vi "CRYUnflatten Analysis.vi"(11 "Unflatten Analysis":string) -> (0 "Error?":bool, 2 "Analysis":T1={"Name"="", "Harmonics"=[1.0], " Algorithm"=0, "delay"=0.0, "THD(%)"=FALSE, "Rub&Buzz"=FALSE, "Imp"=FALSE, "Imp Ref resistor"=1.0, "Y data"=0, "Y prefix"="", "Y unit"="", "Y dB ref"=1.0, "Custom Curve Names"=[], "har list items"=[""], "Envelope"=FALSE, "use custom unit"=FALSE, "autodelay ch"=0.0, "impulse"=FALSE, " start ms"=1.0, " stop ms"=1.0, "Scaling"=1, "Default Overlap "=FALSE, "Advanced View"=FALSE, "Loose Particle"=FALSE, "Use default"=FALSE, "Auto-Correlation(Stimulus)"=FALSE, "Auto-Correlation(Response)"=FALSE, "Deconvolved Response"=FALSE, "Mic Current"=FALSE, "M List Vaiues"=0, "Type"=0, "Delay Method"=3, "Apply Correction Out"=FALSE, "Apply Correction In"=FALSE, "Harmonics @ meas.frq"=FALSE, "THD Normalized(%)"=FALSE, "Total Distortion"=FALSE, "THD+Noise(%)"=FALSE, "Rub&Buzz Norm'd(%)"=FALSE, "Standard Error"=FALSE, "Confidence Limits"=FALSE, "Total Diff"=FALSE, "Total Noise"=FALSE, "Total DFD(%)"=FALSE, "Total IMD(%)"=FALSE, "Total IM"=FALSE, "Total DFD+Noise(%)"=FALSE, "Use Channel Name"=FALSE, "Waveform In"="", "Waveform Out"="", "Method"=3, "Spectral Scaling"=3, "Appliied Unit"=1, "Length Unit"=1, "Applied Units"=1, "Sens Item"=0, "Tab"=1, "Distance Unit"=0, "discard cycles"=1.0, "Weigting"="", "Averaging Time"=0.0, "Max duration"=0.0, "Min duration"=0.0, "Attack Threshold"=0.0, "Hysteresis Up"=0.0, "Fmin(Hz)"=0.0, "Fmax(Hz)"=0.0, "Freq.Resolution"=0.0, "Over-samples Res."=0.0, "Win Resolution"=0.0, "distance"=0.0, "samples"=1.0, "Overlap"=1.0, "Record Length"=1.0, "No.of FFTs"=0.0, "Hz"=1.0, "record delay"=1.0, " Std Err"=1.0, "Response"=FALSE, "Coherent Power*"=FALSE, "Stimulus"=FALSE, "Measurement Confidence"=FALSE, "Auto Spectrum(Response)*"=FALSE, "Auto Spectrum(Stimulus)*"=FALSE, "Cross Spectrum*"=FALSE, "functions"=FALSE, "Frequency Response"=FALSE, "Non-Coherent Power*"=FALSE, "Coherence (%)"=FALSE, "Non-Coherence (%)"=FALSE, "Signal-Noise Ratio (dB)"=FALSE, "Non-Coherenct Distirtion*"=FALSE, "Result Waveforms"=FALSE, "Coupling"=FALSE, "Averaging"=0, "Harmonics"=0, "Custom Curve Names"=0, "unLabel"="", "Custom Curve Names"="", "Unit"="", "Total IMD + Noise(%) "=FALSE, "ResponseMe"=1, "Intermod"=[1.0], "Diff\n"=[1.0], "Cross-Correlation"=FALSE, "IM list items"=[""], "Diff list items"=[""], "TSR Window Type"="", "Help"="", "Custom Curve IDs"=[], "Default Curve Names"=[], "Loose Particle waveform"=FALSE, "Perceptual Rub&Buzz"=FALSE, "Imp Auto Mode"=0, "Mic Auto Mode"=0, "Mic Ref resistor"=1.0, "Curve Resolution"=3, "Curve Resolution Hz"=0.0, "Polarity"=FALSE} {"Curve Resolution Hz" format="%.2f"; "Mic Ref resistor" format="%.2f"; "Diff" format="%.2f"; "Intermod" format="%.2f"; "ResponseMe" items=["Absolute", "Relative"]; "Std Err" format="%.1f"; "record delay" format="%.1f"; "Hz" format="%.1f"; "No.of FFTs" format="%.2f"; "Record Length" format="%.1f"; "Overlap" format="%.1f"; "samples" format="%.1f"; "distance" format="%.2f"; "Win Resolution" format="%.2f"; "Over-samples Res." format="%.2f"; "Freq.Resolution" format="%.2f"; "Fmax(Hz)" format="%.2f"; "Fmin(Hz)" format="%.2f"; "Hysteresis Up" format="%.2f"; "Attack Threshold" format="%.2f"; "Min duration" format="%.2f"; "Max duration" format="%.2f"; "Averaging Time" format="%.2f"; "Distance Unit" items=["Absolute", "Relative"]; "Sens Item" items=["x", "y", "z"]; "Applied Units" items=["Absolute", "Relative"]; "Length Unit" items=["Absolute", "Relative"]; "Appliied Unit" items=["Absolute", "Relative"]; "Spectral Scaling" items=["Absolute", "Relative"]; "M List Vaiues" items=["x", "y", "z"]; "Scaling" format="%.1f"; "stop ms" format="%.1f"; "start ms" format="%.1f"; "Y data" items=["dB", "Lin"]; "Y dB ref" format="%.1f"; "Imp Ref resistor" format="%.2f"; "Harmonics" format="%.2f"; "delay" format="%.2f"}, 3 "Header info":T2={"Data type"="Data            ", "Version"=1, "Dimensions"=0})   [LabVIEW 2013]
uses:
  Typedef Control/CRYAnalysis Cluster.ctl
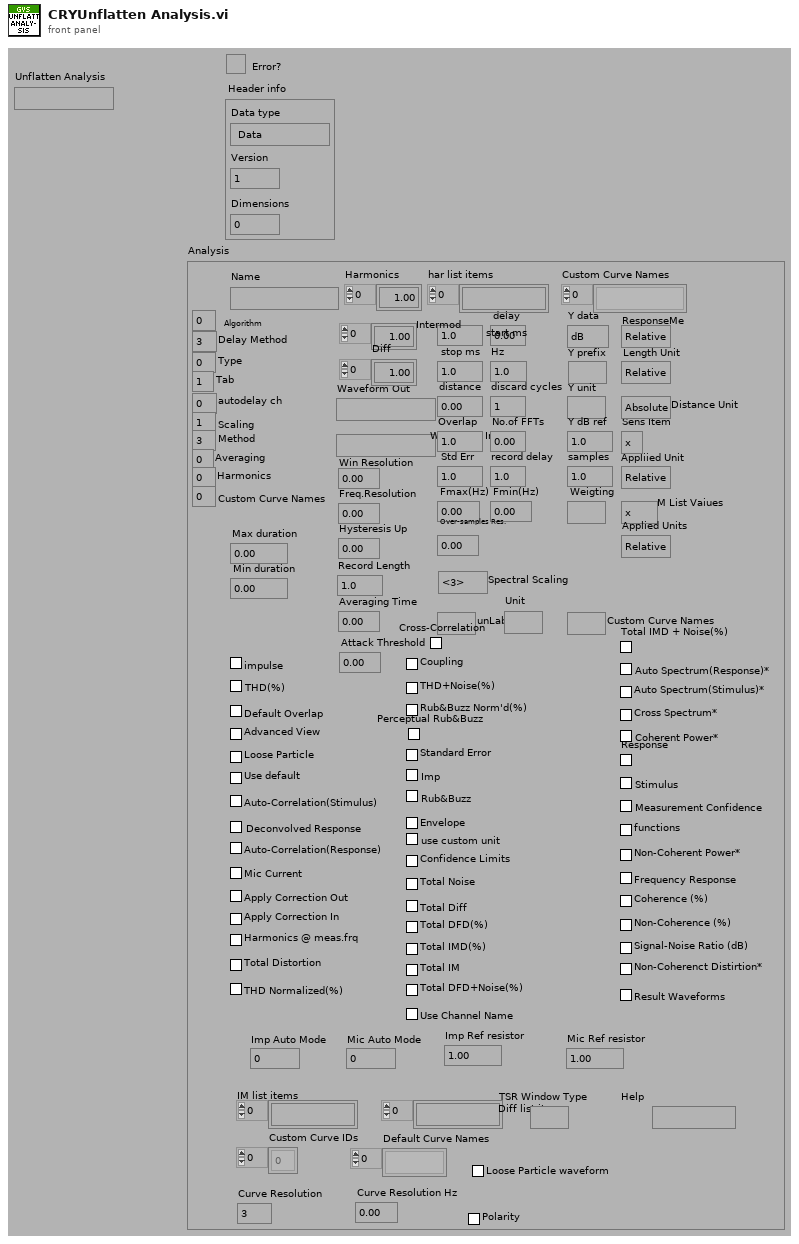
[diagram p1: front panel]
types:
  T1 = typedef "CRYAnalysis Cluster.ctl" = cluster{"Name":string, "Harmonics":dbl[], " Algorithm":u16, "delay":dbl, "THD(%)":bool, "Rub&Buzz":bool, "Imp":bool, "Imp Ref resistor":dbl, "Y data":u16, "Y prefix":string, "Y unit":string, "Y dB ref":dbl, "Custom Curve Names":string[], "har list items":string[], "Envelope":bool, "use custom unit":bool, "autodelay ch":dbl, "impulse":bool, " start ms":dbl, " stop ms":dbl, "Scaling":i32, "Default Overlap ":bool, "Advanced View":bool, "Loose Particle":bool, "Use default":bool, "Auto-Correlation(Stimulus)":bool, "Auto-Correlation(Response)":bool, "Deconvolved Response":bool, "Mic Current":bool, "M List Vaiues":u16, "Type":u16, "Delay Method":u16, "Apply Correction Out":bool, "Apply Correction In":bool, "Harmonics @ meas.frq":bool, "THD Normalized(%)":bool, "Total Distortion":bool, "THD+Noise(%)":bool, "Rub&Buzz Norm'd(%)":bool, "Standard Error":bool, "Confidence Limits":bool, "Total Diff":bool, "Total Noise":bool, "Total DFD(%)":bool, "Total IMD(%)":bool, "Total IM":bool, "Total DFD+Noise(%)":bool, "Use Channel Name":bool, "Waveform In":string, "Waveform Out":string, "Method":u16, "Spectral Scaling":u16, "Appliied Unit":u16, "Length Unit":u16, "Applied Units":u16, "Sens Item":u16, "Tab":i32, "Distance Unit":u16, "discard cycles":dbl, "Weigting":string, "Averaging Time":dbl, "Max duration":dbl, "Min duration":dbl, "Attack Threshold":dbl, "Hysteresis Up":dbl, "Fmin(Hz)":dbl, "Fmax(Hz)":dbl, "Freq.Resolution":dbl, "Over-samples Res.":dbl, "Win Resolution":dbl, "distance":dbl, "samples":dbl, "Overlap":dbl, "Record Length":dbl, "No.of FFTs":dbl, "Hz":dbl, "record delay":dbl, " Std Err":dbl, "Response":bool, "Coherent Power*":bool, "Stimulus":bool, "Measurement Confidence":bool, "Auto Spectrum(Response)*":bool, "Auto Spectrum(Stimulus)*":bool, "Cross Spectrum*":bool, "functions":bool, "Frequency Response":bool, "Non-Coherent Power*":bool, "Coherence (%)":bool, "Non-Coherence (%)":bool, "Signal-Noise Ratio (dB)":bool, "Non-Coherenct Distirtion*":bool, "Result Waveforms":bool, "Coupling":bool, "Averaging":u16, "Harmonics":i32, "Custom Curve Names":i32, "unLabel":string, "Custom Curve Names":string, "Unit":string, "Total IMD + Noise(%) ":bool, "ResponseMe":u16, "Intermod":dbl[], "Diff\n":dbl[], "Cross-Correlation":bool, "IM list items":string[], "Diff list items":string[], "TSR Window Type":string, "Help":string, "Custom Curve IDs":i32[], "Default Curve Names":string[], "Loose Particle waveform":bool, "Perceptual Rub&Buzz":bool, "Imp Auto Mode":u16, "Mic Auto Mode":u16, "Mic Ref resistor":dbl, "Curve Resolution":u16, "Curve Resolution Hz":dbl, "Polarity":bool}
  T2 = cluster{"Data type":string, "Version":u16, "Dimensions":u8}
  T3 = cluster{"Name":string, "Harmonics":dbl[], " Algorithm":u16, "delay":dbl, "THD(%)":bool, "Rub&Buzz":bool, "Imp":bool, "Imp Ref resistor":dbl, "Y data":u16, "Y prefix":string, "Y unit":string, "Y dB ref":dbl, "Custom Curve Names":string[], "har list items":string[], "Envelope":bool, "use custom unit":bool, "autodelay ch":dbl, "impulse":bool, " start ms":dbl, " stop ms":dbl, "Scaling":i32, "Default Overlap ":bool, "Advanced View":bool, "Loose Particle":bool, "Use default":bool, "Auto-Correlation(Stimulus)":bool, "Auto-Correlation(Response)":bool, "Deconvolved Response":bool, "Mic Current":bool, "M List Vaiues":u16, "Type":u16, "Delay Method":u16, "Apply Correction Out":bool, "Apply Correction In":bool, "Harmonics @ meas.frq":bool, "THD Normalized(%)":bool, "Total Distortion":bool, "THD+Noise(%)":bool, "Rub&Buzz Norm'd(%)":bool, "Standard Error":bool, "Confidence Limits":bool, "Total Diff":bool, "Total Noise":bool, "Total DFD(%)":bool, "Total IMD(%)":bool, "Total IM":bool, "Total DFD+Noise(%)":bool, "Use Channel Name":bool, "Waveform In":string, "Waveform Out":string, "Method":u16, "Spectral Scaling":u16, "Appliied Unit":u16, "Length Unit":u16, "Applied Units":u16, "Sens Item":u16, "Tab":i32, "Distance Unit":u16, "discard cycles":dbl, "Weigting":string, "Averaging Time":dbl, "Max duration":dbl, "Min duration":dbl, "Attack Threshold":dbl, "Hysteresis Up":dbl, "Fmin(Hz)":dbl, "Fmax(Hz)":dbl, "Freq.Resolution":dbl, "Over-samples Res.":dbl, "Win Resolution":dbl, "distance":dbl, "samples":dbl, "Overlap":dbl, "Record Length":dbl, "No.of FFTs":dbl, "Hz":dbl, "record delay":dbl, " Std Err":dbl, "Response":bool, "Coherent Power*":bool, "Stimulus":bool, "Measurement Confidence":bool, "Auto Spectrum(Response)*":bool, "Auto Spectrum(Stimulus)*":bool, "Cross Spectrum*":bool, "functions":bool, "Frequency Response":bool, "Non-Coherent Power*":bool, "Coherence (%)":bool, "Non-Coherence (%)":bool, "Signal-Noise Ratio (dB)":bool, "Non-Coherenct Distirtion*":bool, "Result Waveforms":bool, "Coupling":bool, "Averaging":u16, "Harmonics":i32, "Custom Curve Names":i32, "unLabel":string, "Custom Curve Names":string, "Unit":string, "Total IMD + Noise(%) ":bool, "ResponseMe":u16, "Intermod":dbl[], "Diff\n":dbl[], "Cross-Correlation":bool, "IM list items":string[], "Diff list items":string[], "TSR Window Type":string, "Help":string, "Custom Curve IDs":i32[], "Default Curve Names":string[], "Loose Particle waveform":bool, "Perceptual Rub&Buzz":bool, "Imp Auto Mode":u16, "Mic Auto Mode":u16, "Mic Ref resistor":dbl, "Curve Resolution":u16, "Curve Resolution Hz":dbl, "Polarity":bool}
  T4 = cluster{"Name":string, "Harmonics":dbl[], " Algorithm":u16, "delay":dbl, "THD(%)":bool, "Rub&Buzz":bool, "Imp":bool, "Imp Ref resistor":dbl, "Y data":u16, "Y prefix":string, "Y unit":string, "Y dB ref":dbl, "Custom Curve Names":string[], "har list items":string[], "Envelope":bool, "use custom unit":bool, "autodelay ch":dbl, "impulse":bool, " start ms":dbl, " stop ms":dbl, "Scaling":i32, "Default Overlap ":bool, "Advanced View":bool, "Loose Particle":bool, "Use default":bool, "Auto-Correlation(Stimulus)":bool, "Auto-Correlation(Response)":bool, "Deconvolved Response":bool, "Mic Current":bool, "M List Vaiues":u16, "Type":u16, "Delay Method":u16, "Apply Correction Out":bool, "Apply Correction In":bool, "Harmonics @ meas.frq":bool, "THD Normalized(%)":bool, "Total Distortion":bool, "THD+Noise(%)":bool, "Rub&Buzz Norm'd(%)":bool, "Standard Error":bool, "Confidence Limits":bool, "Total Diff":bool, "Total Noise":bool, "Total DFD(%)":bool, "Total IMD(%)":bool, "Total IM":bool, "Total DFD+Noise(%)":bool, "Use Channel Name":bool, "Waveform In":string, "Waveform Out":string, "Method":u16, "Spectral Scaling":u16, "Appliied Unit":u16, "Length Unit":u16, "Applied Units":u16, "Sens Item":u16, "Tab":i32, "Distance Unit":u16, "discard cycles":dbl, "Weigting":string, "Averaging Time":dbl, "Max duration":dbl, "Min duration":dbl, "Attack Threshold":dbl, "Hysteresis Up":dbl, "Fmin(Hz)":dbl, "Fmax(Hz)":dbl, "Freq.Resolution":dbl, "Over-samples Res.":dbl, "Win Resolution":dbl, "distance":dbl, "samples":dbl, "Overlap":dbl, "Record Length":dbl, "No.of FFTs":dbl, "Hz":dbl, "record delay":dbl, " Std Err":dbl, "Response":bool, "Coherent Power*":bool, "Stimulus":bool, "Measurement Confidence":bool, "Auto Spectrum(Response)*":bool, "Auto Spectrum(Stimulus)*":bool, "Cross Spectrum*":bool, "functions":bool, "Frequency Response":bool, "Non-Coherent Power*":bool, "Coherence (%)":bool, "Non-Coherence (%)":bool, "Signal-Noise Ratio (dB)":bool, "Non-Coherenct Distirtion*":bool, "Result Waveforms":bool, "Coupling":bool, "Averaging":u16, "Harmonics":i32, "Custom Curve Names":i32, "unLabel":string, "Custom Curve Names":string, "Unit":string, "Total IMD + Noise(%) ":bool, "ResponseMe":u16, "Intermod":dbl[], "Diff\n":dbl[], "Cross-Correlation":bool, "IM list items":string[], "Diff list items":string[], "TSR Window Type":string, "Help":string, "Custom Curve IDs":i32[], "Default Curve Names":string[], "Loose Particle waveform":bool, "Perceptual Rub&Buzz":bool, "Imp Auto Mode":u16, "Mic Auto Mode":u16, "Mic Ref resistor":dbl, "Curve Resolution":u16, "Curve Resolution Hz":dbl}
  T5 = cluster{"Name":string, "Harmonics":dbl[], " Algorithm":u16, "delay":dbl, "THD(%)":bool, "Rub&Buzz":bool, "Imp":bool, "Imp Ref resistor":dbl, "Y data":u16, "Y prefix":string, "Y unit":string, "Y dB ref":dbl, "Custom Curve Names":string[], "har list items":string[], "Envelope":bool, "use custom unit":bool, "autodelay ch":dbl, "impulse":bool, " start ms":dbl, " stop ms":dbl, "Scaling":i32, "Default Overlap ":bool, "Advanced View":bool, "Loose Particle":bool, "Use default":bool, "Auto-Correlation(Stimulus)":bool, "Auto-Correlation(Response)":bool, "Deconvolved Response":bool, "Mic Current":bool, "M List Vaiues":u16, "Type":u16, "Delay Method":u16, "Apply Correction Out":bool, "Apply Correction In":bool, "Harmonics @ meas.frq":bool, "THD Normalized(%)":bool, "Total Distortion":bool, "THD+Noise(%)":bool, "Rub&Buzz Norm'd(%)":bool, "Standard Error":bool, "Confidence Limits":bool, "Total Diff":bool, "Total Noise":bool, "Total DFD(%)":bool, "Total IMD(%)":bool, "Total IM":bool, "Total DFD+Noise(%)":bool, "Use Channel Name":bool, "Waveform In":string, "Waveform Out":string, "Method":u16, "Spectral Scaling":u16, "Appliied Unit":u16, "Length Unit":u16, "Applied Units":u16, "Sens Item":u16, "Tab":i32, "Distance Unit":u16, "discard cycles":dbl, "Weigting":string, "Averaging Time":dbl, "Max duration":dbl, "Min duration":dbl, "Attack Threshold":dbl, "Hysteresis Up":dbl, "Fmin(Hz)":dbl, "Fmax(Hz)":dbl, "Freq.Resolution":dbl, "Over-samples Res.":dbl, "Win Resolution":dbl, "distance":dbl, "samples":dbl, "Overlap":dbl, "Record Length":dbl, "No.of FFTs":dbl, "Hz":dbl, "record delay":dbl, " Std Err":dbl, "Response":bool, "Coherent Power*":bool, "Stimulus":bool, "Measurement Confidence":bool, "Auto Spectrum(Response)*":bool, "Auto Spectrum(Stimulus)*":bool, "Cross Spectrum*":bool, "functions":bool, "Frequency Response":bool, "Non-Coherent Power*":bool, "Coherence (%)":bool, "Non-Coherence (%)":bool, "Signal-Noise Ratio (dB)":bool, "Non-Coherenct Distirtion*":bool, "Result Waveforms":bool, "Coupling":bool, "Averaging":u16, "Harmonics":i32, "Custom Curve Names":i32, "unLabel":string, "Custom Curve Names":string, "Unit":string, "Total IMD + Noise(%) ":bool, "ResponseMe":u16, "Intermod":dbl[], "Diff\n":dbl[], "Cross-Correlation":bool, "IM list items":string[], "Diff list items":string[], "TSR Window Type":string, "Help":string, "Custom Curve IDs":i32[], "Default Curve Names":string[], "Loose Particle waveform":bool, "Perceptual Rub&Buzz":bool, "Imp Auto Mode":u16, "Mic Auto Mode":u16, "Mic Ref resistor":dbl}
  T6 = cluster{"Name":string, "Harmonics":dbl[], " Algorithm":u16, "delay":dbl, "THD(%)":bool, "Rub&Buzz":bool, "Imp":bool, "Ref resistor":dbl, "Y data":u16, "Y prefix":string, "Y unit":string, "Y dB ref":dbl, "Custom Curve Names":string[], "har list items":string[], "Envelope":bool, "use custom unit":bool, "autodelay ch":dbl, "impulse":bool, " start ms":dbl, " stop ms":dbl, "Scaling":i32, "Default Overlap ":bool, "Advanced View":bool, "Loose Particle":bool, "Use default":bool, "Auto-Correlation(Stimulus)":bool, "Auto-Correlation(Response)":bool, "Deconvolved Response":bool, "Mic Current":bool, "M List Vaiues":u16, "Type":u16, "Delay Method":u16, "Apply Correction Out":bool, "Apply Correction In":bool, "Harmonics @ meas.frq":bool, "THD Normalized(%)":bool, "Total Distortion":bool, "THD+Noise(%)":bool, "Rub&Buzz Norm'd(%)":bool, "Standard Error":bool, "Confidence Limits":bool, "Total Diff":bool, "Total Noise":bool, "Total DFD(%)":bool, "Total IMD(%)":bool, "Total IM":bool, "Total DFD+Noise(%)":bool, "Use Channel Name":bool, "Waveform In":string, "Waveform Out":string, "Method":u16, "Spectral Scaling":u16, "Appliied Unit":u16, "Length Unit":u16, "Applied Units":u16, "Sens Item":u16, "Tab":i32, "Distance Unit":u16, "discard cycles":dbl, "Weigting":string, "Averaging Time":dbl, "Max duration":dbl, "Min duration":dbl, "Attack Threshold":dbl, "Hysteresis Up":dbl, "Fmin(Hz)":dbl, "Fmax(Hz)":dbl, "Freq.Resolution":dbl, "Over-samples Res.":dbl, "Win Resolution":dbl, "distance":dbl, "samples":dbl, "Overlap":dbl, "Record Length":dbl, "No.of FFTs":dbl, "Hz":dbl, "record delay":dbl, " Std Err":dbl, "Response":bool, "Coherent Power*":bool, "Stimulus":bool, "Measurement Confidence":bool, "Auto Spectrum(Response)*":bool, "Auto Spectrum(Stimulus)*":bool, "Cross Spectrum*":bool, "functions":bool, "Frequency Response":bool, "Non-Coherent Power*":bool, "Coherence (%)":bool, "Non-Coherence (%)":bool, "Signal-Noise Ratio (dB)":bool, "Non-Coherenct Distirtion*":bool, "Result Waveforms":bool, "Coupling":bool, "Averaging":u16, "Harmonics":i32, "Custom Curve Names":i32, "unLabel":string, "Custom Curve Names":string, "Unit":string, "Total IMD + Noise(%) ":bool, "ResponseMe":u16, "Intermod":dbl[], "Diff\n":dbl[], "Cross-Correlation":bool, "IM list items":string[], "Diff list items":string[], "TSR Window Type":string, "Help":string, "Custom Curve IDs":i32[], "Default Curve Names":string[], "Loose Particle waveform":bool, "Perceptual Rub&Buzz":bool, "Imp Auto Mode":u16}
  T7 = cluster{"Name":string, "Harmonics":dbl[], " Algorithm":u16, "delay":dbl, "THD(%)":bool, "Rub&Buzz":bool, "Imp":bool, "Ref resistor":dbl, "Y data":u16, "Y prefix":string, "Y unit":string, "Y dB ref":dbl, "Custom Curve Names":string[], "har list items":string[], "AC/DC":bool, "Envelope":bool, "use custom unit":bool, "autodelay ch":dbl, "impulse":bool, " start ms":dbl, " stop ms":dbl, "Scaling":i32, "Default Overlap ":bool, "Advanced View":bool, "Loose Particle":bool, "Use default":bool, "Auto-Correlation(Stimulus)":bool, "Auto-Correlation(Response)":bool, "Deconvolved Response":bool, "DC Connect Measurement":bool, "M List Vaiues":u16, "Type":u16, "Delay Method":u16, "Apply Correction Out":bool, "Apply Correction In":bool, "Harmonics @ meas.frq":bool, "THD Normalized(%)":bool, "Total Distortion":bool, "THD+Noise(%)":bool, "Rub&Buzz Norm'd(%)":bool, "Standard Error":bool, "Confidence Limits":bool, "Total Diff":bool, "Total Noise":bool, "Total DFD(%)":bool, "Total IMD(%)":bool, "Total IM":bool, "Total DFD+Noise(%)":bool, "Use Channel Name":bool, "Waveform In":string, "Waveform Out":string, "Method":u16, "Spectral Scaling":u16, "Appliied Unit":u16, "Length Unit":u16, "Applied Units":u16, "Sens Item":u16, "Tab":i32, "Distance Unit":u16, "discard cycles":dbl, "Weigting":string, "Averaging Time":dbl, "Max duration":dbl, "Min duration":dbl, "Attack Threshold":dbl, "Hysteresis Up":dbl, "Fmin(Hz)":dbl, "Fmax(Hz)":dbl, "Freq.Resolution":dbl, "Over-samples Res.":dbl, "Win Resolution":dbl, "distance":dbl, "samples":dbl, "Overlap":dbl, "Record Length":dbl, "No.of FFTs":dbl, "Hz":dbl, "record delay":dbl, " Std Err":dbl, "Response":bool, "Coherent Power*":bool, "Stimulus":bool, "Measurement Confidence":bool, "Auto Spectrum(Response)*":bool, "Auto Spectrum(Stimulus)*":bool, "Cross Spectrum*":bool, "functions":bool, "Frequency Response":bool, "Non-Coherent Power*":bool, "Coherence (%)":bool, "Non-Coherence (%)":bool, "Signal-Noise Ratio (dB)":bool, "Non-Coherenct Distirtion*":bool, "Result Waveforms":bool, "Coupling":bool, "Averaging":u16, "AC/DC 2":bool, "Harmonics":i32, "Custom Curve Names":i32, "unLabel":string, "Custom Curve Names":string, "Unit":string, "Total IMD + Noise(%) ":bool, "ResponseMe":u16, "Intermod":dbl[], "Diff\n":dbl[], "Cross-Correlation":bool, "IM list items":string[], "Diff list items":string[], "TSR Window Type":string, "Help":string, "Custom Curve IDs":i32[], "Default Curve Names":string[], "Loose Particle waveform":bool, "Perceptual Rub&Buzz":bool}
  T8 = cluster{"Name":string, "Harmonics":dbl[], " Algorithm":u16, "delay":dbl, "THD(%)":bool, "Rub&Buzz":bool, "Imp":bool, "Ref resistor":dbl, "Y data":u16, "Y prefix":string, "Y unit":string, "Y dB ref":dbl, "Custom Curve Names":string[], "har list items":string[], "AC/DC":bool, "Envelope":bool, "use custom unit":bool, "autodelay ch":dbl, "impulse":bool, " start ms":dbl, " stop ms":dbl, "Scaling":i32, "Default Overlap ":bool, "Advanced View":bool, "Loose Particle":bool, "Use default":bool, "Auto-Correlation(Stimulus)":bool, "Auto-Correlation(Response)":bool, "Deconvolved Response":bool, "DC Connect Measurement":bool, "M List Vaiues":u16, "Type":u16, "Delay Method":u16, "Apply Correction Out":bool, "Apply Correction In":bool, "Harmonics @ meas.frq":bool, "THD Normalized(%)":bool, "Total Distortion":bool, "THD+Noise(%)":bool, "Rub&Buzz Norm'd(%)":bool, "Standard Error":bool, "Confidence Limits":bool, "Total Diff":bool, "Total Noise":bool, "Total DFD(%)":bool, "Total IMD(%)":bool, "Total IM":bool, "Total DFD+Noise(%)":bool, "Use Channel Name":bool, "Waveform In":string, "Waveform Out":string, "Method":u16, "Spectral Scaling":u16, "Appliied Unit":u16, "Length Unit":u16, "Applied Units":u16, "Sens Item":u16, "Tab":i32, "Distance Unit":u16, "discard cycles":dbl, "Weigting":string, "Averaging Time":dbl, "Max duration":dbl, "Min duration":dbl, "Attack Threshold":dbl, "Hysteresis Up":dbl, "Fmin(Hz)":dbl, "Fmax(Hz)":dbl, "Freq.Resolution":dbl, "Over-samples Res.":dbl, "Win Resolution":dbl, "distance":dbl, "samples":dbl, "Overlap":dbl, "Record Length":dbl, "No.of FFTs":dbl, "Hz":dbl, "record delay":dbl, " Std Err":dbl, "Response":bool, "Coherent Power*":bool, "Stimulus":bool, "Measurement Confidence":bool, "Auto Spectrum(Response)*":bool, "Auto Spectrum(Stimulus)*":bool, "Cross Spectrum*":bool, "functions":bool, "Frequency Response":bool, "Non-Coherent Power*":bool, "Coherence (%)":bool, "Non-Coherence (%)":bool, "Signal-Noise Ratio (dB)":bool, "Non-Coherenct Distirtion*":bool, "Result Waveforms":bool, "Coupling":bool, "Averaging":u16, "AC/DC 2":bool, "Harmonics":i32, "Custom Curve Names":i32, "unLabel":string, "Custom Curve Names":string, "Unit":string, "Total IMD + Noise(%) ":bool, "ResponseMe":u16, "Intermod":dbl[], "Diff\n":dbl[], "Cross-Correlation":bool, "IM list items":string[], "Diff list items":string[], "TSR Window Type":string, "Help":string, "Custom Curve IDs":i32[], "Default Curve Names":string[]}
  T9 = cluster{"Name":string, "Harmonics":dbl[], " Algorithm":u16, "delay":dbl, "THD(%)":bool, "Rub&Buzz":bool, "Imp":bool, "Ref resistor":dbl, "Y data":u16, "Y prefix":string, "Y unit":string, "Y dB ref":dbl, "Custom Curve Names":string[], "har list items":string[], "AC/DC":bool, "Envelope":bool, "use custom unit":bool, "autodelay ch":dbl, "impulse":bool, " start ms":dbl, " stop ms":dbl, "Scaling":i32, "Default Overlap ":bool, "Advanced View":bool, "Loose Particle":bool, "Use default":bool, "Auto-Correlation(Stimulus)":bool, "Auto-Correlation(Response)":bool, "Deconvolved Response":bool, "DC Connect Measurement":bool, "M List Vaiues":u16, "Type":u16, "Delay Method":u16, "Apply Correction Out":bool, "Apply Correction In":bool, "Harmonics @ meas.frq":bool, "THD Normalized(%)":bool, "Total Distortion":bool, "THD+Noise(%)":bool, "Rub&Buzz Norm'd(%)":bool, "Standard Error":bool, "Confidence Limits":bool, "Total Diff":bool, "Total Noise":bool, "Total DFD(%)":bool, "Total IMD(%)":bool, "Total IM":bool, "Total DFD+Noise(%)":bool, "Use Channel Name":bool, "Waveform In":string, "Waveform Out":string, "Method":u16, "Spectral Scaling":u16, "Appliied Unit":u16, "Length Unit":u16, "Applied Units":u16, "Sens Item":u16, "Tab":i32, "Distance Unit":u16, "discard cycles":dbl, "Weigting":string, "Averaging Time":dbl, "Max duration":dbl, "Min duration":dbl, "Attack Threshold":dbl, "Hysteresis Up":dbl, "Fmin(Hz)":dbl, "Fmax(Hz)":dbl, "Freq.Resolution":dbl, "Over-samples Res.":dbl, "Win Resolution":dbl, "distance":dbl, "samples":dbl, "Overlap":dbl, "Record Length":dbl, "No.of FFTs":dbl, "Hz":dbl, "record delay":dbl, " Std Err":dbl, "Response":bool, "Coherent Power*":bool, "Stimulus":bool, "Measurement Confidence":bool, "Auto Spectrum(Response)*":bool, "Auto Spectrum(Stimulus)*":bool, "Cross Spectrum*":bool, "functions":bool, "Frequency Response":bool, "Non-Coherent Power*":bool, "Coherence (%)":bool, "Non-Coherence (%)":bool, "Signal-Noise Ratio (dB)":bool, "Non-Coherenct Distirtion*":bool, "Result Waveforms":bool, "Coupling":bool, "Averaging":u16, "AC/DC 2":bool, "Harmonics":i32, "Custom Curve Names":i32, "unLabel":string, "Custom Curve Names":string, "Unit":string, "Total IMD + Noise(%) ":bool, "ResponseMe":u16, "Intermod":dbl[], "Diff\n":dbl[], "Cross-Correlation":bool, "IM list items":string[], "Diff list items":string[], "TSR Window Type":string, "Help":string}
  T10 = cluster{"Name":string, "Harmonics":dbl[], " Algorithm":u16, "delay":dbl, "THD(%)":bool, "Rub&Buzz":bool, "Imp":bool, "Ref resistor":dbl, "Y data":u16, "Y prefix":string, "Y unit":string, "Y dB ref":dbl, "Curves generated":string[], "har list items":string[], "AC/DC":bool, "Envelope":bool, "use custom unit":bool, "autodelay ch":dbl, "impulse":bool, " start ms":dbl, " stop ms":dbl, "Scaling":i32, "Default Overlap ":bool, "Advanced View":bool, "Loose Particle":bool, "Use default":bool, "Auto-Correlation(Stimulus)":bool, "Auto-Correlation(Response)":bool, "Deconvolved Response":bool, "DC Connect Measurement":bool, "M List Vaiues":u16, "Type":u16, "Delay Method":u16, "Apply Correction Out":bool, "Apply Correction In":bool, "Harmonics @ meas.frq":bool, "THD Normalized(%)":bool, "Total Distortion":bool, "THD+Noise(%)":bool, "Rub&Buzz Norm'd(%)":bool, "Standard Error":bool, "Confidence Limits":bool, "Total Diff":bool, "Total Noise":bool, "Total DFD(%)":bool, "Total IMD(%)":bool, "Total IM":bool, "Total DFD+Noise(%)":bool, "Use Channel Name":bool, "Waveform In":string, "Waveform Out":string, "Method":u16, "Spectral Scaling":u16, "Appliied Unit":u16, "Length Unit":u16, "Applied Units":u16, "Sens Item":u16, "Tab":i32, "Distance Unit":u16, "discard cycles":dbl, "Weigting":string, "Averaging Time":dbl, "Max duration":dbl, "Min duration":dbl, "Attack Threshold":dbl, "Hysteresis Up":dbl, "Fmin(Hz)":dbl, "Fmax(Hz)":dbl, "Freq.Resolution":dbl, "Over-samples Res.":dbl, "Win Resolution":dbl, "distance":dbl, "samples":dbl, "Overlap":dbl, "Record Length":dbl, "No.of FFTs":dbl, "Hz":dbl, "record delay":dbl, " Std Err":dbl, "Response":bool, "Coherent Power*":bool, "Stimulus":bool, "Measurement Confidence":bool, "Auto Spectrum(Response)*":bool, "Auto Spectrum(Stimulus)*":bool, "Cross Spectrum*":bool, "functions":bool, "Frequency Response":bool, "Non-Coherent Power*":bool, "Coherence (%)":bool, "Non-Coherence (%)":bool, "Signal-Noise Ratio (dB)":bool, "Non-Coherenct Distirtion*":bool, "Result Waveforms":bool, "Coupling":bool, "Averaging":u16, "AC/DC 2":bool, "Harmonics":i32, "Custom Curve Names":i32, "unLabel":string, "Custom Curve Names":string, "Unit":string, "Total IMD + Noise(%) ":bool, "ResponseMe":u16, "Intermod":dbl[], "Diff\n":dbl[], "Cross-Correlation":bool, "IM list items":string[], "Diff list items":string[], "TSR Window Type":string}
  T11 = cluster{"Name":string, "Harmonics":dbl[], " Algorithm":u16, "delay":dbl, "THD(%)":bool, "Rub&Buzz":bool, "Imp":bool, "Ref resistor":dbl, "Y data":u16, "Y prefix":string, "Y unit":string, "Y dB ref":dbl, "Custom Curve Names":string[], "har list items":string[], "AC/DC":bool, "Envelope":bool, "use custom unit":bool, "autodelay ch":dbl, "impulse":bool, " start ms":dbl, " stop ms":dbl, "Scaling":i32, "Default Overlap ":bool, "Advanced View":bool, "Loose Particle":bool, "Use default":bool, "Auto-Correlation(Stimulus)":bool, "Auto-Correlation(Response)":bool, "Deconvolved Response":bool, "DC Connect Measurement":bool, "M List Vaiues":u16, "Type":u16, "Delay Method":u16, "Apply Correction Out":bool, "Apply Correction In":bool, "Harmonics @ meas.frq":bool, "THD Normalized(%)":bool, "Total Distortion":bool, "THD+Noise(%)":bool, "Rub&Buzz Norm'd(%)":bool, "Standard Error":bool, "Confidence Limits":bool, "Total Diff":bool, "Total Noise":bool, "Total DFD(%)":bool, "Total IMD(%)":bool, "Total IM":bool, "Total DFD+Noise(%)":bool, "Use Channel Name":bool, "Waveform In":string, "Waveform Out":string, "Method":u16, "Spectral Scaling":u16, "Appliied Unit":u16, "Length Unit":u16, "Applied Units":u16, "Sens Item":u16, "Tab":i32, "Distance Unit":u16, "discard cycles":dbl, "Weigting":string, "Averaging Time":dbl, "Max duration":dbl, "Min duration":dbl, "Attack Threshold":dbl, "Hysteresis Up":dbl, "Fmin(Hz)":dbl, "Fmax(Hz)":dbl, "Freq.Resolution":dbl, "Over-samples Res.":dbl, "Win Resolution":dbl, "distance":dbl, "samples":dbl, "Overlap":dbl, "Record Length":dbl, "No.of FFTs":dbl, "Hz":dbl, "record delay":dbl, " Std Err":dbl, "Response":bool, "Coherent Power*":bool, "Stimulus":bool, "Measurement Confidence":bool, "Auto Spectrum(Response)*":bool, "Auto Spectrum(Stimulus)*":bool, "Cross Spectrum*":bool, "functions":bool, "Frequency Response":bool, "Non-Coherent Power*":bool, "Coherence (%)":bool, "Non-Coherence (%)":bool, "Signal-Noise Ratio (dB)":bool, "Non-Coherenct Distirtion*":bool, "Result Waveforms":bool, "Coupling":bool, "Averaging":u16, "AC/DC 2":bool, "Harmonics":i32, "Custom Curve Names":i32, "unLabel":string, "Custom Curve Names":string, "Unit":string, "Total IMD + Noise(%) ":bool, "ResponseMe":u16, "Intermod":dbl[], "Diff\n":dbl[], "Cross-Correlation":bool, "IM list items":string[], "Diff list items":string[], "TSR Window Type":string, "Help":string, "Custom Curve IDs":i32[], "Default Curve Names":string[], "Loose Particle waveform":bool}
  T12 = cluster{"Name":string, "Harmonics":dbl[], " Algorithm":u16, "delay":dbl, "THD(%)":bool, "Rub&Buzz":bool, "Imp":bool, "Ref resistor":dbl, "Y data":u16, "Y prefix":string, "Y unit":string, "Y dB ref":dbl, "Curves generated":string[], "har list items":string[], "AC/DC":bool, "Envelope":bool, "use custom unit":bool, "autodelay ch":dbl, "impulse":bool, " start ms":dbl, " stop ms":dbl, "Scaling":i32, "Default Overlap ":bool, "Advanced View":bool, "Loose Particle":bool, "Use default":bool, "Auto-Correlation(Stimulus)":bool, "Auto-Correlation(Response)":bool, "Deconvolved Response":bool, "DC Connect Measurement":bool, "M List Vaiues":u16, "Type":u16, "Delay Method":u16, "Apply Correction Out":bool, "Apply Correction In":bool, "Harmonics @ meas.frq":bool, "THD Normalized(%)":bool, "Total Distortion":bool, "THD+Noise(%)":bool, "Rub&Buzz Norm'd(%)":bool, "Standard Error":bool, "Confidence Limits":bool, "Total Diff":bool, "Total Noise":bool, "Total DFD(%)":bool, "Total IMD(%)":bool, "Total IM":bool, "Total DFD+Noise(%)":bool, "Use Channel Name":bool, "Waveform In":string, "Waveform Out":string, "Method":u16, "Spectral Scaling":u16, "Appliied Unit":u16, "Length Unit":u16, "Applied Units":u16, "Sens Item":u16, "Tab":i32, "Ring":u16, "discard cycles":dbl, "Weigting":string, "Averaging Time":dbl, "Max duration":dbl, "Min duration":dbl, "Attack Threshold":dbl, "Hysteresis Up":dbl, "Fmin(Hz)":dbl, "Fmax(Hz)":dbl, "Freq.Resolution":dbl, "Over-samples Res.":dbl, "Win Resolution":dbl, "distance":dbl, "samples":dbl, "Overlap":dbl, "Record Length":dbl, "No.of FFTs":dbl, "Hz":dbl, "record delay":dbl, " Std Err":dbl, "Response":bool, "Coherent Power*":bool, "Stimulus":bool, "Measurement Confidence":bool, "Auto Spectrum(Response)*":bool, "Auto Spectrum(Stimulus)*":bool, "Cross Spectrum*":bool, "functions":bool, "Frequency Response":bool, "Non-Coherent Power*":bool, "Coherence (%)":bool, "Non-Coherence (%)":bool, "Signal-Noise Ratio (dB)":bool, "Non-Coherenct Dustirtion*":bool, "Result Waveforms":bool, "Coupling":bool, "Averaging":u16, "AC/DC 2":bool, "Harmonics":i32, "Custom Curve Names":i32, "unLabel":string, "Custom Curve Names":string, "Unit":string, "Total IMD + Noise(%) ":bool, "ResponseMe":u16, "Orders 2":dbl[], "Orders1\n":dbl[], "Cross-Correlation":bool, "IM list items":string[], "Diff list items":string[]}
  T13 = cluster{"unsigned byte array[0]":u8, "unsigned byte array[1]":u8, "unsigned byte array[2]":u8}
  T14 = cluster{"substring":string, u16, "unsigned byte array[2]":u8}
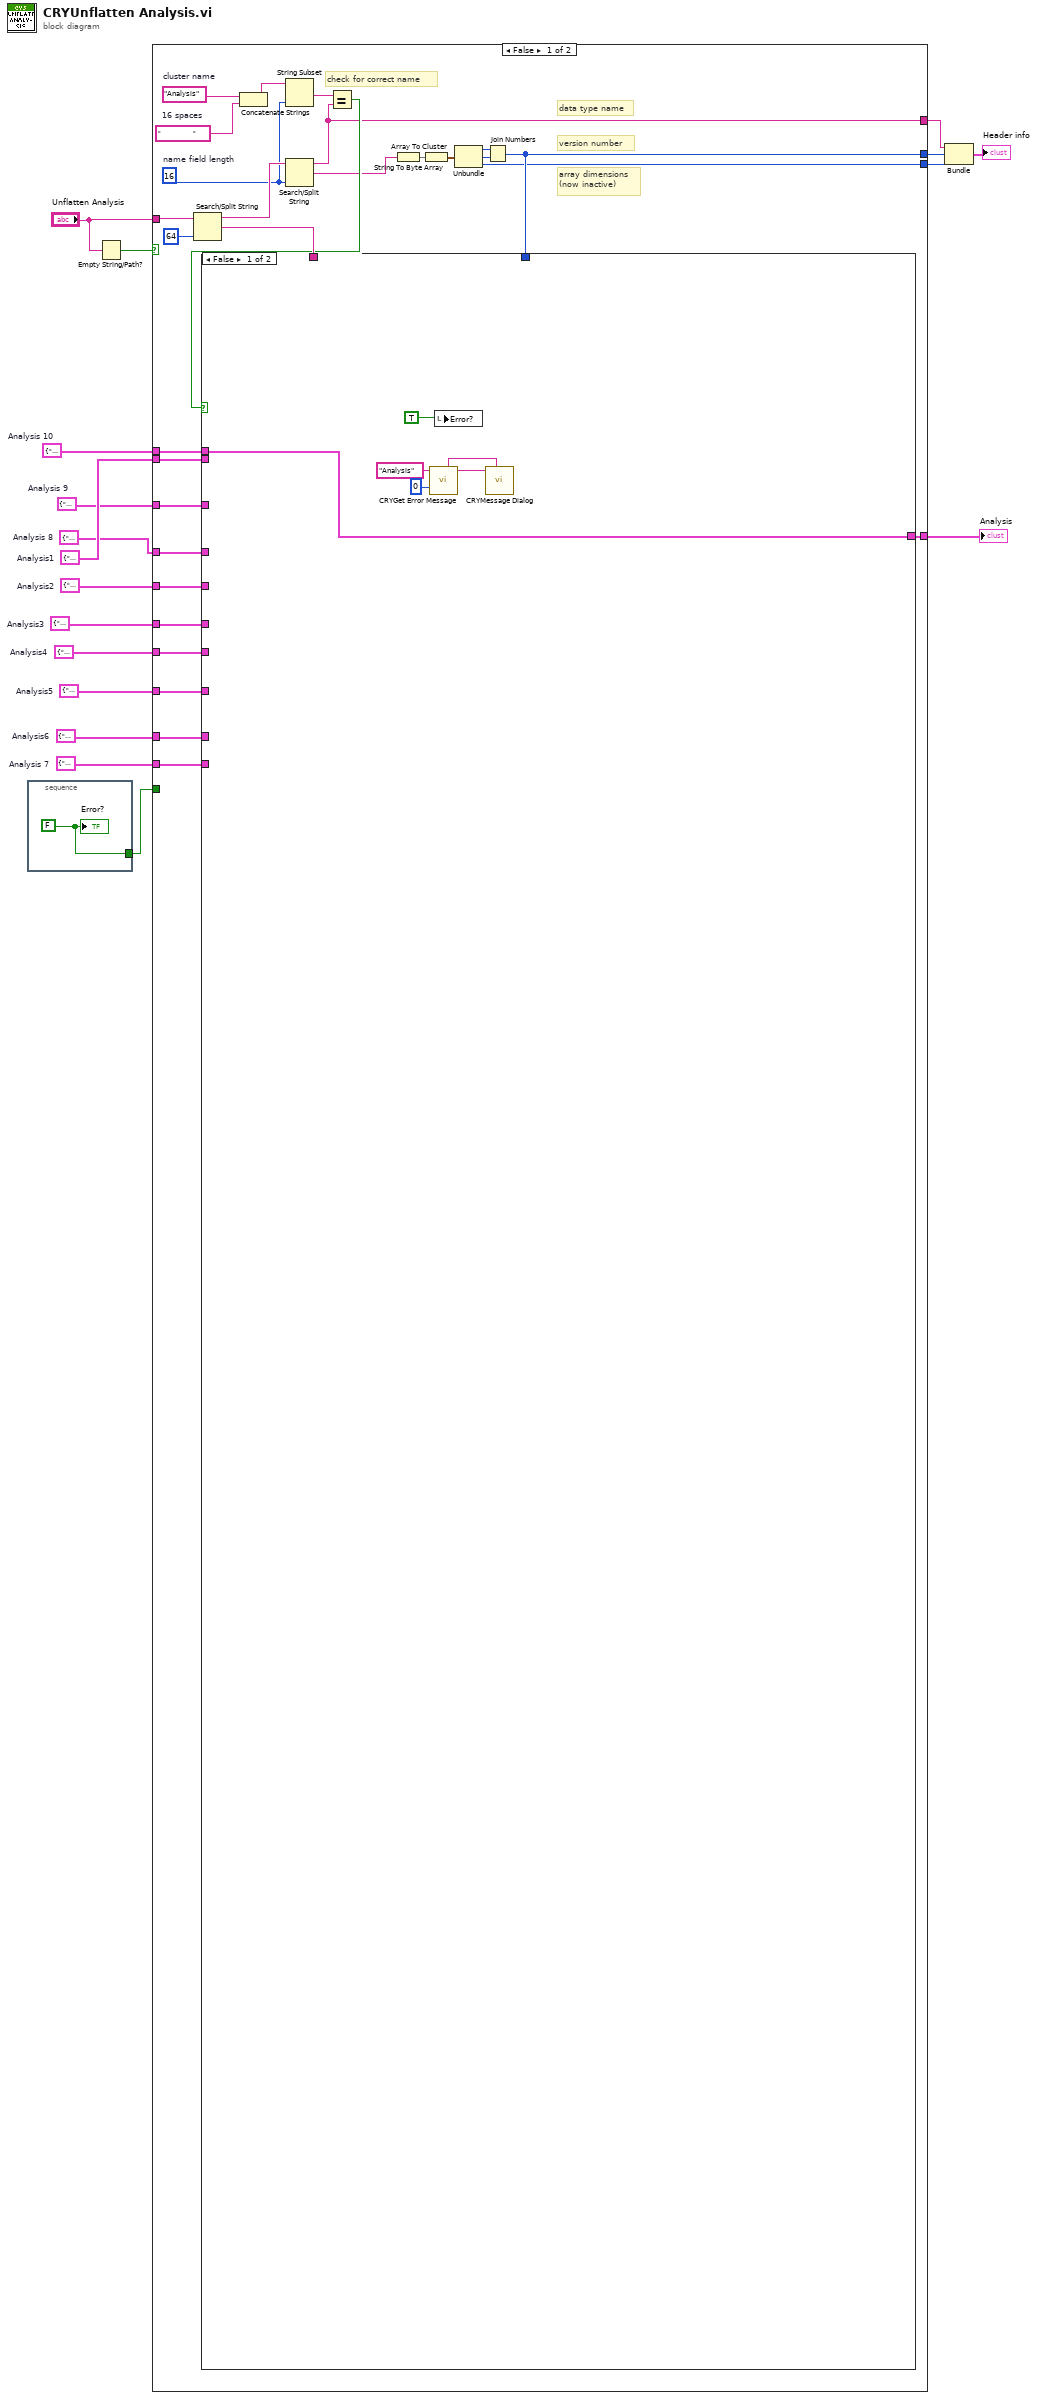
[diagram p0: block diagram]
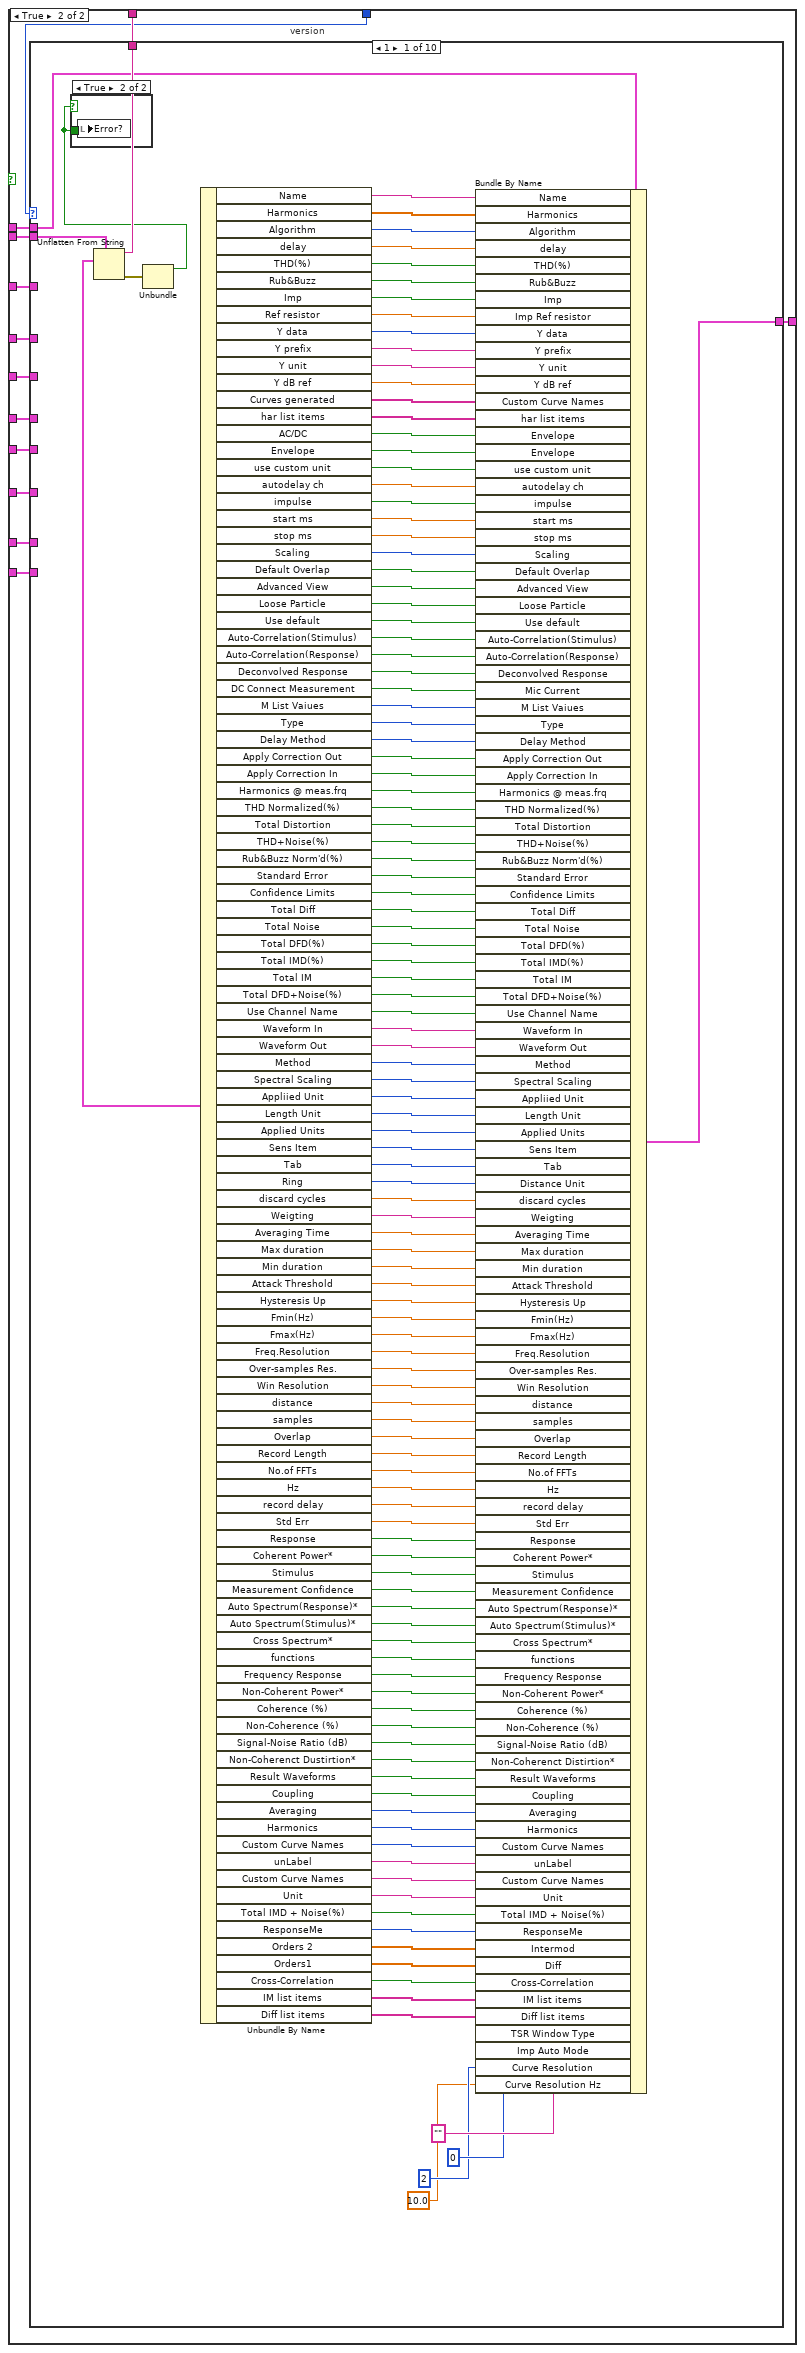
[diagram p2: hidden frame]
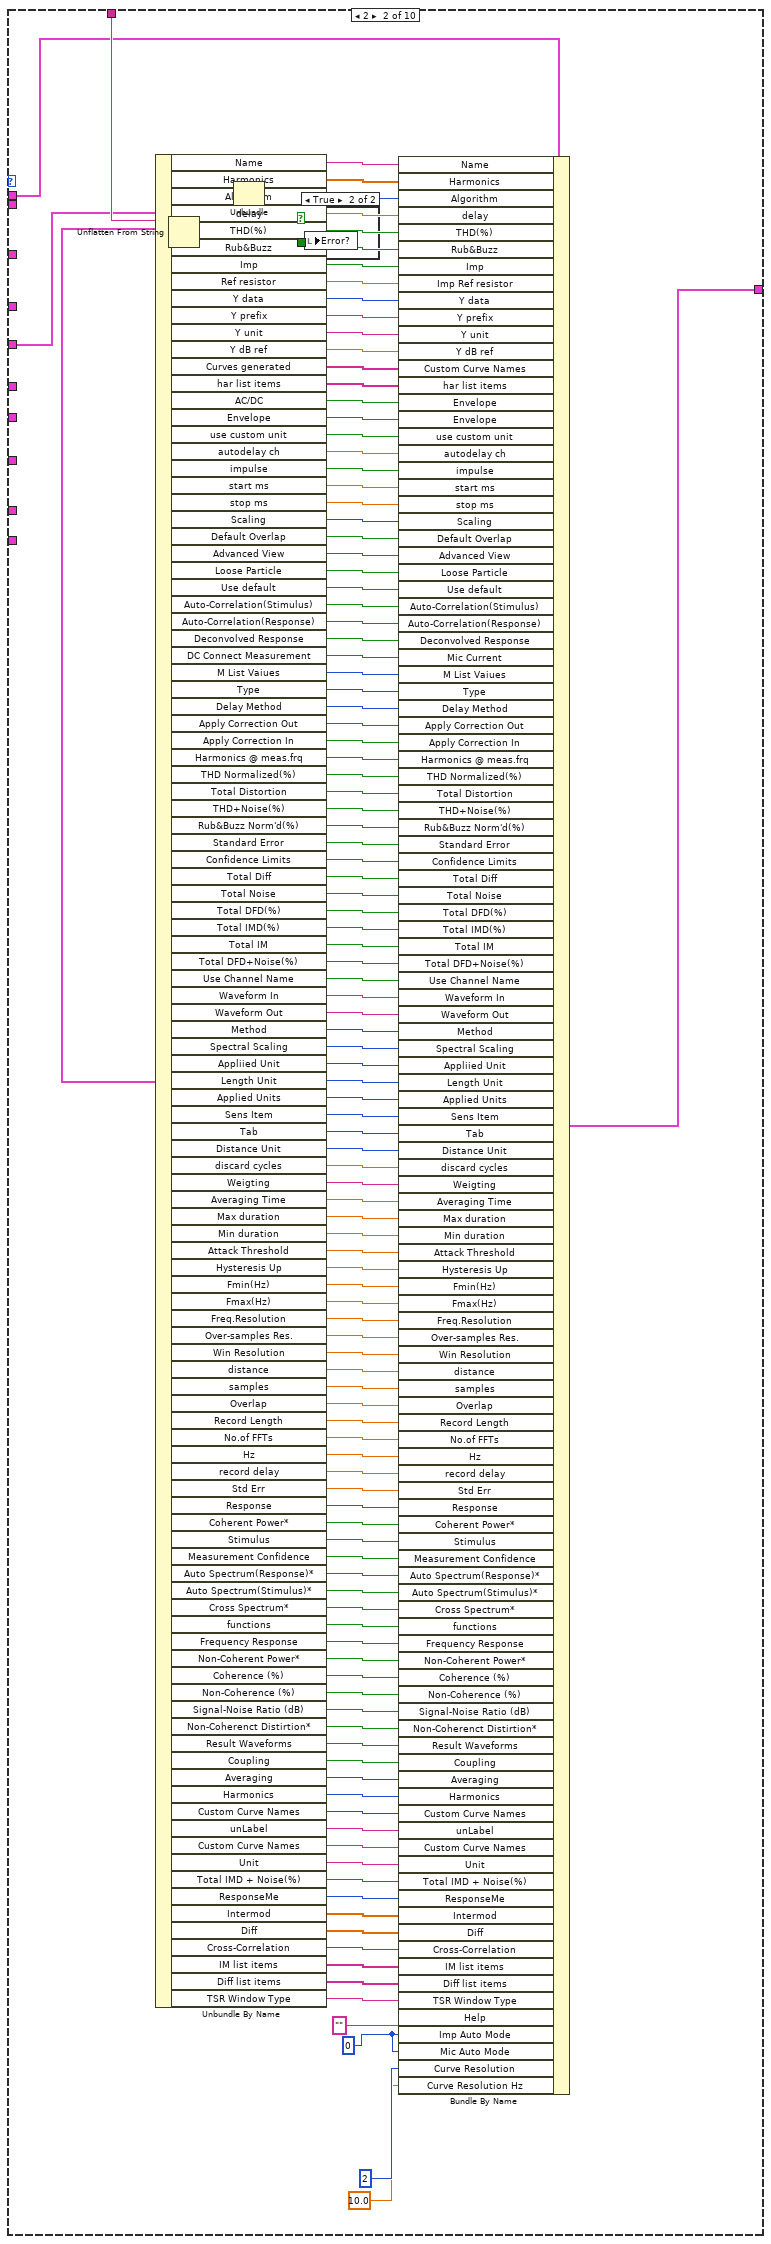
[diagram p4: hidden frame]
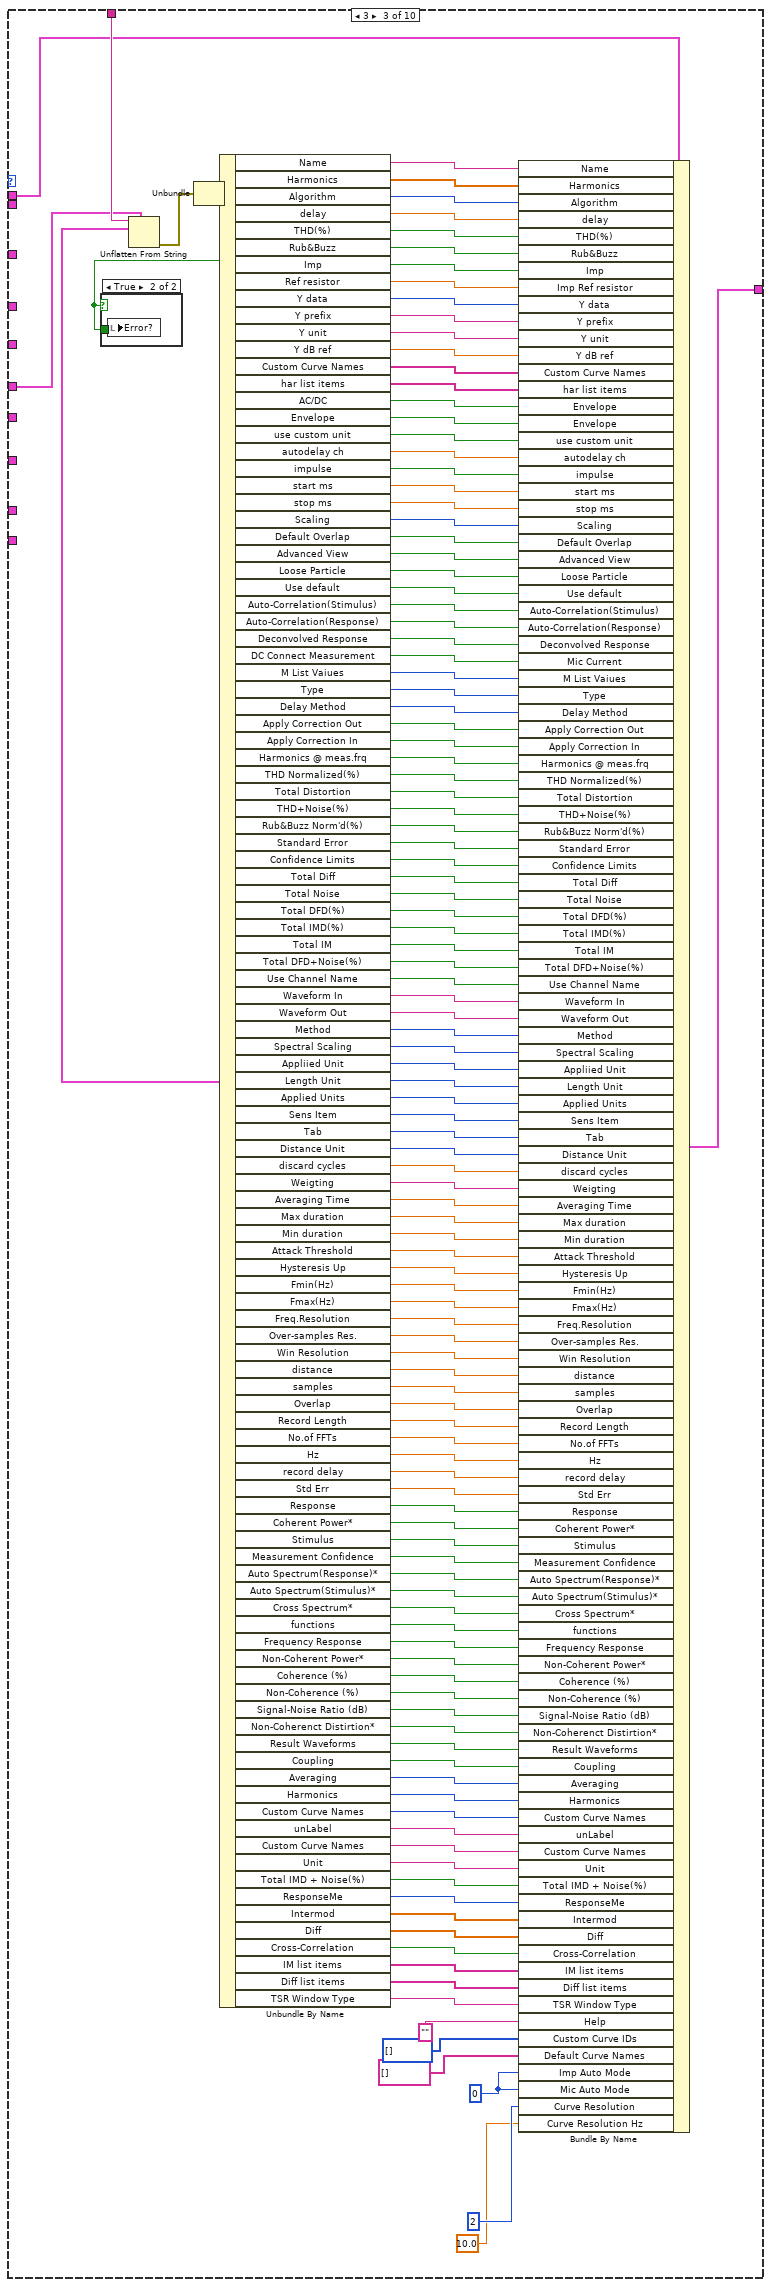
[diagram p6: hidden frame]
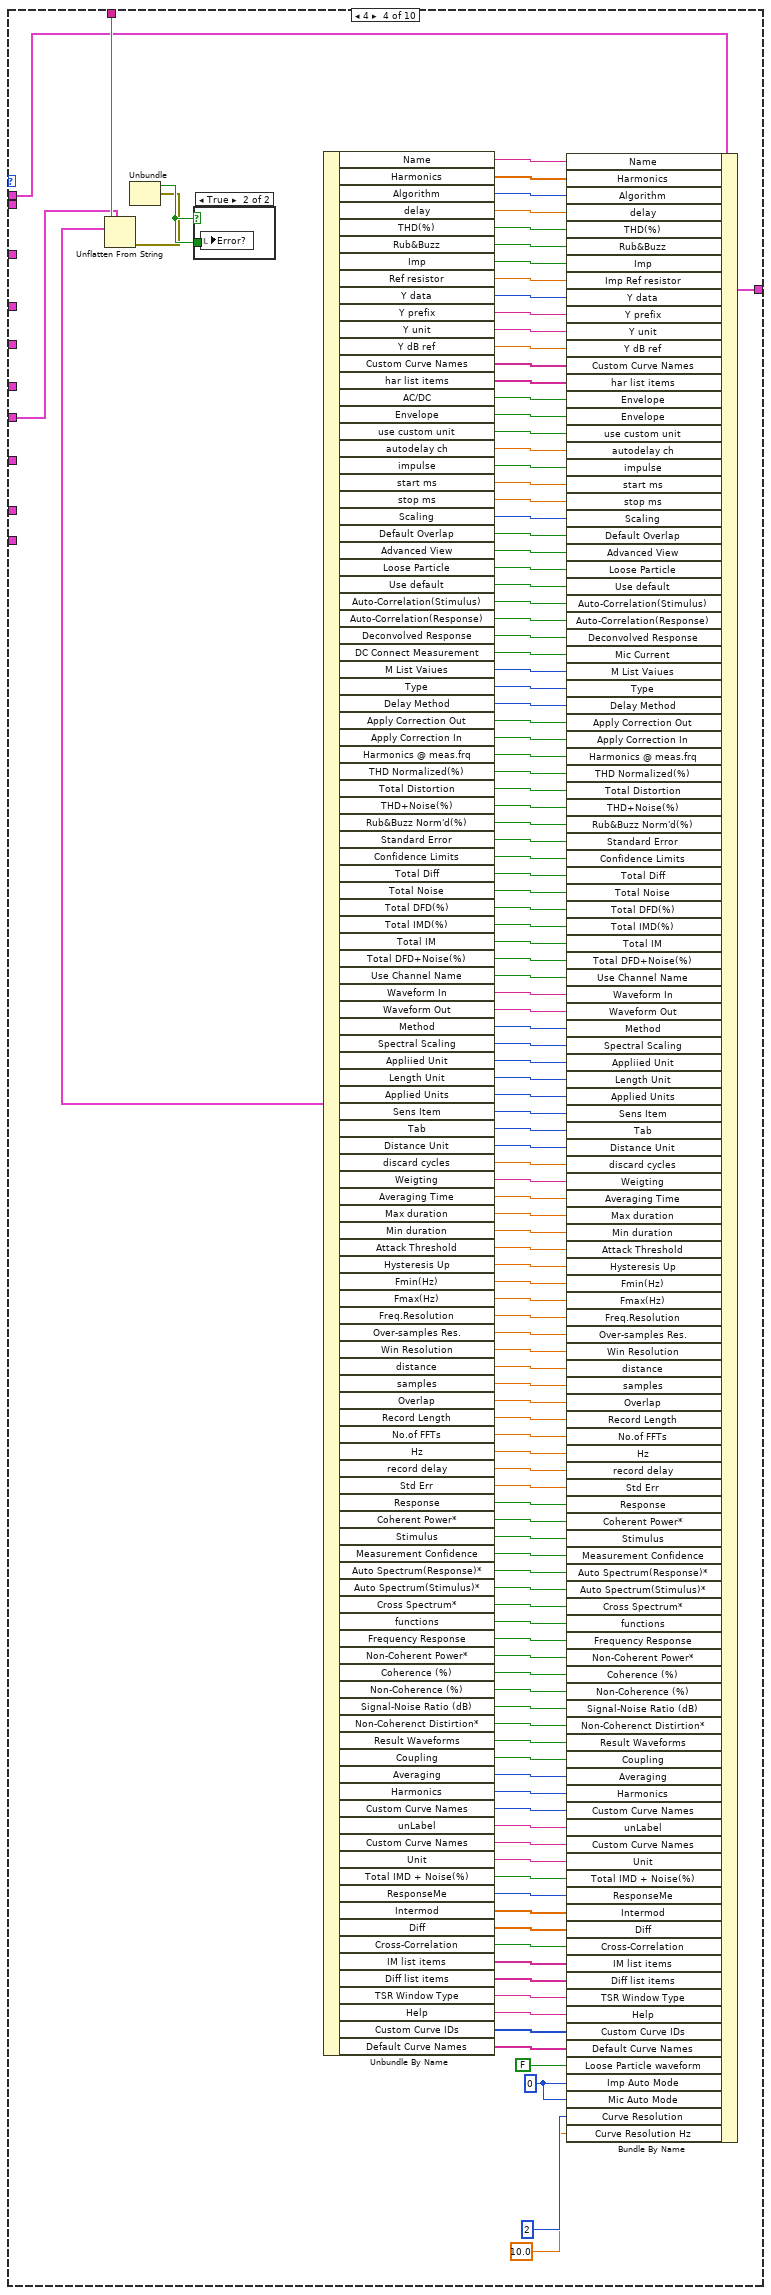
[diagram p8: hidden frame]
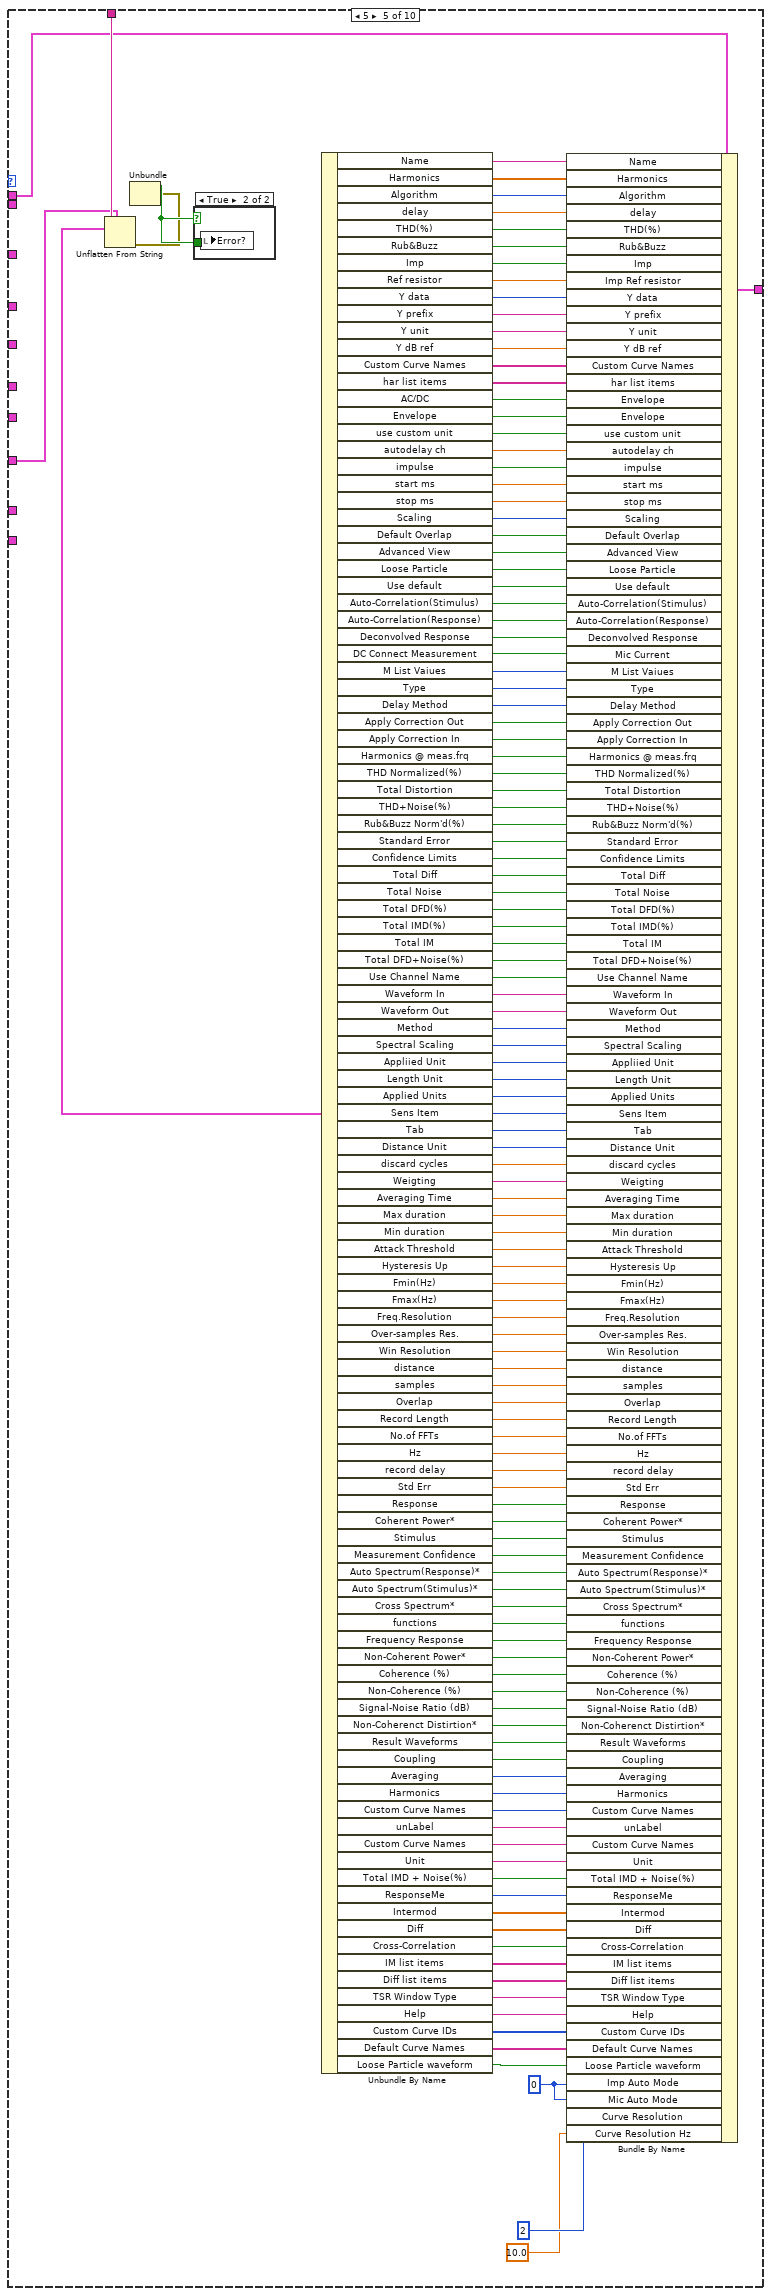
[diagram p10: hidden frame]
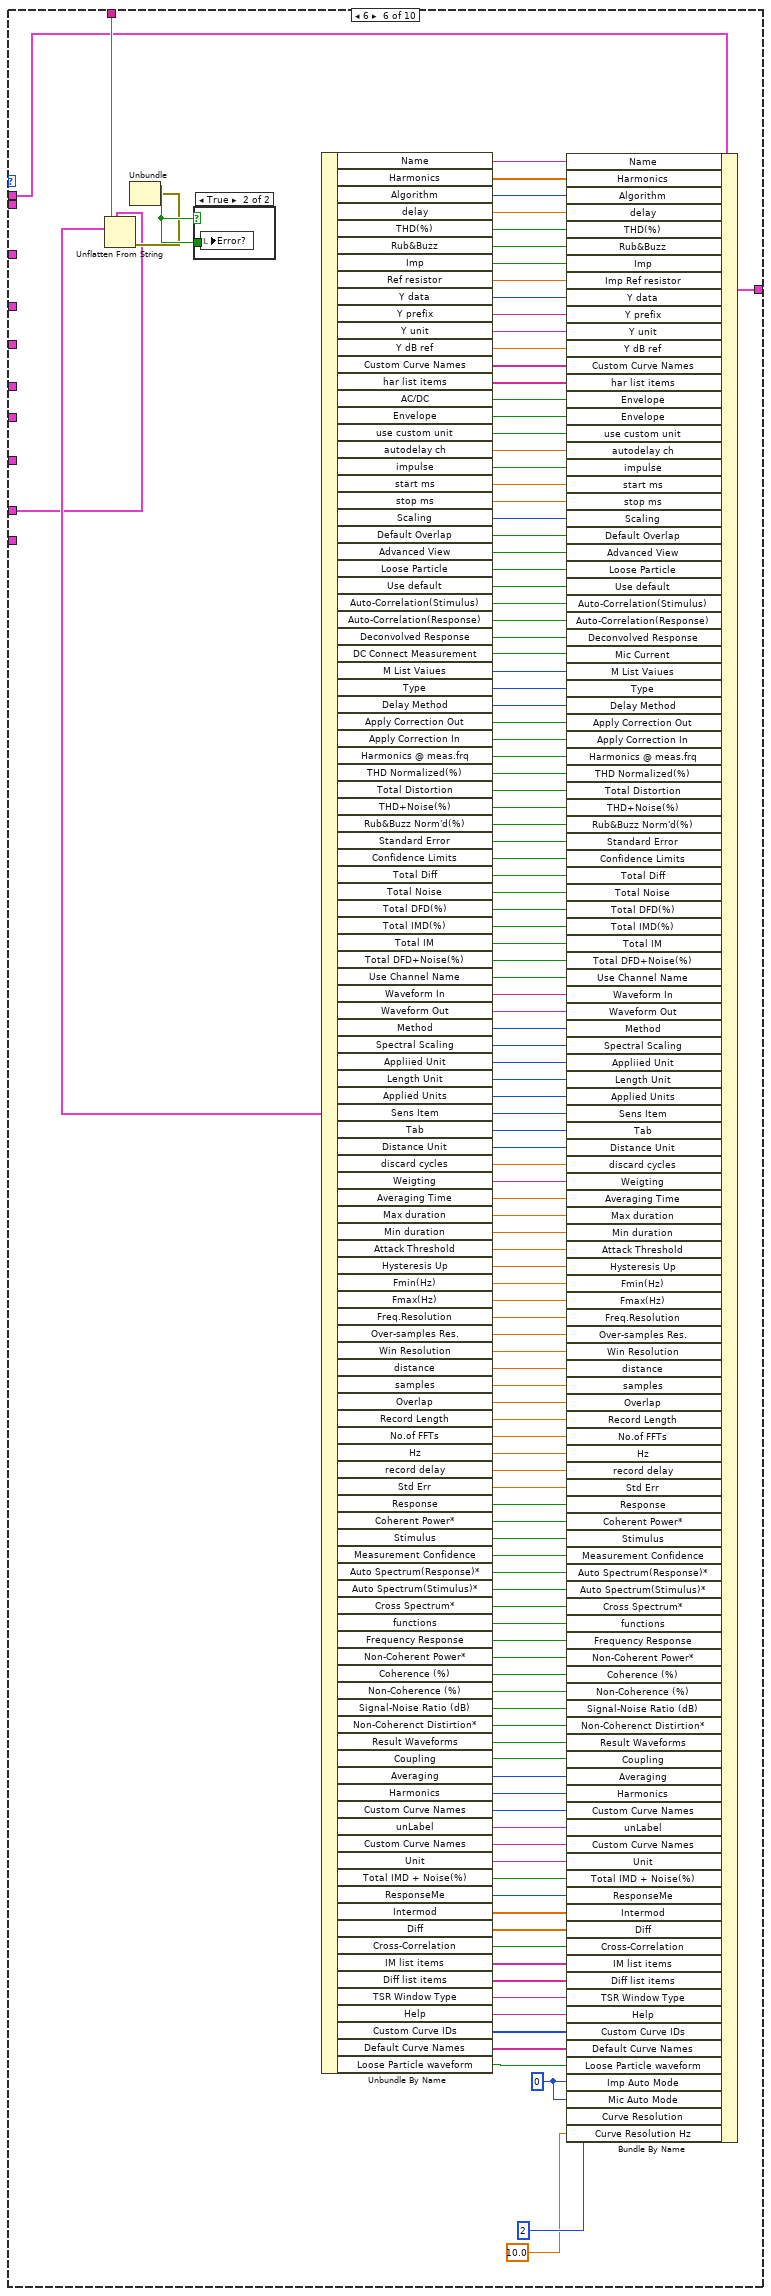
[diagram p12: hidden frame]
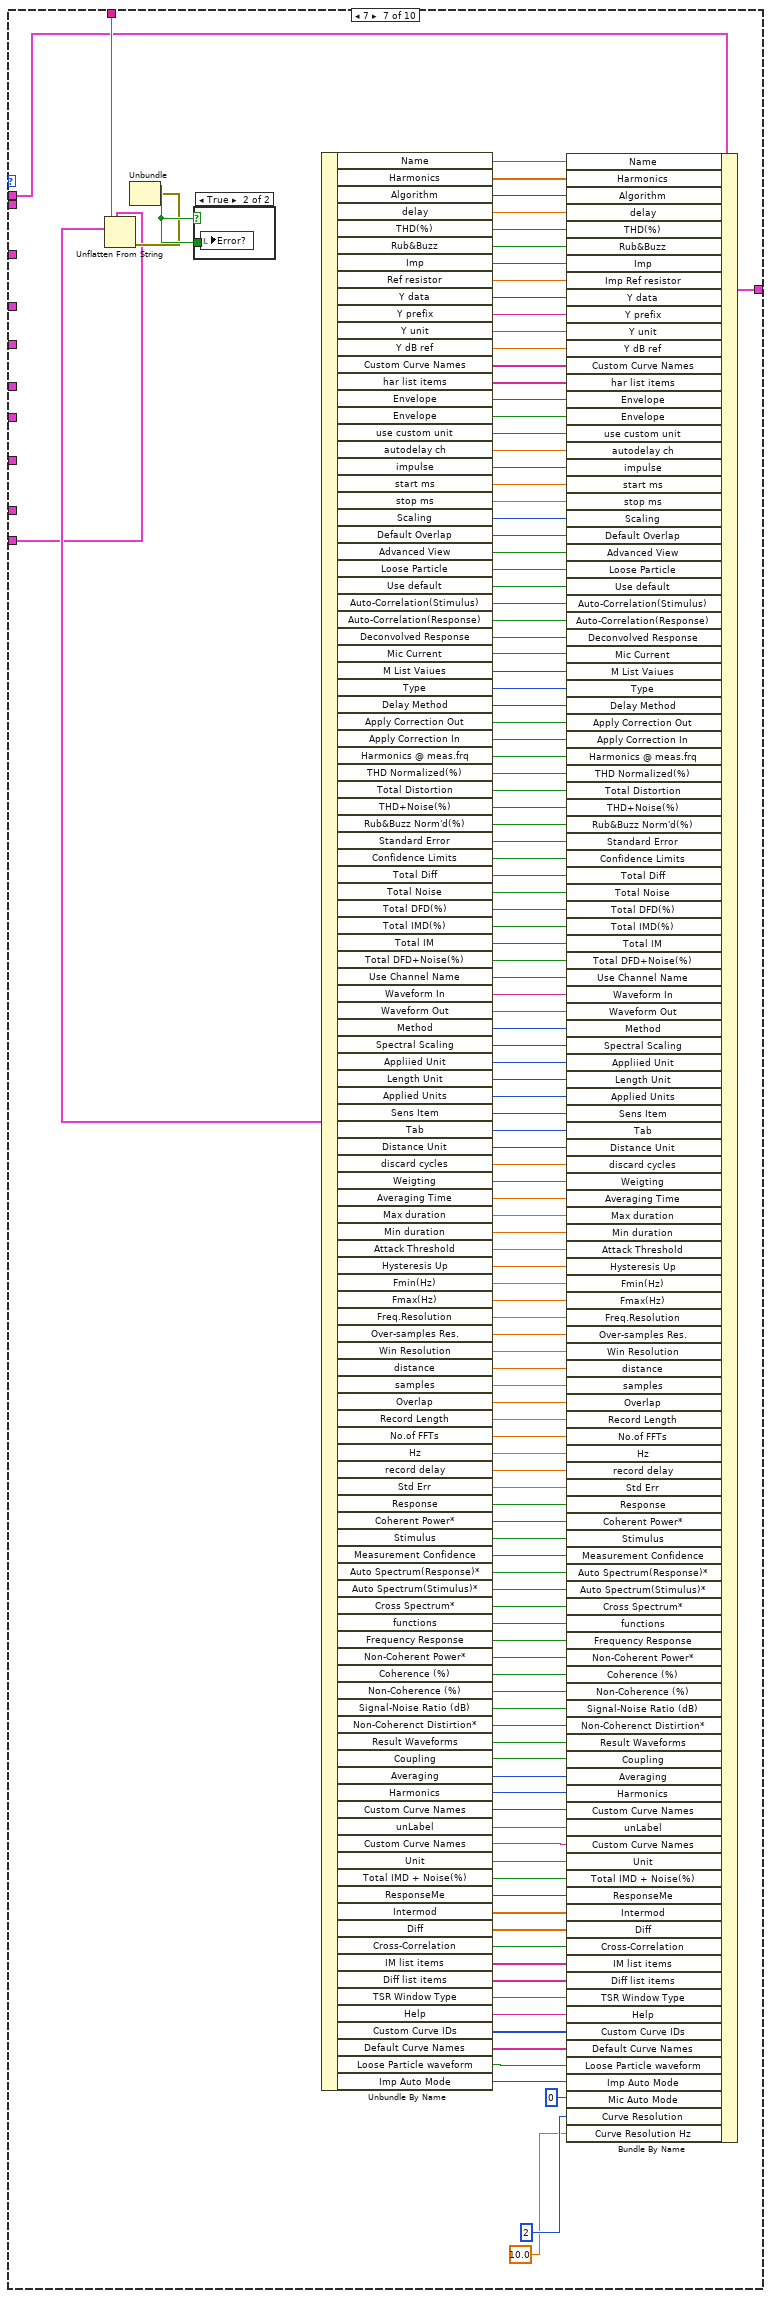
[diagram p14: hidden frame]
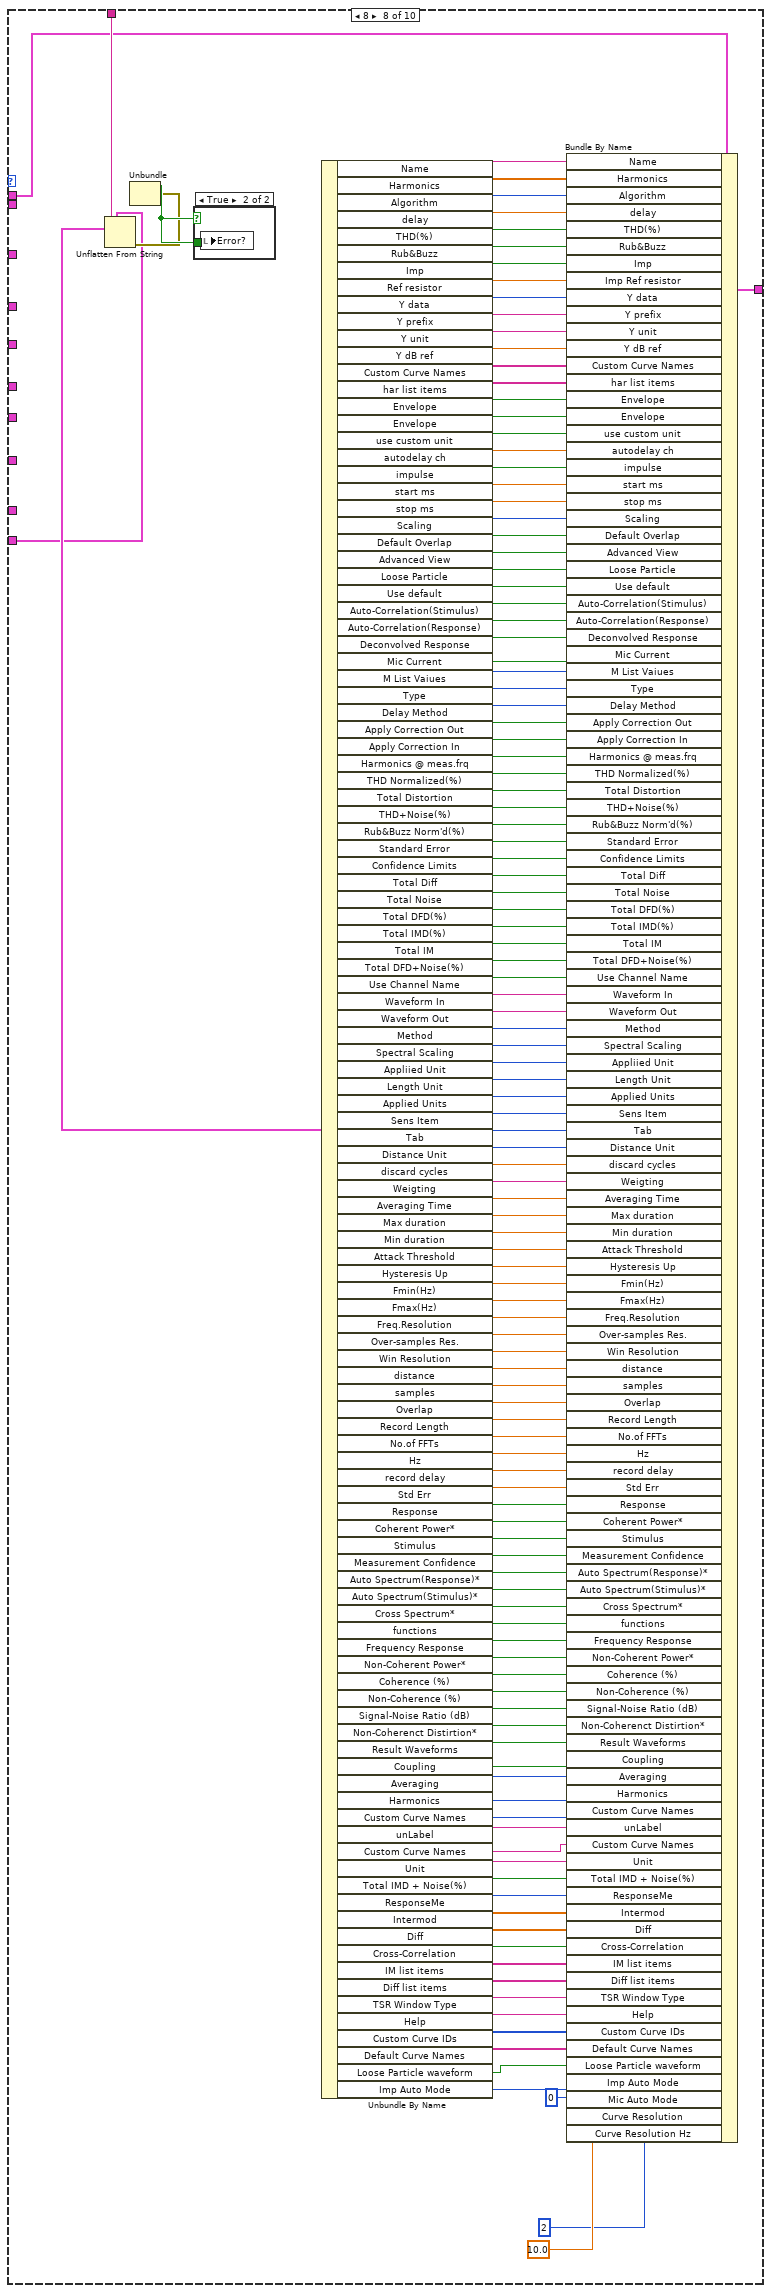
[diagram p16: hidden frame]
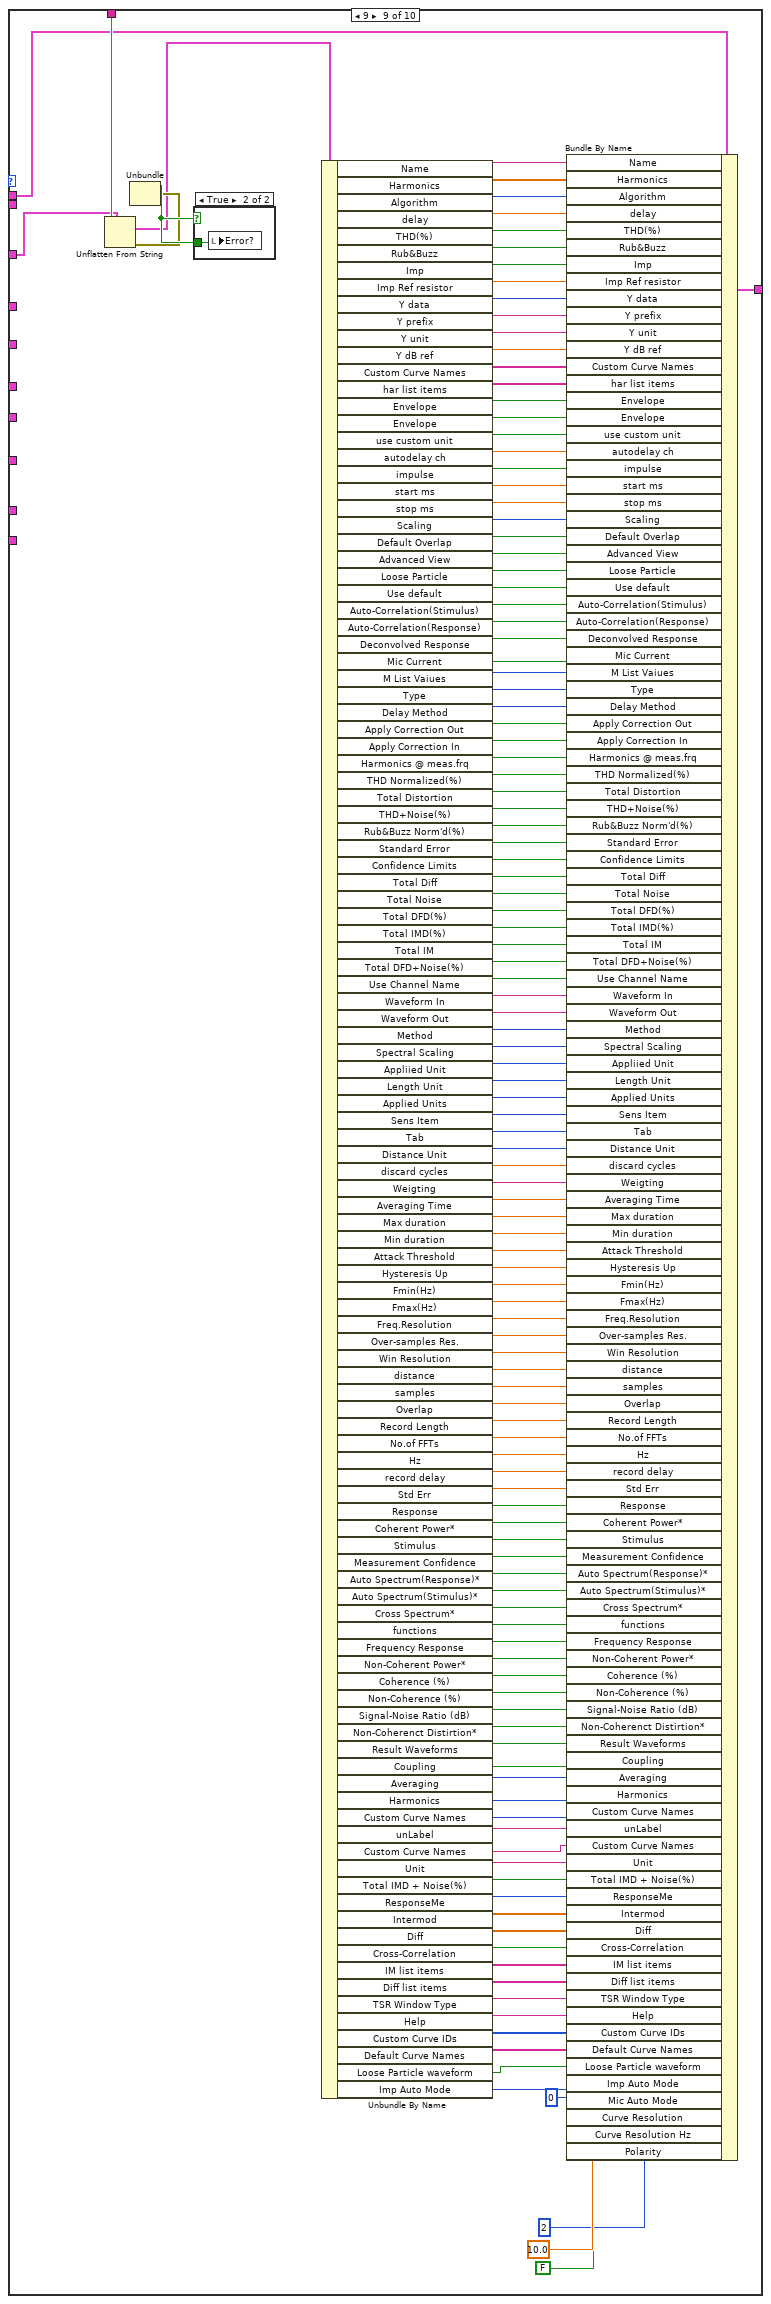
[diagram p18: hidden frame]
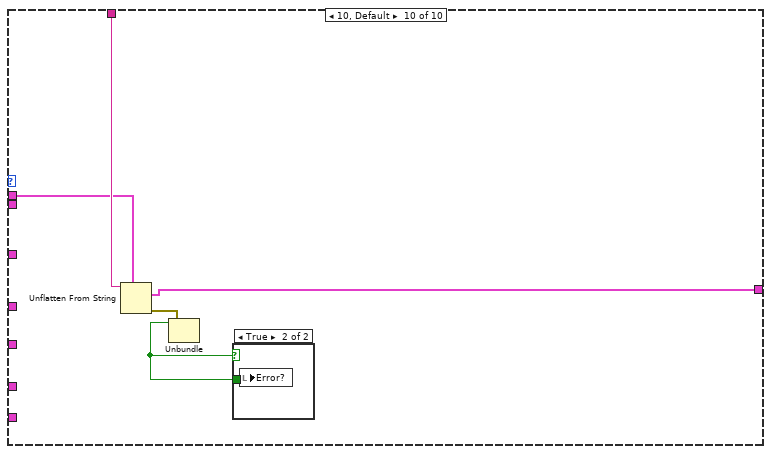
[diagram p20: hidden frame]
diagram:
  w2 = T3 {"Name"="", "Harmonics"=[1.0], " Algorithm"=0, "delay"=0.0, "THD(%)"=FALSE, "Rub&Buzz"=FALSE, "Imp"=FALSE, "Imp Ref resistor"=1.0, "Y data"=0, "Y prefix"="", "Y unit"="", "Y dB ref"=1.0, "Custom Curve Names"=[], "har list items"=[""], "Envelope"=FALSE, "use custom unit"=FALSE, "autodelay ch"=0.0, "impulse"=FALSE, " start ms"=1.0, " stop ms"=1.0, "Scaling"=1, "Default Overlap "=FALSE, "Advanced View"=FALSE, "Loose Particle"=FALSE, "Use default"=FALSE, "Auto-Correlation(Stimulus)"=FALSE, "Auto-Correlation(Response)"=FALSE, "Deconvolved Response"=FALSE, "Mic Current"=FALSE, "M List Vaiues"=0, "Type"=0, "Delay Method"=3, "Apply Correction Out"=FALSE, "Apply Correction In"=FALSE, "Harmonics @ meas.frq"=FALSE, "THD Normalized(%)"=FALSE, "Total Distortion"=FALSE, "THD+Noise(%)"=FALSE, "Rub&Buzz Norm'd(%)"=FALSE, "Standard Error"=FALSE, "Confidence Limits"=FALSE, "Total Diff"=FALSE, "Total Noise"=FALSE, "Total DFD(%)"=FALSE, "Total IMD(%)"=FALSE, "Total IM"=FALSE, "Total DFD+Noise(%)"=FALSE, "Use Channel Name"=FALSE, "Waveform In"="", "Waveform Out"="", "Method"=3, "Spectral Scaling"=3, "Appliied Unit"=1, "Length Unit"=1, "Applied Units"=1, "Sens Item"=0, "Tab"=1, "Distance Unit"=0, "discard cycles"=1.0, "Weigting"="", "Averaging Time"=0.0, "Max duration"=0.0, "Min duration"=0.0, "Attack Threshold"=0.0, "Hysteresis Up"=0.0, "Fmin(Hz)"=0.0, "Fmax(Hz)"=0.0, "Freq.Resolution"=0.0, "Over-samples Res."=0.0, "Win Resolution"=0.0, "distance"=0.0, "samples"=1.0, "Overlap"=1.0, "Record Length"=1.0, "No.of FFTs"=0.0, "Hz"=1.0, "record delay"=1.0, " Std Err"=1.0, "Response"=FALSE, "Coherent Power*"=FALSE, "Stimulus"=FALSE, "Measurement Confidence"=FALSE, "Auto Spectrum(Response)*"=FALSE, "Auto Spectrum(Stimulus)*"=FALSE, "Cross Spectrum*"=FALSE, "functions"=FALSE, "Frequency Response"=FALSE, "Non-Coherent Power*"=FALSE, "Coherence (%)"=FALSE, "Non-Coherence (%)"=FALSE, "Signal-Noise Ratio (dB)"=FALSE, "Non-Coherenct Distirtion*"=FALSE, "Result Waveforms"=FALSE, "Coupling"=FALSE, "Averaging"=0, "Harmonics"=0, "Custom Curve Names"=0, "unLabel"="", "Custom Curve Names"="", "Unit"="", "Total IMD + Noise(%) "=FALSE, "ResponseMe"=1, "Intermod"=[1.0], "Diff\n"=[1.0], "Cross-Correlation"=FALSE, "IM list items"=[""], "Diff list items"=[""], "TSR Window Type"="", "Help"="", "Custom Curve IDs"=[], "Default Curve Names"=[], "Loose Particle waveform"=FALSE, "Perceptual Rub&Buzz"=FALSE, "Imp Auto Mode"=0, "Mic Auto Mode"=0, "Mic Ref resistor"=1.0, "Curve Resolution"=3, "Curve Resolution Hz"=0.0, "Polarity"=FALSE}  # Analysis 10
  w3 = T4 {"Name"="", "Harmonics"=[1.0], " Algorithm"=0, "delay"=0.0, "THD(%)"=FALSE, "Rub&Buzz"=FALSE, "Imp"=FALSE, "Imp Ref resistor"=1.0, "Y data"=0, "Y prefix"="", "Y unit"="", "Y dB ref"=1.0, "Custom Curve Names"=[], "har list items"=[""], "Envelope"=FALSE, "use custom unit"=FALSE, "autodelay ch"=0.0, "impulse"=FALSE, " start ms"=1.0, " stop ms"=1.0, "Scaling"=1, "Default Overlap "=FALSE, "Advanced View"=FALSE, "Loose Particle"=FALSE, "Use default"=FALSE, "Auto-Correlation(Stimulus)"=FALSE, "Auto-Correlation(Response)"=FALSE, "Deconvolved Response"=FALSE, "Mic Current"=FALSE, "M List Vaiues"=0, "Type"=0, "Delay Method"=3, "Apply Correction Out"=FALSE, "Apply Correction In"=FALSE, "Harmonics @ meas.frq"=FALSE, "THD Normalized(%)"=FALSE, "Total Distortion"=FALSE, "THD+Noise(%)"=FALSE, "Rub&Buzz Norm'd(%)"=FALSE, "Standard Error"=FALSE, "Confidence Limits"=FALSE, "Total Diff"=FALSE, "Total Noise"=FALSE, "Total DFD(%)"=FALSE, "Total IMD(%)"=FALSE, "Total IM"=FALSE, "Total DFD+Noise(%)"=FALSE, "Use Channel Name"=FALSE, "Waveform In"="", "Waveform Out"="", "Method"=3, "Spectral Scaling"=3, "Appliied Unit"=1, "Length Unit"=1, "Applied Units"=1, "Sens Item"=0, "Tab"=1, "Distance Unit"=0, "discard cycles"=1.0, "Weigting"="", "Averaging Time"=0.0, "Max duration"=0.0, "Min duration"=0.0, "Attack Threshold"=0.0, "Hysteresis Up"=0.0, "Fmin(Hz)"=0.0, "Fmax(Hz)"=0.0, "Freq.Resolution"=0.0, "Over-samples Res."=0.0, "Win Resolution"=0.0, "distance"=0.0, "samples"=1.0, "Overlap"=1.0, "Record Length"=1.0, "No.of FFTs"=0.0, "Hz"=1.0, "record delay"=1.0, " Std Err"=1.0, "Response"=FALSE, "Coherent Power*"=FALSE, "Stimulus"=FALSE, "Measurement Confidence"=FALSE, "Auto Spectrum(Response)*"=FALSE, "Auto Spectrum(Stimulus)*"=FALSE, "Cross Spectrum*"=FALSE, "functions"=FALSE, "Frequency Response"=FALSE, "Non-Coherent Power*"=FALSE, "Coherence (%)"=FALSE, "Non-Coherence (%)"=FALSE, "Signal-Noise Ratio (dB)"=FALSE, "Non-Coherenct Distirtion*"=FALSE, "Result Waveforms"=FALSE, "Coupling"=FALSE, "Averaging"=0, "Harmonics"=0, "Custom Curve Names"=0, "unLabel"="", "Custom Curve Names"="", "Unit"="", "Total IMD + Noise(%) "=FALSE, "ResponseMe"=1, "Intermod"=[1.0], "Diff\n"=[1.0], "Cross-Correlation"=FALSE, "IM list items"=[""], "Diff list items"=[""], "TSR Window Type"="", "Help"="", "Custom Curve IDs"=[], "Default Curve Names"=[], "Loose Particle waveform"=FALSE, "Perceptual Rub&Buzz"=FALSE, "Imp Auto Mode"=0, "Mic Auto Mode"=0, "Mic Ref resistor"=1.0, "Curve Resolution"=3, "Curve Resolution Hz"=0.0}  # Analysis 9
  w5 = T5 {"Name"="", "Harmonics"=[1.0], " Algorithm"=0, "delay"=0.0, "THD(%)"=FALSE, "Rub&Buzz"=FALSE, "Imp"=FALSE, "Imp Ref resistor"=1.0, "Y data"=0, "Y prefix"="", "Y unit"="", "Y dB ref"=1.0, "Custom Curve Names"=[], "har list items"=[""], "Envelope"=FALSE, "use custom unit"=FALSE, "autodelay ch"=0.0, "impulse"=FALSE, " start ms"=1.0, " stop ms"=1.0, "Scaling"=1, "Default Overlap "=FALSE, "Advanced View"=FALSE, "Loose Particle"=FALSE, "Use default"=FALSE, "Auto-Correlation(Stimulus)"=FALSE, "Auto-Correlation(Response)"=FALSE, "Deconvolved Response"=FALSE, "Mic Current"=FALSE, "M List Vaiues"=0, "Type"=0, "Delay Method"=3, "Apply Correction Out"=FALSE, "Apply Correction In"=FALSE, "Harmonics @ meas.frq"=FALSE, "THD Normalized(%)"=FALSE, "Total Distortion"=FALSE, "THD+Noise(%)"=FALSE, "Rub&Buzz Norm'd(%)"=FALSE, "Standard Error"=FALSE, "Confidence Limits"=FALSE, "Total Diff"=FALSE, "Total Noise"=FALSE, "Total DFD(%)"=FALSE, "Total IMD(%)"=FALSE, "Total IM"=FALSE, "Total DFD+Noise(%)"=FALSE, "Use Channel Name"=FALSE, "Waveform In"="", "Waveform Out"="", "Method"=3, "Spectral Scaling"=3, "Appliied Unit"=1, "Length Unit"=1, "Applied Units"=1, "Sens Item"=0, "Tab"=1, "Distance Unit"=0, "discard cycles"=1.0, "Weigting"="", "Averaging Time"=0.0, "Max duration"=0.0, "Min duration"=0.0, "Attack Threshold"=0.0, "Hysteresis Up"=0.0, "Fmin(Hz)"=0.0, "Fmax(Hz)"=0.0, "Freq.Resolution"=0.0, "Over-samples Res."=0.0, "Win Resolution"=0.0, "distance"=0.0, "samples"=1.0, "Overlap"=1.0, "Record Length"=1.0, "No.of FFTs"=0.0, "Hz"=1.0, "record delay"=1.0, " Std Err"=1.0, "Response"=FALSE, "Coherent Power*"=FALSE, "Stimulus"=FALSE, "Measurement Confidence"=FALSE, "Auto Spectrum(Response)*"=FALSE, "Auto Spectrum(Stimulus)*"=FALSE, "Cross Spectrum*"=FALSE, "functions"=FALSE, "Frequency Response"=FALSE, "Non-Coherent Power*"=FALSE, "Coherence (%)"=FALSE, "Non-Coherence (%)"=FALSE, "Signal-Noise Ratio (dB)"=FALSE, "Non-Coherenct Distirtion*"=FALSE, "Result Waveforms"=FALSE, "Coupling"=FALSE, "Averaging"=0, "Harmonics"=0, "Custom Curve Names"=0, "unLabel"="", "Custom Curve Names"="", "Unit"="", "Total IMD + Noise(%) "=FALSE, "ResponseMe"=1, "Intermod"=[1.0], "Diff\n"=[1.0], "Cross-Correlation"=FALSE, "IM list items"=[""], "Diff list items"=[""], "TSR Window Type"="", "Help"="", "Custom Curve IDs"=[], "Default Curve Names"=[], "Loose Particle waveform"=FALSE, "Perceptual Rub&Buzz"=FALSE, "Imp Auto Mode"=0, "Mic Auto Mode"=0, "Mic Ref resistor"=1.0}  # Analysis 8
  w4 = T6 {"Name"="", "Harmonics"=[1.0], " Algorithm"=0, "delay"=0.0, "THD(%)"=FALSE, "Rub&Buzz"=FALSE, "Imp"=FALSE, "Ref resistor"=1.0, "Y data"=0, "Y prefix"="", "Y unit"="", "Y dB ref"=1.0, "Custom Curve Names"=[], "har list items"=[""], "Envelope"=FALSE, "use custom unit"=FALSE, "autodelay ch"=0.0, "impulse"=FALSE, " start ms"=1.0, " stop ms"=1.0, "Scaling"=1, "Default Overlap "=FALSE, "Advanced View"=FALSE, "Loose Particle"=FALSE, "Use default"=FALSE, "Auto-Correlation(Stimulus)"=FALSE, "Auto-Correlation(Response)"=FALSE, "Deconvolved Response"=FALSE, "Mic Current"=FALSE, "M List Vaiues"=0, "Type"=0, "Delay Method"=3, "Apply Correction Out"=FALSE, "Apply Correction In"=FALSE, "Harmonics @ meas.frq"=FALSE, "THD Normalized(%)"=FALSE, "Total Distortion"=FALSE, "THD+Noise(%)"=FALSE, "Rub&Buzz Norm'd(%)"=FALSE, "Standard Error"=FALSE, "Confidence Limits"=FALSE, "Total Diff"=FALSE, "Total Noise"=FALSE, "Total DFD(%)"=FALSE, "Total IMD(%)"=FALSE, "Total IM"=FALSE, "Total DFD+Noise(%)"=FALSE, "Use Channel Name"=FALSE, "Waveform In"="", "Waveform Out"="", "Method"=3, "Spectral Scaling"=3, "Appliied Unit"=1, "Length Unit"=1, "Applied Units"=1, "Sens Item"=0, "Tab"=1, "Distance Unit"=0, "discard cycles"=1.0, "Weigting"="", "Averaging Time"=0.0, "Max duration"=0.0, "Min duration"=0.0, "Attack Threshold"=0.0, "Hysteresis Up"=0.0, "Fmin(Hz)"=0.0, "Fmax(Hz)"=0.0, "Freq.Resolution"=0.0, "Over-samples Res."=0.0, "Win Resolution"=0.0, "distance"=0.0, "samples"=1.0, "Overlap"=1.0, "Record Length"=1.0, "No.of FFTs"=0.0, "Hz"=1.0, "record delay"=1.0, " Std Err"=1.0, "Response"=FALSE, "Coherent Power*"=FALSE, "Stimulus"=FALSE, "Measurement Confidence"=FALSE, "Auto Spectrum(Response)*"=FALSE, "Auto Spectrum(Stimulus)*"=FALSE, "Cross Spectrum*"=FALSE, "functions"=FALSE, "Frequency Response"=FALSE, "Non-Coherent Power*"=FALSE, "Coherence (%)"=FALSE, "Non-Coherence (%)"=FALSE, "Signal-Noise Ratio (dB)"=FALSE, "Non-Coherenct Distirtion*"=FALSE, "Result Waveforms"=FALSE, "Coupling"=FALSE, "Averaging"=0, "Harmonics"=0, "Custom Curve Names"=0, "unLabel"="", "Custom Curve Names"="", "Unit"="", "Total IMD + Noise(%) "=FALSE, "ResponseMe"=1, "Intermod"=[1.0], "Diff\n"=[1.0], "Cross-Correlation"=FALSE, "IM list items"=[""], "Diff list items"=[""], "TSR Window Type"="", "Help"="", "Custom Curve IDs"=[], "Default Curve Names"=[], "Loose Particle waveform"=FALSE, "Perceptual Rub&Buzz"=FALSE, "Imp Auto Mode"=0}  # Analysis 7
  w6 = T7 {"Name"="", "Harmonics"=[1.0], " Algorithm"=0, "delay"=0.0, "THD(%)"=FALSE, "Rub&Buzz"=FALSE, "Imp"=FALSE, "Ref resistor"=1.0, "Y data"=0, "Y prefix"="", "Y unit"="", "Y dB ref"=1.0, "Custom Curve Names"=[], "har list items"=[""], "AC/DC"=FALSE, "Envelope"=FALSE, "use custom unit"=FALSE, "autodelay ch"=0.0, "impulse"=FALSE, " start ms"=1.0, " stop ms"=1.0, "Scaling"=0, "Default Overlap "=FALSE, "Advanced View"=FALSE, "Loose Particle"=FALSE, "Use default"=FALSE, "Auto-Correlation(Stimulus)"=FALSE, "Auto-Correlation(Response)"=FALSE, "Deconvolved Response"=FALSE, "DC Connect Measurement"=FALSE, "M List Vaiues"=0, "Type"=3, "Delay Method"=3, "Apply Correction Out"=FALSE, "Apply Correction In"=FALSE, "Harmonics @ meas.frq"=FALSE, "THD Normalized(%)"=FALSE, "Total Distortion"=FALSE, "THD+Noise(%)"=FALSE, "Rub&Buzz Norm'd(%)"=FALSE, "Standard Error"=FALSE, "Confidence Limits"=FALSE, "Total Diff"=FALSE, "Total Noise"=FALSE, "Total DFD(%)"=FALSE, "Total IMD(%)"=FALSE, "Total IM"=FALSE, "Total DFD+Noise(%)"=FALSE, "Use Channel Name"=FALSE, "Waveform In"="", "Waveform Out"="", "Method"=3, "Spectral Scaling"=1, "Appliied Unit"=1, "Length Unit"=1, "Applied Units"=0, "Sens Item"=1, "Tab"=0, "Distance Unit"=1, "discard cycles"=0.0, "Weigting"="", "Averaging Time"=0.0, "Max duration"=0.0, "Min duration"=0.0, "Attack Threshold"=0.0, "Hysteresis Up"=0.0, "Fmin(Hz)"=0.0, "Fmax(Hz)"=0.0, "Freq.Resolution"=0.0, "Over-samples Res."=0.0, "Win Resolution"=0.0, "distance"=1.0, "samples"=1.0, "Overlap"=1.0, "Record Length"=0.0, "No.of FFTs"=1.0, "Hz"=1.0, "record delay"=1.0, " Std Err"=1.0, "Response"=FALSE, "Coherent Power*"=FALSE, "Stimulus"=FALSE, "Measurement Confidence"=FALSE, "Auto Spectrum(Response)*"=FALSE, "Auto Spectrum(Stimulus)*"=FALSE, "Cross Spectrum*"=FALSE, "functions"=FALSE, "Frequency Response"=FALSE, "Non-Coherent Power*"=FALSE, "Coherence (%)"=FALSE, "Non-Coherence (%)"=FALSE, "Signal-Noise Ratio (dB)"=FALSE, "Non-Coherenct Distirtion*"=FALSE, "Result Waveforms"=FALSE, "Coupling"=FALSE, "Averaging"=0, "AC/DC 2"=FALSE, "Harmonics"=0, "Custom Curve Names"=0, "unLabel"="", "Custom Curve Names"="", "Unit"="", "Total IMD + Noise(%) "=FALSE, "ResponseMe"=1, "Intermod"=[1.0], "Diff\n"=[1.0], "Cross-Correlation"=FALSE, "IM list items"=[""], "Diff list items"=[""], "TSR Window Type"="", "Help"="", "Custom Curve IDs"=[], "Default Curve Names"=[], "Loose Particle waveform"=FALSE, "Perceptual Rub&Buzz"=FALSE}  # Analysis6
  w8 = T8 {"Name"="", "Harmonics"=[1.0], " Algorithm"=0, "delay"=0.0, "THD(%)"=FALSE, "Rub&Buzz"=FALSE, "Imp"=FALSE, "Ref resistor"=1.0, "Y data"=0, "Y prefix"="", "Y unit"="", "Y dB ref"=1.0, "Custom Curve Names"=[], "har list items"=[""], "AC/DC"=FALSE, "Envelope"=FALSE, "use custom unit"=FALSE, "autodelay ch"=0.0, "impulse"=FALSE, " start ms"=1.0, " stop ms"=1.0, "Scaling"=0, "Default Overlap "=FALSE, "Advanced View"=FALSE, "Loose Particle"=FALSE, "Use default"=FALSE, "Auto-Correlation(Stimulus)"=FALSE, "Auto-Correlation(Response)"=FALSE, "Deconvolved Response"=FALSE, "DC Connect Measurement"=FALSE, "M List Vaiues"=0, "Type"=3, "Delay Method"=3, "Apply Correction Out"=FALSE, "Apply Correction In"=FALSE, "Harmonics @ meas.frq"=FALSE, "THD Normalized(%)"=FALSE, "Total Distortion"=FALSE, "THD+Noise(%)"=FALSE, "Rub&Buzz Norm'd(%)"=FALSE, "Standard Error"=FALSE, "Confidence Limits"=FALSE, "Total Diff"=FALSE, "Total Noise"=FALSE, "Total DFD(%)"=FALSE, "Total IMD(%)"=FALSE, "Total IM"=FALSE, "Total DFD+Noise(%)"=FALSE, "Use Channel Name"=FALSE, "Waveform In"="", "Waveform Out"="", "Method"=3, "Spectral Scaling"=1, "Appliied Unit"=1, "Length Unit"=1, "Applied Units"=0, "Sens Item"=1, "Tab"=0, "Distance Unit"=1, "discard cycles"=0.0, "Weigting"="", "Averaging Time"=0.0, "Max duration"=0.0, "Min duration"=0.0, "Attack Threshold"=0.0, "Hysteresis Up"=0.0, "Fmin(Hz)"=0.0, "Fmax(Hz)"=0.0, "Freq.Resolution"=0.0, "Over-samples Res."=0.0, "Win Resolution"=0.0, "distance"=1.0, "samples"=1.0, "Overlap"=1.0, "Record Length"=0.0, "No.of FFTs"=1.0, "Hz"=1.0, "record delay"=1.0, " Std Err"=1.0, "Response"=FALSE, "Coherent Power*"=FALSE, "Stimulus"=FALSE, "Measurement Confidence"=FALSE, "Auto Spectrum(Response)*"=FALSE, "Auto Spectrum(Stimulus)*"=FALSE, "Cross Spectrum*"=FALSE, "functions"=FALSE, "Frequency Response"=FALSE, "Non-Coherent Power*"=FALSE, "Coherence (%)"=FALSE, "Non-Coherence (%)"=FALSE, "Signal-Noise Ratio (dB)"=FALSE, "Non-Coherenct Distirtion*"=FALSE, "Result Waveforms"=FALSE, "Coupling"=FALSE, "Averaging"=0, "AC/DC 2"=FALSE, "Harmonics"=0, "Custom Curve Names"=0, "unLabel"="", "Custom Curve Names"="", "Unit"="", "Total IMD + Noise(%) "=FALSE, "ResponseMe"=1, "Intermod"=[1.0], "Diff\n"=[1.0], "Cross-Correlation"=FALSE, "IM list items"=[""], "Diff list items"=[""], "TSR Window Type"="", "Help"="", "Custom Curve IDs"=[], "Default Curve Names"=[]}  # Analysis4
  w9 = T9 {"Name"="", "Harmonics"=[1.0], " Algorithm"=0, "delay"=0.0, "THD(%)"=FALSE, "Rub&Buzz"=FALSE, "Imp"=FALSE, "Ref resistor"=1.0, "Y data"=0, "Y prefix"="", "Y unit"="", "Y dB ref"=1.0, "Custom Curve Names"=[], "har list items"=[""], "AC/DC"=FALSE, "Envelope"=FALSE, "use custom unit"=FALSE, "autodelay ch"=0.0, "impulse"=FALSE, " start ms"=1.0, " stop ms"=1.0, "Scaling"=0, "Default Overlap "=FALSE, "Advanced View"=FALSE, "Loose Particle"=FALSE, "Use default"=FALSE, "Auto-Correlation(Stimulus)"=FALSE, "Auto-Correlation(Response)"=FALSE, "Deconvolved Response"=FALSE, "DC Connect Measurement"=FALSE, "M List Vaiues"=0, "Type"=3, "Delay Method"=3, "Apply Correction Out"=FALSE, "Apply Correction In"=FALSE, "Harmonics @ meas.frq"=FALSE, "THD Normalized(%)"=FALSE, "Total Distortion"=FALSE, "THD+Noise(%)"=FALSE, "Rub&Buzz Norm'd(%)"=FALSE, "Standard Error"=FALSE, "Confidence Limits"=FALSE, "Total Diff"=FALSE, "Total Noise"=FALSE, "Total DFD(%)"=FALSE, "Total IMD(%)"=FALSE, "Total IM"=FALSE, "Total DFD+Noise(%)"=FALSE, "Use Channel Name"=FALSE, "Waveform In"="", "Waveform Out"="", "Method"=3, "Spectral Scaling"=1, "Appliied Unit"=1, "Length Unit"=1, "Applied Units"=0, "Sens Item"=1, "Tab"=0, "Distance Unit"=1, "discard cycles"=0.0, "Weigting"="", "Averaging Time"=0.0, "Max duration"=0.0, "Min duration"=0.0, "Attack Threshold"=0.0, "Hysteresis Up"=0.0, "Fmin(Hz)"=0.0, "Fmax(Hz)"=0.0, "Freq.Resolution"=0.0, "Over-samples Res."=0.0, "Win Resolution"=0.0, "distance"=1.0, "samples"=1.0, "Overlap"=1.0, "Record Length"=0.0, "No.of FFTs"=1.0, "Hz"=1.0, "record delay"=1.0, " Std Err"=1.0, "Response"=FALSE, "Coherent Power*"=FALSE, "Stimulus"=FALSE, "Measurement Confidence"=FALSE, "Auto Spectrum(Response)*"=FALSE, "Auto Spectrum(Stimulus)*"=FALSE, "Cross Spectrum*"=FALSE, "functions"=FALSE, "Frequency Response"=FALSE, "Non-Coherent Power*"=FALSE, "Coherence (%)"=FALSE, "Non-Coherence (%)"=FALSE, "Signal-Noise Ratio (dB)"=FALSE, "Non-Coherenct Distirtion*"=FALSE, "Result Waveforms"=FALSE, "Coupling"=FALSE, "Averaging"=0, "AC/DC 2"=FALSE, "Harmonics"=0, "Custom Curve Names"=0, "unLabel"="", "Custom Curve Names"="", "Unit"="", "Total IMD + Noise(%) "=FALSE, "ResponseMe"=1, "Intermod"=[1.0], "Diff\n"=[1.0], "Cross-Correlation"=FALSE, "IM list items"=[""], "Diff list items"=[""], "TSR Window Type"="", "Help"=""}  # Analysis3
  w10 = T10 {"Name"="", "Harmonics"=[1.0], " Algorithm"=0, "delay"=0.0, "THD(%)"=FALSE, "Rub&Buzz"=FALSE, "Imp"=FALSE, "Ref resistor"=1.0, "Y data"=0, "Y prefix"="", "Y unit"="", "Y dB ref"=1.0, "Curves generated"=[], "har list items"=[""], "AC/DC"=FALSE, "Envelope"=FALSE, "use custom unit"=FALSE, "autodelay ch"=0.0, "impulse"=FALSE, " start ms"=1.0, " stop ms"=1.0, "Scaling"=0, "Default Overlap "=FALSE, "Advanced View"=FALSE, "Loose Particle"=FALSE, "Use default"=FALSE, "Auto-Correlation(Stimulus)"=FALSE, "Auto-Correlation(Response)"=FALSE, "Deconvolved Response"=FALSE, "DC Connect Measurement"=FALSE, "M List Vaiues"=0, "Type"=3, "Delay Method"=3, "Apply Correction Out"=FALSE, "Apply Correction In"=FALSE, "Harmonics @ meas.frq"=FALSE, "THD Normalized(%)"=FALSE, "Total Distortion"=FALSE, "THD+Noise(%)"=FALSE, "Rub&Buzz Norm'd(%)"=FALSE, "Standard Error"=FALSE, "Confidence Limits"=FALSE, "Total Diff"=FALSE, "Total Noise"=FALSE, "Total DFD(%)"=FALSE, "Total IMD(%)"=FALSE, "Total IM"=FALSE, "Total DFD+Noise(%)"=FALSE, "Use Channel Name"=FALSE, "Waveform In"="", "Waveform Out"="", "Method"=3, "Spectral Scaling"=1, "Appliied Unit"=1, "Length Unit"=1, "Applied Units"=0, "Sens Item"=1, "Tab"=0, "Distance Unit"=1, "discard cycles"=0.0, "Weigting"="", "Averaging Time"=0.0, "Max duration"=0.0, "Min duration"=0.0, "Attack Threshold"=0.0, "Hysteresis Up"=0.0, "Fmin(Hz)"=0.0, "Fmax(Hz)"=0.0, "Freq.Resolution"=0.0, "Over-samples Res."=0.0, "Win Resolution"=0.0, "distance"=1.0, "samples"=1.0, "Overlap"=1.0, "Record Length"=0.0, "No.of FFTs"=1.0, "Hz"=1.0, "record delay"=1.0, " Std Err"=1.0, "Response"=FALSE, "Coherent Power*"=FALSE, "Stimulus"=FALSE, "Measurement Confidence"=FALSE, "Auto Spectrum(Response)*"=FALSE, "Auto Spectrum(Stimulus)*"=FALSE, "Cross Spectrum*"=FALSE, "functions"=FALSE, "Frequency Response"=FALSE, "Non-Coherent Power*"=FALSE, "Coherence (%)"=FALSE, "Non-Coherence (%)"=FALSE, "Signal-Noise Ratio (dB)"=FALSE, "Non-Coherenct Distirtion*"=FALSE, "Result Waveforms"=FALSE, "Coupling"=FALSE, "Averaging"=0, "AC/DC 2"=FALSE, "Harmonics"=0, "Custom Curve Names"=0, "unLabel"="", "Custom Curve Names"="", "Unit"="", "Total IMD + Noise(%) "=FALSE, "ResponseMe"=1, "Intermod"=[1.0], "Diff\n"=[1.0], "Cross-Correlation"=FALSE, "IM list items"=[""], "Diff list items"=[""], "TSR Window Type"=""}  # Analysis2
  w7 = T11 {"Name"="", "Harmonics"=[1.0], " Algorithm"=0, "delay"=0.0, "THD(%)"=FALSE, "Rub&Buzz"=FALSE, "Imp"=FALSE, "Ref resistor"=1.0, "Y data"=0, "Y prefix"="", "Y unit"="", "Y dB ref"=1.0, "Custom Curve Names"=[], "har list items"=[""], "AC/DC"=FALSE, "Envelope"=FALSE, "use custom unit"=FALSE, "autodelay ch"=0.0, "impulse"=FALSE, " start ms"=1.0, " stop ms"=1.0, "Scaling"=0, "Default Overlap "=FALSE, "Advanced View"=FALSE, "Loose Particle"=FALSE, "Use default"=FALSE, "Auto-Correlation(Stimulus)"=FALSE, "Auto-Correlation(Response)"=FALSE, "Deconvolved Response"=FALSE, "DC Connect Measurement"=FALSE, "M List Vaiues"=0, "Type"=3, "Delay Method"=3, "Apply Correction Out"=FALSE, "Apply Correction In"=FALSE, "Harmonics @ meas.frq"=FALSE, "THD Normalized(%)"=FALSE, "Total Distortion"=FALSE, "THD+Noise(%)"=FALSE, "Rub&Buzz Norm'd(%)"=FALSE, "Standard Error"=FALSE, "Confidence Limits"=FALSE, "Total Diff"=FALSE, "Total Noise"=FALSE, "Total DFD(%)"=FALSE, "Total IMD(%)"=FALSE, "Total IM"=FALSE, "Total DFD+Noise(%)"=FALSE, "Use Channel Name"=FALSE, "Waveform In"="", "Waveform Out"="", "Method"=3, "Spectral Scaling"=1, "Appliied Unit"=1, "Length Unit"=1, "Applied Units"=0, "Sens Item"=1, "Tab"=0, "Distance Unit"=1, "discard cycles"=0.0, "Weigting"="", "Averaging Time"=0.0, "Max duration"=0.0, "Min duration"=0.0, "Attack Threshold"=0.0, "Hysteresis Up"=0.0, "Fmin(Hz)"=0.0, "Fmax(Hz)"=0.0, "Freq.Resolution"=0.0, "Over-samples Res."=0.0, "Win Resolution"=0.0, "distance"=1.0, "samples"=1.0, "Overlap"=1.0, "Record Length"=0.0, "No.of FFTs"=1.0, "Hz"=1.0, "record delay"=1.0, " Std Err"=1.0, "Response"=FALSE, "Coherent Power*"=FALSE, "Stimulus"=FALSE, "Measurement Confidence"=FALSE, "Auto Spectrum(Response)*"=FALSE, "Auto Spectrum(Stimulus)*"=FALSE, "Cross Spectrum*"=FALSE, "functions"=FALSE, "Frequency Response"=FALSE, "Non-Coherent Power*"=FALSE, "Coherence (%)"=FALSE, "Non-Coherence (%)"=FALSE, "Signal-Noise Ratio (dB)"=FALSE, "Non-Coherenct Distirtion*"=FALSE, "Result Waveforms"=FALSE, "Coupling"=FALSE, "Averaging"=0, "AC/DC 2"=FALSE, "Harmonics"=0, "Custom Curve Names"=0, "unLabel"="", "Custom Curve Names"="", "Unit"="", "Total IMD + Noise(%) "=FALSE, "ResponseMe"=1, "Intermod"=[1.0], "Diff\n"=[1.0], "Cross-Correlation"=FALSE, "IM list items"=[""], "Diff list items"=[""], "TSR Window Type"="", "Help"="", "Custom Curve IDs"=[], "Default Curve Names"=[], "Loose Particle waveform"=FALSE}  # Analysis5
  w11 = T12 {"Name"="", "Harmonics"=[], " Algorithm"=0, "delay"=0.0, "THD(%)"=FALSE, "Rub&Buzz"=FALSE, "Imp"=FALSE, "Ref resistor"=0.0, "Y data"=0, "Y prefix"="", "Y unit"="", "Y dB ref"=0.0, "Curves generated"=[], "har list items"=[], "AC/DC"=FALSE, "Envelope"=FALSE, "use custom unit"=FALSE, "autodelay ch"=0.0, "impulse"=FALSE, " start ms"=0.0, " stop ms"=0.0, "Scaling"=0, "Default Overlap "=FALSE, "Advanced View"=FALSE, "Loose Particle"=FALSE, "Use default"=FALSE, "Auto-Correlation(Stimulus)"=FALSE, "Auto-Correlation(Response)"=FALSE, "Deconvolved Response"=FALSE, "DC Connect Measurement"=FALSE, "M List Vaiues"=0, "Type"=0, "Delay Method"=0, "Apply Correction Out"=FALSE, "Apply Correction In"=FALSE, "Harmonics @ meas.frq"=FALSE, "THD Normalized(%)"=FALSE, "Total Distortion"=FALSE, "THD+Noise(%)"=FALSE, "Rub&Buzz Norm'd(%)"=FALSE, "Standard Error"=FALSE, "Confidence Limits"=FALSE, "Total Diff"=FALSE, "Total Noise"=FALSE, "Total DFD(%)"=FALSE, "Total IMD(%)"=FALSE, "Total IM"=FALSE, "Total DFD+Noise(%)"=FALSE, "Use Channel Name"=FALSE, "Waveform In"="", "Waveform Out"="", "Method"=0, "Spectral Scaling"=0, "Appliied Unit"=0, "Length Unit"=0, "Applied Units"=0, "Sens Item"=0, "Tab"=0, "Ring"=0, "discard cycles"=0.0, "Weigting"="", "Averaging Time"=0.0, "Max duration"=0.0, "Min duration"=0.0, "Attack Threshold"=0.0, "Hysteresis Up"=0.0, "Fmin(Hz)"=0.0, "Fmax(Hz)"=0.0, "Freq.Resolution"=0.0, "Over-samples Res."=0.0, "Win Resolution"=0.0, "distance"=0.0, "samples"=0.0, "Overlap"=0.0, "Record Length"=0.0, "No.of FFTs"=0.0, "Hz"=0.0, "record delay"=0.0, " Std Err"=0.0, "Response"=FALSE, "Coherent Power*"=FALSE, "Stimulus"=FALSE, "Measurement Confidence"=FALSE, "Auto Spectrum(Response)*"=FALSE, "Auto Spectrum(Stimulus)*"=FALSE, "Cross Spectrum*"=FALSE, "functions"=FALSE, "Frequency Response"=FALSE, "Non-Coherent Power*"=FALSE, "Coherence (%)"=FALSE, "Non-Coherence (%)"=FALSE, "Signal-Noise Ratio (dB)"=FALSE, "Non-Coherenct Dustirtion*"=FALSE, "Result Waveforms"=FALSE, "Coupling"=FALSE, "Averaging"=0, "AC/DC 2"=FALSE, "Harmonics"=0, "Custom Curve Names"=0, "unLabel"="", "Custom Curve Names"="", "Unit"="", "Total IMD + Noise(%) "=FALSE, "ResponseMe"=0, "Orders 2"=[], "Orders1\n"=[], "Cross-Correlation"=FALSE, "IM list items"=[], "Diff list items"=[]}  # Analysis1
  n1 = stacked-sequence {
    tunnel: [w19] -> w12
    frame #0 {
      w19 = FALSE
      "Error?" <- w19
    }
  }
  n2 = Empty String/Path?(string/path="Unflatten Analysis") -> (empty?=w17:bool)
  n3 = case shown="False" w17 {
    tunnel: "Unflatten Analysis" -> [w48 _]
    tunnel: [w40 u16 0] -> w15
    tunnel: [w32 u8 0] -> w16
    tunnel: [w33 "(no data input)" ("substring")] -> w14
    tunnel: w12 -> [_ _]
    tunnel: [w31 w1186] -> w1
    tunnel: w5 -> [w30 _]
    tunnel: w11 -> [w29 _]
    tunnel: w10 -> [w28 _]
    tunnel: w9 -> [w26 _]
    tunnel: w8 -> [w25 _]
    tunnel: w7 -> [w24 _]
    tunnel: w6 -> [w23 _]
    tunnel: w4 -> [w22 _]
    tunnel: w3 -> [w21 _]
    tunnel: w2 -> [w20 w1186]
    frame False {
      w37 = "                "  # 16 spaces
      w38 = "Analysis"  # cluster name
      w35 = 16  # name field length
      # "check for correct name"
      # "array dimensions\n(now inactive)"
      # "version number"
      # "data type name"
      n4 = Search/Split String(string=w48, offset (0)=64 ("header length")) -> (substring before match=w42:string, match + rest of string=w43:string)  [unwired: 2 out]
      n5 = Concatenate Strings(w38, w37) -> (w36:string)
      n6 = String Subset(string=w36, length (rest)=w35) -> (substring=w34:string)  [unwired: 1 out]
      n7 = Search/Split String(string=w42, offset (0)=w35) -> (substring before match=w33:string, match + rest of string=w39:string)  [unwired: 2 out]
      n8 = Equal?(x=w34, y=w33) -> (x = y?=w41:bool)
      n9 = String To Byte Array(string=w39) -> (unsigned byte array=w47:u8[])
      n10 = Array To Cluster(array=w47) -> (cluster=w46:T13)
      n11 = Unbundle(w46) -> ("unsigned byte array[0]"=w45:u8, "unsigned byte array[1]"=w44:u8, "unsigned byte array[2]"=w32:u8)
      n12 = Join Numbers(hi=w45, lo=w44) -> ((hi.lo)=w40:u16)
      n13 = case shown="False" w41 {
        tunnel: w43 -> [_ w67]
        tunnel: w40 -> [_ w66]
        tunnel: [w49 w65] -> w31
        tunnel: w30 -> [_ w64]
        tunnel: w29 -> [_ w63]
        tunnel: w28 -> [_ w62]
        tunnel: w26 -> [_ w61]
        tunnel: w25 -> [_ w60]
        tunnel: w24 -> [_ w59]
        tunnel: w23 -> [_ w58]
        tunnel: w22 -> [_ w57]
        tunnel: w21 -> [_ w56]
        tunnel: w20 -> [w49 w55]
        frame False {
          n14 = call "CRYGet Error Message.vi"("Error No"=0, "Kind"="Analysis") -> ("Message"=w51:string, "Window Title"=w50:string)  [unwired: 4 in, 4 out]
          n15 = local write "Error?"(TRUE) -> ()
          n16 = call "CRYMessage Dialog.vi"("Window Title"=w50, "Message Content"=w51) -> ()  [unwired: 8 in, 2 out]
        }
        frame True {
          n17 = case "version" shown="1" w66 {
            tunnel: w67 -> [w186 w307 w430 w554 w678 w802 w927 w1052 w1178 w1184]
            tunnel: [w181 w303 w426 w550 w674 w798 w923 w1048 w1174 w1181] -> w65
            tunnel: w64 -> [_ _ _ _ _ _ _ _ _ _]
            tunnel: w63 -> [w183 _ _ _ _ _ _ _ _ _]
            tunnel: w62 -> [_ w193 _ _ _ _ _ _ _ _]
            tunnel: w61 -> [_ _ w315 _ _ _ _ _ _ _]
            tunnel: w60 -> [_ _ _ w442 _ _ _ _ _ _]
            tunnel: w59 -> [_ _ _ _ w562 _ _ _ _ _]
            tunnel: w58 -> [_ _ _ _ _ w684 _ _ _ _]
            tunnel: w57 -> [_ _ _ _ _ _ w812 w937 _ _]
            tunnel: w56 -> [_ _ _ _ _ _ _ _ w1055 _]
            tunnel: w55 -> [w68 w188 w309 w432 w556 w680 w804 w929 w1056 w1180]
            frame 1 {
              n18 = Unflatten From String(type=w183, binary string=w186) -> (value=w182:T12, error out=w184:errorcluster)  [unwired: 1 in, 3 out]
              n19 = Unbundle(w184) -> ("status"=w185:bool)  [unwired: 2 out]
              n20 = case shown="True" w185 {
                tunnel: w185 -> [_ w187]
                frame False {
                }
                frame True {
                  n21 = local write "Error?"(w187) -> ()
                }
              }
              n22 = Unbundle By Name(w182) -> ("Name"=w180:string, "Harmonics"=w179:dbl[], "Algorithm"=w178:u16, "delay"=w177:dbl, "THD(%)"=w176:bool, "Rub&Buzz"=w175:bool, "Imp"=w174:bool, "Ref resistor"=w173:dbl, "Y data"=w172:u16, "Y prefix"=w171:string, "Y unit"=w170:string, "Y dB ref"=w169:dbl, "Curves generated"=w168:string[], "har list items"=w167:string[], "AC/DC"=w166:bool, "Envelope"=w165:bool, "use custom unit"=w164:bool, "autodelay ch"=w163:dbl, "impulse"=w162:bool, "start ms"=w161:dbl, "stop ms"=w160:dbl, "Scaling"=w159:i32, "Default Overlap"=w158:bool, "Advanced View"=w157:bool, "Loose Particle"=w156:bool, "Use default"=w155:bool, "Auto-Correlation(Stimulus)"=w154:bool, "Auto-Correlation(Response)"=w153:bool, "Deconvolved Response"=w152:bool, "DC Connect Measurement"=w151:bool, "M List Vaiues"=w150:u16, "Type"=w149:u16, "Delay Method"=w148:u16, "Apply Correction Out"=w147:bool, "Apply Correction In"=w146:bool, "Harmonics @ meas.frq"=w145:bool, "THD Normalized(%)"=w144:bool, "Total Distortion"=w143:bool, "THD+Noise(%)"=w142:bool, "Rub&Buzz Norm'd(%)"=w141:bool, "Standard Error"=w140:bool, "Confidence Limits"=w139:bool, "Total Diff"=w138:bool, "Total Noise"=w137:bool, "Total DFD(%)"=w136:bool, "Total IMD(%)"=w135:bool, "Total IM"=w134:bool, "Total DFD+Noise(%)"=w133:bool, "Use Channel Name"=w132:bool, "Waveform In"=w131:string, "Waveform Out"=w130:string, "Method"=w129:u16, "Spectral Scaling"=w128:u16, "Appliied Unit"=w127:u16, "Length Unit"=w126:u16, "Applied Units"=w125:u16, "Sens Item"=w124:u16, "Tab"=w123:i32, "Ring"=w122:u16, "discard cycles"=w121:dbl, "Weigting"=w120:string, "Averaging Time"=w119:dbl, "Max duration"=w118:dbl, "Min duration"=w117:dbl, "Attack Threshold"=w116:dbl, "Hysteresis Up"=w115:dbl, "Fmin(Hz)"=w114:dbl, "Fmax(Hz)"=w113:dbl, "Freq.Resolution"=w112:dbl, "Over-samples Res."=w111:dbl, "Win Resolution"=w110:dbl, "distance"=w109:dbl, "samples"=w108:dbl, "Overlap"=w107:dbl, "Record Length"=w106:dbl, "No.of FFTs"=w105:dbl, "Hz"=w104:dbl, "record delay"=w103:dbl, "Std Err"=w102:dbl, "Response"=w101:bool, "Coherent Power*"=w100:bool, "Stimulus"=w99:bool, "Measurement Confidence"=w98:bool, "Auto Spectrum(Response)*"=w97:bool, "Auto Spectrum(Stimulus)*"=w96:bool, "Cross Spectrum*"=w95:bool, "functions"=w94:bool, "Frequency Response"=w93:bool, "Non-Coherent Power*"=w92:bool, "Coherence (%)"=w91:bool, "Non-Coherence (%)"=w90:bool, "Signal-Noise Ratio (dB)"=w89:bool, "Non-Coherenct Dustirtion*"=w88:bool, "Result Waveforms"=w87:bool, "Coupling"=w86:bool, "Averaging"=w85:u16, "Harmonics"=w84:i32, "Custom Curve Names"=w72:i32, "unLabel"=w83:string, "Custom Curve Names"=w82:string, "Unit"=w81:string, "Total IMD + Noise(%)"=w80:bool, "ResponseMe"=w79:u16, "Orders 2"=w78:dbl[], "Orders1"=w77:dbl[], "Cross-Correlation"=w76:bool, "IM list items"=w75:string[], "Diff list items"=w74:string[])
              n23 = Bundle By Name(cluster=w68, "Name"=w180, "Harmonics"=w179, "Algorithm"=w178, "delay"=w177, "THD(%)"=w176, "Rub&Buzz"=w175, "Imp"=w174, "Imp Ref resistor"=w173, "Y data"=w172, "Y prefix"=w171, "Y unit"=w170, "Y dB ref"=w169, "Custom Curve Names"=w168, "har list items"=w167, "Envelope"=w166, "Envelope"=w165, "use custom unit"=w164, "autodelay ch"=w163, "impulse"=w162, "start ms"=w161, "stop ms"=w160, "Scaling"=w159, "Default Overlap"=w158, "Advanced View"=w157, "Loose Particle"=w156, "Use default"=w155, "Auto-Correlation(Stimulus)"=w154, "Auto-Correlation(Response)"=w153, "Deconvolved Response"=w152, "Mic Current"=w151, "M List Vaiues"=w150, "Type"=w149, "Delay Method"=w148, "Apply Correction Out"=w147, "Apply Correction In"=w146, "Harmonics @ meas.frq"=w145, "THD Normalized(%)"=w144, "Total Distortion"=w143, "THD+Noise(%)"=w142, "Rub&Buzz Norm'd(%)"=w141, "Standard Error"=w140, "Confidence Limits"=w139, "Total Diff"=w138, "Total Noise"=w137, "Total DFD(%)"=w136, "Total IMD(%)"=w135, "Total IM"=w134, "Total DFD+Noise(%)"=w133, "Use Channel Name"=w132, "Waveform In"=w131, "Waveform Out"=w130, "Method"=w129, "Spectral Scaling"=w128, "Appliied Unit"=w127, "Length Unit"=w126, "Applied Units"=w125, "Sens Item"=w124, "Tab"=w123, "Distance Unit"=w122, "discard cycles"=w121, "Weigting"=w120, "Averaging Time"=w119, "Max duration"=w118, "Min duration"=w117, "Attack Threshold"=w116, "Hysteresis Up"=w115, "Fmin(Hz)"=w114, "Fmax(Hz)"=w113, "Freq.Resolution"=w112, "Over-samples Res."=w111, "Win Resolution"=w110, "distance"=w109, "samples"=w108, "Overlap"=w107, "Record Length"=w106, "No.of FFTs"=w105, "Hz"=w104, "record delay"=w103, "Std Err"=w102, "Response"=w101, "Coherent Power*"=w100, "Stimulus"=w99, "Measurement Confidence"=w98, "Auto Spectrum(Response)*"=w97, "Auto Spectrum(Stimulus)*"=w96, "Cross Spectrum*"=w95, "functions"=w94, "Frequency Response"=w93, "Non-Coherent Power*"=w92, "Coherence (%)"=w91, "Non-Coherence (%)"=w90, "Signal-Noise Ratio (dB)"=w89, "Non-Coherenct Distirtion*"=w88, "Result Waveforms"=w87, "Coupling"=w86, "Averaging"=w85, "Harmonics"=w84, "Custom Curve Names"=w72, "unLabel"=w83, "Custom Curve Names"=w82, "Unit"=w81, "Total IMD + Noise(%)"=w80, "ResponseMe"=w79, "Intermod"=w78, "Diff"=w77, "Cross-Correlation"=w76, "IM list items"=w75, "Diff list items"=w74, "TSR Window Type"="", "Imp Auto Mode"=u16 0, "Curve Resolution"=u16 2, "Curve Resolution Hz"=10.0) -> (w181:T3)
            }
            frame 2 {
              w191 = u16 0 ("Imp Auto Mode")
              n24 = Unflatten From String(type=w193, binary string=w307) -> (value=w304:T10, error out=w305:errorcluster)  [unwired: 1 in, 3 out]
              n25 = Unbundle By Name(w304) -> ("Name"=w302:string, "Harmonics"=w301:dbl[], "Algorithm"=w300:u16, "delay"=w299:dbl, "THD(%)"=w298:bool, "Rub&Buzz"=w297:bool, "Imp"=w296:bool, "Ref resistor"=w295:dbl, "Y data"=w294:u16, "Y prefix"=w293:string, "Y unit"=w292:string, "Y dB ref"=w291:dbl, "Curves generated"=w290:string[], "har list items"=w289:string[], "AC/DC"=w288:bool, "Envelope"=w287:bool, "use custom unit"=w286:bool, "autodelay ch"=w285:dbl, "impulse"=w284:bool, "start ms"=w283:dbl, "stop ms"=w282:dbl, "Scaling"=w281:i32, "Default Overlap"=w280:bool, "Advanced View"=w279:bool, "Loose Particle"=w278:bool, "Use default"=w277:bool, "Auto-Correlation(Stimulus)"=w276:bool, "Auto-Correlation(Response)"=w275:bool, "Deconvolved Response"=w274:bool, "DC Connect Measurement"=w273:bool, "M List Vaiues"=w272:u16, "Type"=w271:u16, "Delay Method"=w270:u16, "Apply Correction Out"=w269:bool, "Apply Correction In"=w268:bool, "Harmonics @ meas.frq"=w267:bool, "THD Normalized(%)"=w266:bool, "Total Distortion"=w265:bool, "THD+Noise(%)"=w264:bool, "Rub&Buzz Norm'd(%)"=w263:bool, "Standard Error"=w262:bool, "Confidence Limits"=w261:bool, "Total Diff"=w260:bool, "Total Noise"=w259:bool, "Total DFD(%)"=w258:bool, "Total IMD(%)"=w257:bool, "Total IM"=w256:bool, "Total DFD+Noise(%)"=w255:bool, "Use Channel Name"=w254:bool, "Waveform In"=w253:string, "Waveform Out"=w252:string, "Method"=w251:u16, "Spectral Scaling"=w250:u16, "Appliied Unit"=w249:u16, "Length Unit"=w248:u16, "Applied Units"=w247:u16, "Sens Item"=w246:u16, "Tab"=w245:i32, "Distance Unit"=w244:u16, "discard cycles"=w243:dbl, "Weigting"=w242:string, "Averaging Time"=w241:dbl, "Max duration"=w240:dbl, "Min duration"=w239:dbl, "Attack Threshold"=w238:dbl, "Hysteresis Up"=w237:dbl, "Fmin(Hz)"=w236:dbl, "Fmax(Hz)"=w235:dbl, "Freq.Resolution"=w234:dbl, "Over-samples Res."=w233:dbl, "Win Resolution"=w232:dbl, "distance"=w231:dbl, "samples"=w230:dbl, "Overlap"=w229:dbl, "Record Length"=w228:dbl, "No.of FFTs"=w227:dbl, "Hz"=w226:dbl, "record delay"=w225:dbl, "Std Err"=w224:dbl, "Response"=w223:bool, "Coherent Power*"=w222:bool, "Stimulus"=w221:bool, "Measurement Confidence"=w220:bool, "Auto Spectrum(Response)*"=w219:bool, "Auto Spectrum(Stimulus)*"=w218:bool, "Cross Spectrum*"=w217:bool, "functions"=w216:bool, "Frequency Response"=w215:bool, "Non-Coherent Power*"=w214:bool, "Coherence (%)"=w213:bool, "Non-Coherence (%)"=w212:bool, "Signal-Noise Ratio (dB)"=w211:bool, "Non-Coherenct Distirtion*"=w210:bool, "Result Waveforms"=w209:bool, "Coupling"=w208:bool, "Averaging"=w207:u16, "Harmonics"=w206:i32, "Custom Curve Names"=w205:i32, "unLabel"=w204:string, "Custom Curve Names"=w203:string, "Unit"=w202:string, "Total IMD + Noise(%)"=w201:bool, "ResponseMe"=w200:u16, "Intermod"=w199:dbl[], "Diff"=w198:dbl[], "Cross-Correlation"=w197:bool, "IM list items"=w196:string[], "Diff list items"=w195:string[], "TSR Window Type"=w192:string)
              n26 = Unbundle(w305) -> ("status"=w306:bool)  [unwired: 2 out]
              n27 = case shown="True" w306 {
                tunnel: w306 -> [_ w308]
                frame False {
                }
                frame True {
                  n28 = local write "Error?"(w308) -> ()
                }
              }
              n29 = Bundle By Name(cluster=w188, "Name"=w302, "Harmonics"=w301, "Algorithm"=w300, "delay"=w299, "THD(%)"=w298, "Rub&Buzz"=w297, "Imp"=w296, "Imp Ref resistor"=w295, "Y data"=w294, "Y prefix"=w293, "Y unit"=w292, "Y dB ref"=w291, "Custom Curve Names"=w290, "har list items"=w289, "Envelope"=w288, "Envelope"=w287, "use custom unit"=w286, "autodelay ch"=w285, "impulse"=w284, "start ms"=w283, "stop ms"=w282, "Scaling"=w281, "Default Overlap"=w280, "Advanced View"=w279, "Loose Particle"=w278, "Use default"=w277, "Auto-Correlation(Stimulus)"=w276, "Auto-Correlation(Response)"=w275, "Deconvolved Response"=w274, "Mic Current"=w273, "M List Vaiues"=w272, "Type"=w271, "Delay Method"=w270, "Apply Correction Out"=w269, "Apply Correction In"=w268, "Harmonics @ meas.frq"=w267, "THD Normalized(%)"=w266, "Total Distortion"=w265, "THD+Noise(%)"=w264, "Rub&Buzz Norm'd(%)"=w263, "Standard Error"=w262, "Confidence Limits"=w261, "Total Diff"=w260, "Total Noise"=w259, "Total DFD(%)"=w258, "Total IMD(%)"=w257, "Total IM"=w256, "Total DFD+Noise(%)"=w255, "Use Channel Name"=w254, "Waveform In"=w253, "Waveform Out"=w252, "Method"=w251, "Spectral Scaling"=w250, "Appliied Unit"=w249, "Length Unit"=w248, "Applied Units"=w247, "Sens Item"=w246, "Tab"=w245, "Distance Unit"=w244, "discard cycles"=w243, "Weigting"=w242, "Averaging Time"=w241, "Max duration"=w240, "Min duration"=w239, "Attack Threshold"=w238, "Hysteresis Up"=w237, "Fmin(Hz)"=w236, "Fmax(Hz)"=w235, "Freq.Resolution"=w234, "Over-samples Res."=w233, "Win Resolution"=w232, "distance"=w231, "samples"=w230, "Overlap"=w229, "Record Length"=w228, "No.of FFTs"=w227, "Hz"=w226, "record delay"=w225, "Std Err"=w224, "Response"=w223, "Coherent Power*"=w222, "Stimulus"=w221, "Measurement Confidence"=w220, "Auto Spectrum(Response)*"=w219, "Auto Spectrum(Stimulus)*"=w218, "Cross Spectrum*"=w217, "functions"=w216, "Frequency Response"=w215, "Non-Coherent Power*"=w214, "Coherence (%)"=w213, "Non-Coherence (%)"=w212, "Signal-Noise Ratio (dB)"=w211, "Non-Coherenct Distirtion*"=w210, "Result Waveforms"=w209, "Coupling"=w208, "Averaging"=w207, "Harmonics"=w206, "Custom Curve Names"=w205, "unLabel"=w204, "Custom Curve Names"=w203, "Unit"=w202, "Total IMD + Noise(%)"=w201, "ResponseMe"=w200, "Intermod"=w199, "Diff"=w198, "Cross-Correlation"=w197, "IM list items"=w196, "Diff list items"=w195, "TSR Window Type"=w192, "Help"="" ("TSR Window Type"), "Imp Auto Mode"=w191, "Mic Auto Mode"=w191, "Curve Resolution"=u16 2, "Curve Resolution Hz"=10.0) -> (w303:T3)
            }
            frame 3 {
              w312 = u16 0 ("Imp Auto Mode")
              n30 = Unflatten From String(type=w315, binary string=w430) -> (value=w427:T9, error out=w428:errorcluster)  [unwired: 1 in, 3 out]
              n31 = Unbundle(w428) -> ("status"=w429:bool)  [unwired: 2 out]
              n32 = case shown="True" w429 {
                tunnel: w429 -> [_ w431]
                frame False {
                }
                frame True {
                  n33 = local write "Error?"(w431) -> ()
                }
              }
              n34 = Unbundle By Name(w427) -> ("Name"=w425:string, "Harmonics"=w424:dbl[], "Algorithm"=w423:u16, "delay"=w422:dbl, "THD(%)"=w421:bool, "Rub&Buzz"=w420:bool, "Imp"=w419:bool, "Ref resistor"=w418:dbl, "Y data"=w417:u16, "Y prefix"=w416:string, "Y unit"=w415:string, "Y dB ref"=w414:dbl, "Custom Curve Names"=w413:string[], "har list items"=w412:string[], "AC/DC"=w411:bool, "Envelope"=w410:bool, "use custom unit"=w409:bool, "autodelay ch"=w408:dbl, "impulse"=w407:bool, "start ms"=w406:dbl, "stop ms"=w405:dbl, "Scaling"=w404:i32, "Default Overlap"=w403:bool, "Advanced View"=w402:bool, "Loose Particle"=w401:bool, "Use default"=w400:bool, "Auto-Correlation(Stimulus)"=w399:bool, "Auto-Correlation(Response)"=w398:bool, "Deconvolved Response"=w397:bool, "DC Connect Measurement"=w396:bool, "M List Vaiues"=w395:u16, "Type"=w394:u16, "Delay Method"=w393:u16, "Apply Correction Out"=w392:bool, "Apply Correction In"=w391:bool, "Harmonics @ meas.frq"=w390:bool, "THD Normalized(%)"=w389:bool, "Total Distortion"=w388:bool, "THD+Noise(%)"=w387:bool, "Rub&Buzz Norm'd(%)"=w386:bool, "Standard Error"=w385:bool, "Confidence Limits"=w384:bool, "Total Diff"=w383:bool, "Total Noise"=w382:bool, "Total DFD(%)"=w381:bool, "Total IMD(%)"=w380:bool, "Total IM"=w379:bool, "Total DFD+Noise(%)"=w378:bool, "Use Channel Name"=w377:bool, "Waveform In"=w376:string, "Waveform Out"=w375:string, "Method"=w374:u16, "Spectral Scaling"=w373:u16, "Appliied Unit"=w372:u16, "Length Unit"=w371:u16, "Applied Units"=w370:u16, "Sens Item"=w369:u16, "Tab"=w368:i32, "Distance Unit"=w367:u16, "discard cycles"=w366:dbl, "Weigting"=w365:string, "Averaging Time"=w364:dbl, "Max duration"=w363:dbl, "Min duration"=w362:dbl, "Attack Threshold"=w361:dbl, "Hysteresis Up"=w360:dbl, "Fmin(Hz)"=w359:dbl, "Fmax(Hz)"=w358:dbl, "Freq.Resolution"=w357:dbl, "Over-samples Res."=w356:dbl, "Win Resolution"=w355:dbl, "distance"=w354:dbl, "samples"=w353:dbl, "Overlap"=w352:dbl, "Record Length"=w351:dbl, "No.of FFTs"=w350:dbl, "Hz"=w349:dbl, "record delay"=w348:dbl, "Std Err"=w347:dbl, "Response"=w346:bool, "Coherent Power*"=w345:bool, "Stimulus"=w344:bool, "Measurement Confidence"=w343:bool, "Auto Spectrum(Response)*"=w342:bool, "Auto Spectrum(Stimulus)*"=w341:bool, "Cross Spectrum*"=w340:bool, "functions"=w339:bool, "Frequency Response"=w338:bool, "Non-Coherent Power*"=w337:bool, "Coherence (%)"=w336:bool, "Non-Coherence (%)"=w335:bool, "Signal-Noise Ratio (dB)"=w334:bool, "Non-Coherenct Distirtion*"=w333:bool, "Result Waveforms"=w332:bool, "Coupling"=w331:bool, "Averaging"=w330:u16, "Harmonics"=w329:i32, "Custom Curve Names"=w328:i32, "unLabel"=w327:string, "Custom Curve Names"=w326:string, "Unit"=w325:string, "Total IMD + Noise(%)"=w324:bool, "ResponseMe"=w323:u16, "Intermod"=w322:dbl[], "Diff"=w321:dbl[], "Cross-Correlation"=w320:bool, "IM list items"=w319:string[], "Diff list items"=w318:string[], "TSR Window Type"=w316:string)
              n35 = Bundle By Name(cluster=w309, "Name"=w425, "Harmonics"=w424, "Algorithm"=w423, "delay"=w422, "THD(%)"=w421, "Rub&Buzz"=w420, "Imp"=w419, "Imp Ref resistor"=w418, "Y data"=w417, "Y prefix"=w416, "Y unit"=w415, "Y dB ref"=w414, "Custom Curve Names"=w413, "har list items"=w412, "Envelope"=w411, "Envelope"=w410, "use custom unit"=w409, "autodelay ch"=w408, "impulse"=w407, "start ms"=w406, "stop ms"=w405, "Scaling"=w404, "Default Overlap"=w403, "Advanced View"=w402, "Loose Particle"=w401, "Use default"=w400, "Auto-Correlation(Stimulus)"=w399, "Auto-Correlation(Response)"=w398, "Deconvolved Response"=w397, "Mic Current"=w396, "M List Vaiues"=w395, "Type"=w394, "Delay Method"=w393, "Apply Correction Out"=w392, "Apply Correction In"=w391, "Harmonics @ meas.frq"=w390, "THD Normalized(%)"=w389, "Total Distortion"=w388, "THD+Noise(%)"=w387, "Rub&Buzz Norm'd(%)"=w386, "Standard Error"=w385, "Confidence Limits"=w384, "Total Diff"=w383, "Total Noise"=w382, "Total DFD(%)"=w381, "Total IMD(%)"=w380, "Total IM"=w379, "Total DFD+Noise(%)"=w378, "Use Channel Name"=w377, "Waveform In"=w376, "Waveform Out"=w375, "Method"=w374, "Spectral Scaling"=w373, "Appliied Unit"=w372, "Length Unit"=w371, "Applied Units"=w370, "Sens Item"=w369, "Tab"=w368, "Distance Unit"=w367, "discard cycles"=w366, "Weigting"=w365, "Averaging Time"=w364, "Max duration"=w363, "Min duration"=w362, "Attack Threshold"=w361, "Hysteresis Up"=w360, "Fmin(Hz)"=w359, "Fmax(Hz)"=w358, "Freq.Resolution"=w357, "Over-samples Res."=w356, "Win Resolution"=w355, "distance"=w354, "samples"=w353, "Overlap"=w352, "Record Length"=w351, "No.of FFTs"=w350, "Hz"=w349, "record delay"=w348, "Std Err"=w347, "Response"=w346, "Coherent Power*"=w345, "Stimulus"=w344, "Measurement Confidence"=w343, "Auto Spectrum(Response)*"=w342, "Auto Spectrum(Stimulus)*"=w341, "Cross Spectrum*"=w340, "functions"=w339, "Frequency Response"=w338, "Non-Coherent Power*"=w337, "Coherence (%)"=w336, "Non-Coherence (%)"=w335, "Signal-Noise Ratio (dB)"=w334, "Non-Coherenct Distirtion*"=w333, "Result Waveforms"=w332, "Coupling"=w331, "Averaging"=w330, "Harmonics"=w329, "Custom Curve Names"=w328, "unLabel"=w327, "Custom Curve Names"=w326, "Unit"=w325, "Total IMD + Noise(%)"=w324, "ResponseMe"=w323, "Intermod"=w322, "Diff"=w321, "Cross-Correlation"=w320, "IM list items"=w319, "Diff list items"=w318, "TSR Window Type"=w316, "Help"="" ("TSR Window Type"), "Custom Curve IDs"=i32[] [], "Default Curve Names"=string[] [], "Imp Auto Mode"=w312, "Mic Auto Mode"=w312, "Curve Resolution"=u16 2, "Curve Resolution Hz"=10.0) -> (w426:T3)
            }
            frame 4 {
              w435 = u16 0 ("Imp Auto Mode")
              n36 = Unflatten From String(type=w442, binary string=w554) -> (value=w551:T8, error out=w552:errorcluster)  [unwired: 1 in, 3 out]
              n37 = Unbundle(w552) -> ("status"=w553:bool)  [unwired: 2 out]
              n38 = case shown="True" w553 {
                tunnel: w553 -> [_ w555]
                frame False {
                }
                frame True {
                  n39 = local write "Error?"(w555) -> ()
                }
              }
              n40 = Unbundle By Name(w551) -> ("Name"=w549:string, "Harmonics"=w548:dbl[], "Algorithm"=w547:u16, "delay"=w546:dbl, "THD(%)"=w545:bool, "Rub&Buzz"=w544:bool, "Imp"=w543:bool, "Ref resistor"=w542:dbl, "Y data"=w541:u16, "Y prefix"=w540:string, "Y unit"=w539:string, "Y dB ref"=w538:dbl, "Custom Curve Names"=w537:string[], "har list items"=w536:string[], "AC/DC"=w535:bool, "Envelope"=w534:bool, "use custom unit"=w533:bool, "autodelay ch"=w532:dbl, "impulse"=w531:bool, "start ms"=w530:dbl, "stop ms"=w529:dbl, "Scaling"=w528:i32, "Default Overlap"=w527:bool, "Advanced View"=w526:bool, "Loose Particle"=w525:bool, "Use default"=w524:bool, "Auto-Correlation(Stimulus)"=w523:bool, "Auto-Correlation(Response)"=w522:bool, "Deconvolved Response"=w521:bool, "DC Connect Measurement"=w437:bool, "M List Vaiues"=w520:u16, "Type"=w519:u16, "Delay Method"=w518:u16, "Apply Correction Out"=w517:bool, "Apply Correction In"=w516:bool, "Harmonics @ meas.frq"=w515:bool, "THD Normalized(%)"=w514:bool, "Total Distortion"=w513:bool, "THD+Noise(%)"=w512:bool, "Rub&Buzz Norm'd(%)"=w511:bool, "Standard Error"=w510:bool, "Confidence Limits"=w509:bool, "Total Diff"=w508:bool, "Total Noise"=w507:bool, "Total DFD(%)"=w506:bool, "Total IMD(%)"=w505:bool, "Total IM"=w504:bool, "Total DFD+Noise(%)"=w503:bool, "Use Channel Name"=w502:bool, "Waveform In"=w501:string, "Waveform Out"=w500:string, "Method"=w499:u16, "Spectral Scaling"=w498:u16, "Appliied Unit"=w497:u16, "Length Unit"=w496:u16, "Applied Units"=w495:u16, "Sens Item"=w494:u16, "Tab"=w493:i32, "Distance Unit"=w492:u16, "discard cycles"=w491:dbl, "Weigting"=w490:string, "Averaging Time"=w489:dbl, "Max duration"=w488:dbl, "Min duration"=w487:dbl, "Attack Threshold"=w486:dbl, "Hysteresis Up"=w485:dbl, "Fmin(Hz)"=w484:dbl, "Fmax(Hz)"=w483:dbl, "Freq.Resolution"=w482:dbl, "Over-samples Res."=w481:dbl, "Win Resolution"=w480:dbl, "distance"=w479:dbl, "samples"=w478:dbl, "Overlap"=w477:dbl, "Record Length"=w476:dbl, "No.of FFTs"=w475:dbl, "Hz"=w474:dbl, "record delay"=w473:dbl, "Std Err"=w472:dbl, "Response"=w471:bool, "Coherent Power*"=w470:bool, "Stimulus"=w469:bool, "Measurement Confidence"=w468:bool, "Auto Spectrum(Response)*"=w467:bool, "Auto Spectrum(Stimulus)*"=w466:bool, "Cross Spectrum*"=w465:bool, "functions"=w464:bool, "Frequency Response"=w463:bool, "Non-Coherent Power*"=w462:bool, "Coherence (%)"=w461:bool, "Non-Coherence (%)"=w460:bool, "Signal-Noise Ratio (dB)"=w459:bool, "Non-Coherenct Distirtion*"=w458:bool, "Result Waveforms"=w457:bool, "Coupling"=w456:bool, "Averaging"=w455:u16, "Harmonics"=w454:i32, "Custom Curve Names"=w436:i32, "unLabel"=w453:string, "Custom Curve Names"=w452:string, "Unit"=w451:string, "Total IMD + Noise(%)"=w450:bool, "ResponseMe"=w449:u16, "Intermod"=w448:dbl[], "Diff"=w447:dbl[], "Cross-Correlation"=w446:bool, "IM list items"=w445:string[], "Diff list items"=w444:string[], "TSR Window Type"=w443:string, "Help"=w441:string, "Custom Curve IDs"=w440:i32[], "Default Curve Names"=w439:string[])
              n41 = Bundle By Name(cluster=w432, "Name"=w549, "Harmonics"=w548, "Algorithm"=w547, "delay"=w546, "THD(%)"=w545, "Rub&Buzz"=w544, "Imp"=w543, "Imp Ref resistor"=w542, "Y data"=w541, "Y prefix"=w540, "Y unit"=w539, "Y dB ref"=w538, "Custom Curve Names"=w537, "har list items"=w536, "Envelope"=w535, "Envelope"=w534, "use custom unit"=w533, "autodelay ch"=w532, "impulse"=w531, "start ms"=w530, "stop ms"=w529, "Scaling"=w528, "Default Overlap"=w527, "Advanced View"=w526, "Loose Particle"=w525, "Use default"=w524, "Auto-Correlation(Stimulus)"=w523, "Auto-Correlation(Response)"=w522, "Deconvolved Response"=w521, "Mic Current"=w437, "M List Vaiues"=w520, "Type"=w519, "Delay Method"=w518, "Apply Correction Out"=w517, "Apply Correction In"=w516, "Harmonics @ meas.frq"=w515, "THD Normalized(%)"=w514, "Total Distortion"=w513, "THD+Noise(%)"=w512, "Rub&Buzz Norm'd(%)"=w511, "Standard Error"=w510, "Confidence Limits"=w509, "Total Diff"=w508, "Total Noise"=w507, "Total DFD(%)"=w506, "Total IMD(%)"=w505, "Total IM"=w504, "Total DFD+Noise(%)"=w503, "Use Channel Name"=w502, "Waveform In"=w501, "Waveform Out"=w500, "Method"=w499, "Spectral Scaling"=w498, "Appliied Unit"=w497, "Length Unit"=w496, "Applied Units"=w495, "Sens Item"=w494, "Tab"=w493, "Distance Unit"=w492, "discard cycles"=w491, "Weigting"=w490, "Averaging Time"=w489, "Max duration"=w488, "Min duration"=w487, "Attack Threshold"=w486, "Hysteresis Up"=w485, "Fmin(Hz)"=w484, "Fmax(Hz)"=w483, "Freq.Resolution"=w482, "Over-samples Res."=w481, "Win Resolution"=w480, "distance"=w479, "samples"=w478, "Overlap"=w477, "Record Length"=w476, "No.of FFTs"=w475, "Hz"=w474, "record delay"=w473, "Std Err"=w472, "Response"=w471, "Coherent Power*"=w470, "Stimulus"=w469, "Measurement Confidence"=w468, "Auto Spectrum(Response)*"=w467, "Auto Spectrum(Stimulus)*"=w466, "Cross Spectrum*"=w465, "functions"=w464, "Frequency Response"=w463, "Non-Coherent Power*"=w462, "Coherence (%)"=w461, "Non-Coherence (%)"=w460, "Signal-Noise Ratio (dB)"=w459, "Non-Coherenct Distirtion*"=w458, "Result Waveforms"=w457, "Coupling"=w456, "Averaging"=w455, "Harmonics"=w454, "Custom Curve Names"=w436, "unLabel"=w453, "Custom Curve Names"=w452, "Unit"=w451, "Total IMD + Noise(%)"=w450, "ResponseMe"=w449, "Intermod"=w448, "Diff"=w447, "Cross-Correlation"=w446, "IM list items"=w445, "Diff list items"=w444, "TSR Window Type"=w443, "Help"=w441, "Custom Curve IDs"=w440, "Default Curve Names"=w439, "Loose Particle waveform"=FALSE, "Imp Auto Mode"=w435, "Mic Auto Mode"=w435, "Curve Resolution"=u16 2, "Curve Resolution Hz"=10.0) -> (w550:T3)
            }
            frame 5 {
              w559 = u16 0 ("Imp Auto Mode")
              n42 = Unflatten From String(type=w562, binary string=w678) -> (value=w675:T11, error out=w676:errorcluster)  [unwired: 1 in, 3 out]
              n43 = Unbundle(w676) -> ("status"=w677:bool)  [unwired: 2 out]
              n44 = case shown="True" w677 {
                tunnel: w677 -> [_ w679]
                frame False {
                }
                frame True {
                  n45 = local write "Error?"(w679) -> ()
                }
              }
              n46 = Unbundle By Name(w675) -> ("Name"=w673:string, "Harmonics"=w672:dbl[], "Algorithm"=w671:u16, "delay"=w670:dbl, "THD(%)"=w669:bool, "Rub&Buzz"=w668:bool, "Imp"=w667:bool, "Ref resistor"=w666:dbl, "Y data"=w665:u16, "Y prefix"=w664:string, "Y unit"=w663:string, "Y dB ref"=w662:dbl, "Custom Curve Names"=w661:string[], "har list items"=w660:string[], "AC/DC"=w659:bool, "Envelope"=w658:bool, "use custom unit"=w657:bool, "autodelay ch"=w656:dbl, "impulse"=w655:bool, "start ms"=w654:dbl, "stop ms"=w653:dbl, "Scaling"=w652:i32, "Default Overlap"=w651:bool, "Advanced View"=w650:bool, "Loose Particle"=w649:bool, "Use default"=w648:bool, "Auto-Correlation(Stimulus)"=w647:bool, "Auto-Correlation(Response)"=w646:bool, "Deconvolved Response"=w645:bool, "DC Connect Measurement"=w560:bool, "M List Vaiues"=w644:u16, "Type"=w643:u16, "Delay Method"=w642:u16, "Apply Correction Out"=w641:bool, "Apply Correction In"=w640:bool, "Harmonics @ meas.frq"=w639:bool, "THD Normalized(%)"=w638:bool, "Total Distortion"=w637:bool, "THD+Noise(%)"=w636:bool, "Rub&Buzz Norm'd(%)"=w635:bool, "Standard Error"=w634:bool, "Confidence Limits"=w633:bool, "Total Diff"=w632:bool, "Total Noise"=w631:bool, "Total DFD(%)"=w630:bool, "Total IMD(%)"=w629:bool, "Total IM"=w628:bool, "Total DFD+Noise(%)"=w627:bool, "Use Channel Name"=w626:bool, "Waveform In"=w625:string, "Waveform Out"=w624:string, "Method"=w623:u16, "Spectral Scaling"=w622:u16, "Appliied Unit"=w621:u16, "Length Unit"=w620:u16, "Applied Units"=w619:u16, "Sens Item"=w618:u16, "Tab"=w617:i32, "Distance Unit"=w616:u16, "discard cycles"=w615:dbl, "Weigting"=w614:string, "Averaging Time"=w613:dbl, "Max duration"=w612:dbl, "Min duration"=w611:dbl, "Attack Threshold"=w610:dbl, "Hysteresis Up"=w609:dbl, "Fmin(Hz)"=w608:dbl, "Fmax(Hz)"=w607:dbl, "Freq.Resolution"=w606:dbl, "Over-samples Res."=w605:dbl, "Win Resolution"=w604:dbl, "distance"=w603:dbl, "samples"=w602:dbl, "Overlap"=w601:dbl, "Record Length"=w600:dbl, "No.of FFTs"=w599:dbl, "Hz"=w598:dbl, "record delay"=w597:dbl, "Std Err"=w596:dbl, "Response"=w595:bool, "Coherent Power*"=w594:bool, "Stimulus"=w593:bool, "Measurement Confidence"=w592:bool, "Auto Spectrum(Response)*"=w591:bool, "Auto Spectrum(Stimulus)*"=w590:bool, "Cross Spectrum*"=w589:bool, "functions"=w588:bool, "Frequency Response"=w587:bool, "Non-Coherent Power*"=w586:bool, "Coherence (%)"=w585:bool, "Non-Coherence (%)"=w584:bool, "Signal-Noise Ratio (dB)"=w583:bool, "Non-Coherenct Distirtion*"=w582:bool, "Result Waveforms"=w581:bool, "Coupling"=w580:bool, "Averaging"=w579:u16, "Harmonics"=w578:i32, "Custom Curve Names"=w577:i32, "unLabel"=w576:string, "Custom Curve Names"=w575:string, "Unit"=w574:string, "Total IMD + Noise(%)"=w573:bool, "ResponseMe"=w572:u16, "Intermod"=w571:dbl[], "Diff"=w570:dbl[], "Cross-Correlation"=w569:bool, "IM list items"=w568:string[], "Diff list items"=w567:string[], "TSR Window Type"=w566:string, "Help"=w565:string, "Custom Curve IDs"=w564:i32[], "Default Curve Names"=w563:string[], "Loose Particle waveform"=w561:bool)
              n47 = Bundle By Name(cluster=w556, "Name"=w673, "Harmonics"=w672, "Algorithm"=w671, "delay"=w670, "THD(%)"=w669, "Rub&Buzz"=w668, "Imp"=w667, "Imp Ref resistor"=w666, "Y data"=w665, "Y prefix"=w664, "Y unit"=w663, "Y dB ref"=w662, "Custom Curve Names"=w661, "har list items"=w660, "Envelope"=w659, "Envelope"=w658, "use custom unit"=w657, "autodelay ch"=w656, "impulse"=w655, "start ms"=w654, "stop ms"=w653, "Scaling"=w652, "Default Overlap"=w651, "Advanced View"=w650, "Loose Particle"=w649, "Use default"=w648, "Auto-Correlation(Stimulus)"=w647, "Auto-Correlation(Response)"=w646, "Deconvolved Response"=w645, "Mic Current"=w560, "M List Vaiues"=w644, "Type"=w643, "Delay Method"=w642, "Apply Correction Out"=w641, "Apply Correction In"=w640, "Harmonics @ meas.frq"=w639, "THD Normalized(%)"=w638, "Total Distortion"=w637, "THD+Noise(%)"=w636, "Rub&Buzz Norm'd(%)"=w635, "Standard Error"=w634, "Confidence Limits"=w633, "Total Diff"=w632, "Total Noise"=w631, "Total DFD(%)"=w630, "Total IMD(%)"=w629, "Total IM"=w628, "Total DFD+Noise(%)"=w627, "Use Channel Name"=w626, "Waveform In"=w625, "Waveform Out"=w624, "Method"=w623, "Spectral Scaling"=w622, "Appliied Unit"=w621, "Length Unit"=w620, "Applied Units"=w619, "Sens Item"=w618, "Tab"=w617, "Distance Unit"=w616, "discard cycles"=w615, "Weigting"=w614, "Averaging Time"=w613, "Max duration"=w612, "Min duration"=w611, "Attack Threshold"=w610, "Hysteresis Up"=w609, "Fmin(Hz)"=w608, "Fmax(Hz)"=w607, "Freq.Resolution"=w606, "Over-samples Res."=w605, "Win Resolution"=w604, "distance"=w603, "samples"=w602, "Overlap"=w601, "Record Length"=w600, "No.of FFTs"=w599, "Hz"=w598, "record delay"=w597, "Std Err"=w596, "Response"=w595, "Coherent Power*"=w594, "Stimulus"=w593, "Measurement Confidence"=w592, "Auto Spectrum(Response)*"=w591, "Auto Spectrum(Stimulus)*"=w590, "Cross Spectrum*"=w589, "functions"=w588, "Frequency Response"=w587, "Non-Coherent Power*"=w586, "Coherence (%)"=w585, "Non-Coherence (%)"=w584, "Signal-Noise Ratio (dB)"=w583, "Non-Coherenct Distirtion*"=w582, "Result Waveforms"=w581, "Coupling"=w580, "Averaging"=w579, "Harmonics"=w578, "Custom Curve Names"=w577, "unLabel"=w576, "Custom Curve Names"=w575, "Unit"=w574, "Total IMD + Noise(%)"=w573, "ResponseMe"=w572, "Intermod"=w571, "Diff"=w570, "Cross-Correlation"=w569, "IM list items"=w568, "Diff list items"=w567, "TSR Window Type"=w566, "Help"=w565, "Custom Curve IDs"=w564, "Default Curve Names"=w563, "Loose Particle waveform"=w561, "Imp Auto Mode"=w559, "Mic Auto Mode"=w559, "Curve Resolution"=u16 2, "Curve Resolution Hz"=10.0) -> (w674:T3)
            }
            frame 6 {
              w683 = u16 0 ("Imp Auto Mode")
              n48 = Unflatten From String(type=w684, binary string=w802) -> (value=w799:T7, error out=w800:errorcluster)  [unwired: 1 in, 3 out]
              n49 = Unbundle(w800) -> ("status"=w801:bool)  [unwired: 2 out]
              n50 = case shown="True" w801 {
                tunnel: w801 -> [_ w803]
                frame False {
                }
                frame True {
                  n51 = local write "Error?"(w803) -> ()
                }
              }
              n52 = Unbundle By Name(w799) -> ("Name"=w797:string, "Harmonics"=w796:dbl[], "Algorithm"=w795:u16, "delay"=w794:dbl, "THD(%)"=w793:bool, "Rub&Buzz"=w792:bool, "Imp"=w791:bool, "Ref resistor"=w790:dbl, "Y data"=w789:u16, "Y prefix"=w788:string, "Y unit"=w787:string, "Y dB ref"=w786:dbl, "Custom Curve Names"=w785:string[], "har list items"=w784:string[], "AC/DC"=w783:bool, "Envelope"=w782:bool, "use custom unit"=w781:bool, "autodelay ch"=w780:dbl, "impulse"=w779:bool, "start ms"=w778:dbl, "stop ms"=w777:dbl, "Scaling"=w776:i32, "Default Overlap"=w775:bool, "Advanced View"=w774:bool, "Loose Particle"=w773:bool, "Use default"=w772:bool, "Auto-Correlation(Stimulus)"=w771:bool, "Auto-Correlation(Response)"=w770:bool, "Deconvolved Response"=w769:bool, "DC Connect Measurement"=w685:bool, "M List Vaiues"=w768:u16, "Type"=w767:u16, "Delay Method"=w766:u16, "Apply Correction Out"=w765:bool, "Apply Correction In"=w764:bool, "Harmonics @ meas.frq"=w763:bool, "THD Normalized(%)"=w762:bool, "Total Distortion"=w761:bool, "THD+Noise(%)"=w760:bool, "Rub&Buzz Norm'd(%)"=w759:bool, "Standard Error"=w758:bool, "Confidence Limits"=w757:bool, "Total Diff"=w756:bool, "Total Noise"=w755:bool, "Total DFD(%)"=w754:bool, "Total IMD(%)"=w753:bool, "Total IM"=w752:bool, "Total DFD+Noise(%)"=w751:bool, "Use Channel Name"=w750:bool, "Waveform In"=w749:string, "Waveform Out"=w748:string, "Method"=w747:u16, "Spectral Scaling"=w746:u16, "Appliied Unit"=w745:u16, "Length Unit"=w744:u16, "Applied Units"=w743:u16, "Sens Item"=w742:u16, "Tab"=w741:i32, "Distance Unit"=w740:u16, "discard cycles"=w739:dbl, "Weigting"=w738:string, "Averaging Time"=w737:dbl, "Max duration"=w736:dbl, "Min duration"=w735:dbl, "Attack Threshold"=w734:dbl, "Hysteresis Up"=w733:dbl, "Fmin(Hz)"=w732:dbl, "Fmax(Hz)"=w731:dbl, "Freq.Resolution"=w730:dbl, "Over-samples Res."=w729:dbl, "Win Resolution"=w728:dbl, "distance"=w727:dbl, "samples"=w726:dbl, "Overlap"=w725:dbl, "Record Length"=w724:dbl, "No.of FFTs"=w723:dbl, "Hz"=w722:dbl, "record delay"=w721:dbl, "Std Err"=w720:dbl, "Response"=w719:bool, "Coherent Power*"=w718:bool, "Stimulus"=w717:bool, "Measurement Confidence"=w716:bool, "Auto Spectrum(Response)*"=w715:bool, "Auto Spectrum(Stimulus)*"=w714:bool, "Cross Spectrum*"=w713:bool, "functions"=w712:bool, "Frequency Response"=w711:bool, "Non-Coherent Power*"=w710:bool, "Coherence (%)"=w709:bool, "Non-Coherence (%)"=w708:bool, "Signal-Noise Ratio (dB)"=w707:bool, "Non-Coherenct Distirtion*"=w706:bool, "Result Waveforms"=w705:bool, "Coupling"=w704:bool, "Averaging"=w703:u16, "Harmonics"=w702:i32, "Custom Curve Names"=w701:i32, "unLabel"=w700:string, "Custom Curve Names"=w699:string, "Unit"=w698:string, "Total IMD + Noise(%)"=w697:bool, "ResponseMe"=w696:u16, "Intermod"=w695:dbl[], "Diff"=w694:dbl[], "Cross-Correlation"=w693:bool, "IM list items"=w692:string[], "Diff list items"=w691:string[], "TSR Window Type"=w690:string, "Help"=w689:string, "Custom Curve IDs"=w688:i32[], "Default Curve Names"=w687:string[], "Loose Particle waveform"=w686:bool)
              n53 = Bundle By Name(cluster=w680, "Name"=w797, "Harmonics"=w796, "Algorithm"=w795, "delay"=w794, "THD(%)"=w793, "Rub&Buzz"=w792, "Imp"=w791, "Imp Ref resistor"=w790, "Y data"=w789, "Y prefix"=w788, "Y unit"=w787, "Y dB ref"=w786, "Custom Curve Names"=w785, "har list items"=w784, "Envelope"=w783, "Envelope"=w782, "use custom unit"=w781, "autodelay ch"=w780, "impulse"=w779, "start ms"=w778, "stop ms"=w777, "Scaling"=w776, "Default Overlap"=w775, "Advanced View"=w774, "Loose Particle"=w773, "Use default"=w772, "Auto-Correlation(Stimulus)"=w771, "Auto-Correlation(Response)"=w770, "Deconvolved Response"=w769, "Mic Current"=w685, "M List Vaiues"=w768, "Type"=w767, "Delay Method"=w766, "Apply Correction Out"=w765, "Apply Correction In"=w764, "Harmonics @ meas.frq"=w763, "THD Normalized(%)"=w762, "Total Distortion"=w761, "THD+Noise(%)"=w760, "Rub&Buzz Norm'd(%)"=w759, "Standard Error"=w758, "Confidence Limits"=w757, "Total Diff"=w756, "Total Noise"=w755, "Total DFD(%)"=w754, "Total IMD(%)"=w753, "Total IM"=w752, "Total DFD+Noise(%)"=w751, "Use Channel Name"=w750, "Waveform In"=w749, "Waveform Out"=w748, "Method"=w747, "Spectral Scaling"=w746, "Appliied Unit"=w745, "Length Unit"=w744, "Applied Units"=w743, "Sens Item"=w742, "Tab"=w741, "Distance Unit"=w740, "discard cycles"=w739, "Weigting"=w738, "Averaging Time"=w737, "Max duration"=w736, "Min duration"=w735, "Attack Threshold"=w734, "Hysteresis Up"=w733, "Fmin(Hz)"=w732, "Fmax(Hz)"=w731, "Freq.Resolution"=w730, "Over-samples Res."=w729, "Win Resolution"=w728, "distance"=w727, "samples"=w726, "Overlap"=w725, "Record Length"=w724, "No.of FFTs"=w723, "Hz"=w722, "record delay"=w721, "Std Err"=w720, "Response"=w719, "Coherent Power*"=w718, "Stimulus"=w717, "Measurement Confidence"=w716, "Auto Spectrum(Response)*"=w715, "Auto Spectrum(Stimulus)*"=w714, "Cross Spectrum*"=w713, "functions"=w712, "Frequency Response"=w711, "Non-Coherent Power*"=w710, "Coherence (%)"=w709, "Non-Coherence (%)"=w708, "Signal-Noise Ratio (dB)"=w707, "Non-Coherenct Distirtion*"=w706, "Result Waveforms"=w705, "Coupling"=w704, "Averaging"=w703, "Harmonics"=w702, "Custom Curve Names"=w701, "unLabel"=w700, "Custom Curve Names"=w699, "Unit"=w698, "Total IMD + Noise(%)"=w697, "ResponseMe"=w696, "Intermod"=w695, "Diff"=w694, "Cross-Correlation"=w693, "IM list items"=w692, "Diff list items"=w691, "TSR Window Type"=w690, "Help"=w689, "Custom Curve IDs"=w688, "Default Curve Names"=w687, "Loose Particle waveform"=w686, "Imp Auto Mode"=w683, "Mic Auto Mode"=w683, "Curve Resolution"=u16 2, "Curve Resolution Hz"=10.0) -> (w798:T3)
            }
            frame 7 {
              n54 = Unflatten From String(type=w812, binary string=w927) -> (value=w924:T6, error out=w925:errorcluster)  [unwired: 1 in, 3 out]
              n55 = Unbundle(w925) -> ("status"=w926:bool)  [unwired: 2 out]
              n56 = case shown="True" w926 {
                tunnel: w926 -> [_ w928]
                frame False {
                }
                frame True {
                  n57 = local write "Error?"(w928) -> ()
                }
              }
              n58 = Unbundle By Name(w924) -> ("Name"=w922:string, "Harmonics"=w921:dbl[], "Algorithm"=w920:u16, "delay"=w919:dbl, "THD(%)"=w918:bool, "Rub&Buzz"=w917:bool, "Imp"=w916:bool, "Ref resistor"=w915:dbl, "Y data"=w914:u16, "Y prefix"=w913:string, "Y unit"=w912:string, "Y dB ref"=w911:dbl, "Custom Curve Names"=w910:string[], "har list items"=w909:string[], "Envelope"=w908:bool, "Envelope"=w907:bool, "use custom unit"=w906:bool, "autodelay ch"=w905:dbl, "impulse"=w904:bool, "start ms"=w903:dbl, "stop ms"=w902:dbl, "Scaling"=w901:i32, "Default Overlap"=w900:bool, "Advanced View"=w899:bool, "Loose Particle"=w898:bool, "Use default"=w897:bool, "Auto-Correlation(Stimulus)"=w896:bool, "Auto-Correlation(Response)"=w895:bool, "Deconvolved Response"=w894:bool, "Mic Current"=w813:bool, "M List Vaiues"=w893:u16, "Type"=w892:u16, "Delay Method"=w891:u16, "Apply Correction Out"=w890:bool, "Apply Correction In"=w889:bool, "Harmonics @ meas.frq"=w888:bool, "THD Normalized(%)"=w887:bool, "Total Distortion"=w886:bool, "THD+Noise(%)"=w885:bool, "Rub&Buzz Norm'd(%)"=w884:bool, "Standard Error"=w883:bool, "Confidence Limits"=w882:bool, "Total Diff"=w881:bool, "Total Noise"=w880:bool, "Total DFD(%)"=w879:bool, "Total IMD(%)"=w878:bool, "Total IM"=w877:bool, "Total DFD+Noise(%)"=w876:bool, "Use Channel Name"=w875:bool, "Waveform In"=w874:string, "Waveform Out"=w873:string, "Method"=w872:u16, "Spectral Scaling"=w871:u16, "Appliied Unit"=w870:u16, "Length Unit"=w869:u16, "Applied Units"=w868:u16, "Sens Item"=w867:u16, "Tab"=w866:i32, "Distance Unit"=w865:u16, "discard cycles"=w864:dbl, "Weigting"=w863:string, "Averaging Time"=w862:dbl, "Max duration"=w861:dbl, "Min duration"=w860:dbl, "Attack Threshold"=w859:dbl, "Hysteresis Up"=w858:dbl, "Fmin(Hz)"=w857:dbl, "Fmax(Hz)"=w856:dbl, "Freq.Resolution"=w855:dbl, "Over-samples Res."=w854:dbl, "Win Resolution"=w853:dbl, "distance"=w852:dbl, "samples"=w851:dbl, "Overlap"=w850:dbl, "Record Length"=w849:dbl, "No.of FFTs"=w848:dbl, "Hz"=w847:dbl, "record delay"=w846:dbl, "Std Err"=w845:dbl, "Response"=w844:bool, "Coherent Power*"=w843:bool, "Stimulus"=w842:bool, "Measurement Confidence"=w841:bool, "Auto Spectrum(Response)*"=w840:bool, "Auto Spectrum(Stimulus)*"=w839:bool, "Cross Spectrum*"=w838:bool, "functions"=w837:bool, "Frequency Response"=w836:bool, "Non-Coherent Power*"=w835:bool, "Coherence (%)"=w834:bool, "Non-Coherence (%)"=w833:bool, "Signal-Noise Ratio (dB)"=w832:bool, "Non-Coherenct Distirtion*"=w831:bool, "Result Waveforms"=w830:bool, "Coupling"=w829:bool, "Averaging"=w828:u16, "Harmonics"=w809:i32, "Custom Curve Names"=w808:i32, "unLabel"=w827:string, "Custom Curve Names"=w807:string, "Unit"=w826:string, "Total IMD + Noise(%)"=w825:bool, "ResponseMe"=w824:u16, "Intermod"=w823:dbl[], "Diff"=w822:dbl[], "Cross-Correlation"=w821:bool, "IM list items"=w820:string[], "Diff list items"=w819:string[], "TSR Window Type"=w818:string, "Help"=w817:string, "Custom Curve IDs"=w816:i32[], "Default Curve Names"=w815:string[], "Loose Particle waveform"=w814:bool, "Imp Auto Mode"=w811:u16)
              n59 = Bundle By Name(cluster=w804, "Name"=w922, "Harmonics"=w921, "Algorithm"=w920, "delay"=w919, "THD(%)"=w918, "Rub&Buzz"=w917, "Imp"=w916, "Imp Ref resistor"=w915, "Y data"=w914, "Y prefix"=w913, "Y unit"=w912, "Y dB ref"=w911, "Custom Curve Names"=w910, "har list items"=w909, "Envelope"=w908, "Envelope"=w907, "use custom unit"=w906, "autodelay ch"=w905, "impulse"=w904, "start ms"=w903, "stop ms"=w902, "Scaling"=w901, "Default Overlap"=w900, "Advanced View"=w899, "Loose Particle"=w898, "Use default"=w897, "Auto-Correlation(Stimulus)"=w896, "Auto-Correlation(Response)"=w895, "Deconvolved Response"=w894, "Mic Current"=w813, "M List Vaiues"=w893, "Type"=w892, "Delay Method"=w891, "Apply Correction Out"=w890, "Apply Correction In"=w889, "Harmonics @ meas.frq"=w888, "THD Normalized(%)"=w887, "Total Distortion"=w886, "THD+Noise(%)"=w885, "Rub&Buzz Norm'd(%)"=w884, "Standard Error"=w883, "Confidence Limits"=w882, "Total Diff"=w881, "Total Noise"=w880, "Total DFD(%)"=w879, "Total IMD(%)"=w878, "Total IM"=w877, "Total DFD+Noise(%)"=w876, "Use Channel Name"=w875, "Waveform In"=w874, "Waveform Out"=w873, "Method"=w872, "Spectral Scaling"=w871, "Appliied Unit"=w870, "Length Unit"=w869, "Applied Units"=w868, "Sens Item"=w867, "Tab"=w866, "Distance Unit"=w865, "discard cycles"=w864, "Weigting"=w863, "Averaging Time"=w862, "Max duration"=w861, "Min duration"=w860, "Attack Threshold"=w859, "Hysteresis Up"=w858, "Fmin(Hz)"=w857, "Fmax(Hz)"=w856, "Freq.Resolution"=w855, "Over-samples Res."=w854, "Win Resolution"=w853, "distance"=w852, "samples"=w851, "Overlap"=w850, "Record Length"=w849, "No.of FFTs"=w848, "Hz"=w847, "record delay"=w846, "Std Err"=w845, "Response"=w844, "Coherent Power*"=w843, "Stimulus"=w842, "Measurement Confidence"=w841, "Auto Spectrum(Response)*"=w840, "Auto Spectrum(Stimulus)*"=w839, "Cross Spectrum*"=w838, "functions"=w837, "Frequency Response"=w836, "Non-Coherent Power*"=w835, "Coherence (%)"=w834, "Non-Coherence (%)"=w833, "Signal-Noise Ratio (dB)"=w832, "Non-Coherenct Distirtion*"=w831, "Result Waveforms"=w830, "Coupling"=w829, "Averaging"=w828, "Harmonics"=w809, "Custom Curve Names"=w808, "unLabel"=w827, "Custom Curve Names"=w807, "Unit"=w826, "Total IMD + Noise(%)"=w825, "ResponseMe"=w824, "Intermod"=w823, "Diff"=w822, "Cross-Correlation"=w821, "IM list items"=w820, "Diff list items"=w819, "TSR Window Type"=w818, "Help"=w817, "Custom Curve IDs"=w816, "Default Curve Names"=w815, "Loose Particle waveform"=w814, "Imp Auto Mode"=w811, "Mic Auto Mode"=u16 0, "Curve Resolution"=u16 2, "Curve Resolution Hz"=10.0) -> (w923:T3)
            }
            frame 8 {
              n60 = Unflatten From String(type=w937, binary string=w1052) -> (value=w1049:T6, error out=w1050:errorcluster)  [unwired: 1 in, 3 out]
              n61 = Unbundle(w1050) -> ("status"=w1051:bool)  [unwired: 2 out]
              n62 = case shown="True" w1051 {
                tunnel: w1051 -> [_ w1053]
                frame False {
                }
                frame True {
                  n63 = local write "Error?"(w1053) -> ()
                }
              }
              n64 = Unbundle By Name(w1049) -> ("Name"=w1047:string, "Harmonics"=w1046:dbl[], "Algorithm"=w1045:u16, "delay"=w1044:dbl, "THD(%)"=w1043:bool, "Rub&Buzz"=w1042:bool, "Imp"=w1041:bool, "Ref resistor"=w1040:dbl, "Y data"=w1039:u16, "Y prefix"=w1038:string, "Y unit"=w1037:string, "Y dB ref"=w1036:dbl, "Custom Curve Names"=w1035:string[], "har list items"=w1034:string[], "Envelope"=w1033:bool, "Envelope"=w1032:bool, "use custom unit"=w1031:bool, "autodelay ch"=w1030:dbl, "impulse"=w1029:bool, "start ms"=w1028:dbl, "stop ms"=w1027:dbl, "Scaling"=w1026:i32, "Default Overlap"=w1025:bool, "Advanced View"=w1024:bool, "Loose Particle"=w1023:bool, "Use default"=w1022:bool, "Auto-Correlation(Stimulus)"=w1021:bool, "Auto-Correlation(Response)"=w1020:bool, "Deconvolved Response"=w1019:bool, "Mic Current"=w938:bool, "M List Vaiues"=w1018:u16, "Type"=w1017:u16, "Delay Method"=w1016:u16, "Apply Correction Out"=w1015:bool, "Apply Correction In"=w1014:bool, "Harmonics @ meas.frq"=w1013:bool, "THD Normalized(%)"=w1012:bool, "Total Distortion"=w1011:bool, "THD+Noise(%)"=w1010:bool, "Rub&Buzz Norm'd(%)"=w1009:bool, "Standard Error"=w1008:bool, "Confidence Limits"=w1007:bool, "Total Diff"=w1006:bool, "Total Noise"=w1005:bool, "Total DFD(%)"=w1004:bool, "Total IMD(%)"=w1003:bool, "Total IM"=w1002:bool, "Total DFD+Noise(%)"=w1001:bool, "Use Channel Name"=w1000:bool, "Waveform In"=w999:string, "Waveform Out"=w998:string, "Method"=w997:u16, "Spectral Scaling"=w996:u16, "Appliied Unit"=w995:u16, "Length Unit"=w994:u16, "Applied Units"=w993:u16, "Sens Item"=w992:u16, "Tab"=w991:i32, "Distance Unit"=w990:u16, "discard cycles"=w989:dbl, "Weigting"=w988:string, "Averaging Time"=w987:dbl, "Max duration"=w986:dbl, "Min duration"=w985:dbl, "Attack Threshold"=w984:dbl, "Hysteresis Up"=w983:dbl, "Fmin(Hz)"=w982:dbl, "Fmax(Hz)"=w981:dbl, "Freq.Resolution"=w980:dbl, "Over-samples Res."=w979:dbl, "Win Resolution"=w978:dbl, "distance"=w977:dbl, "samples"=w976:dbl, "Overlap"=w975:dbl, "Record Length"=w974:dbl, "No.of FFTs"=w973:dbl, "Hz"=w972:dbl, "record delay"=w971:dbl, "Std Err"=w970:dbl, "Response"=w969:bool, "Coherent Power*"=w968:bool, "Stimulus"=w967:bool, "Measurement Confidence"=w966:bool, "Auto Spectrum(Response)*"=w965:bool, "Auto Spectrum(Stimulus)*"=w964:bool, "Cross Spectrum*"=w963:bool, "functions"=w962:bool, "Frequency Response"=w961:bool, "Non-Coherent Power*"=w960:bool, "Coherence (%)"=w959:bool, "Non-Coherence (%)"=w958:bool, "Signal-Noise Ratio (dB)"=w957:bool, "Non-Coherenct Distirtion*"=w956:bool, "Result Waveforms"=w955:bool, "Coupling"=w954:bool, "Averaging"=w953:u16, "Harmonics"=w934:i32, "Custom Curve Names"=w933:i32, "unLabel"=w952:string, "Custom Curve Names"=w932:string, "Unit"=w951:string, "Total IMD + Noise(%)"=w950:bool, "ResponseMe"=w949:u16, "Intermod"=w948:dbl[], "Diff"=w947:dbl[], "Cross-Correlation"=w946:bool, "IM list items"=w945:string[], "Diff list items"=w944:string[], "TSR Window Type"=w943:string, "Help"=w942:string, "Custom Curve IDs"=w941:i32[], "Default Curve Names"=w940:string[], "Loose Particle waveform"=w939:bool, "Imp Auto Mode"=w936:u16)
              n65 = Bundle By Name(cluster=w929, "Name"=w1047, "Harmonics"=w1046, "Algorithm"=w1045, "delay"=w1044, "THD(%)"=w1043, "Rub&Buzz"=w1042, "Imp"=w1041, "Imp Ref resistor"=w1040, "Y data"=w1039, "Y prefix"=w1038, "Y unit"=w1037, "Y dB ref"=w1036, "Custom Curve Names"=w1035, "har list items"=w1034, "Envelope"=w1033, "Envelope"=w1032, "use custom unit"=w1031, "autodelay ch"=w1030, "impulse"=w1029, "start ms"=w1028, "stop ms"=w1027, "Scaling"=w1026, "Default Overlap"=w1025, "Advanced View"=w1024, "Loose Particle"=w1023, "Use default"=w1022, "Auto-Correlation(Stimulus)"=w1021, "Auto-Correlation(Response)"=w1020, "Deconvolved Response"=w1019, "Mic Current"=w938, "M List Vaiues"=w1018, "Type"=w1017, "Delay Method"=w1016, "Apply Correction Out"=w1015, "Apply Correction In"=w1014, "Harmonics @ meas.frq"=w1013, "THD Normalized(%)"=w1012, "Total Distortion"=w1011, "THD+Noise(%)"=w1010, "Rub&Buzz Norm'd(%)"=w1009, "Standard Error"=w1008, "Confidence Limits"=w1007, "Total Diff"=w1006, "Total Noise"=w1005, "Total DFD(%)"=w1004, "Total IMD(%)"=w1003, "Total IM"=w1002, "Total DFD+Noise(%)"=w1001, "Use Channel Name"=w1000, "Waveform In"=w999, "Waveform Out"=w998, "Method"=w997, "Spectral Scaling"=w996, "Appliied Unit"=w995, "Length Unit"=w994, "Applied Units"=w993, "Sens Item"=w992, "Tab"=w991, "Distance Unit"=w990, "discard cycles"=w989, "Weigting"=w988, "Averaging Time"=w987, "Max duration"=w986, "Min duration"=w985, "Attack Threshold"=w984, "Hysteresis Up"=w983, "Fmin(Hz)"=w982, "Fmax(Hz)"=w981, "Freq.Resolution"=w980, "Over-samples Res."=w979, "Win Resolution"=w978, "distance"=w977, "samples"=w976, "Overlap"=w975, "Record Length"=w974, "No.of FFTs"=w973, "Hz"=w972, "record delay"=w971, "Std Err"=w970, "Response"=w969, "Coherent Power*"=w968, "Stimulus"=w967, "Measurement Confidence"=w966, "Auto Spectrum(Response)*"=w965, "Auto Spectrum(Stimulus)*"=w964, "Cross Spectrum*"=w963, "functions"=w962, "Frequency Response"=w961, "Non-Coherent Power*"=w960, "Coherence (%)"=w959, "Non-Coherence (%)"=w958, "Signal-Noise Ratio (dB)"=w957, "Non-Coherenct Distirtion*"=w956, "Result Waveforms"=w955, "Coupling"=w954, "Averaging"=w953, "Harmonics"=w934, "Custom Curve Names"=w933, "unLabel"=w952, "Custom Curve Names"=w932, "Unit"=w951, "Total IMD + Noise(%)"=w950, "ResponseMe"=w949, "Intermod"=w948, "Diff"=w947, "Cross-Correlation"=w946, "IM list items"=w945, "Diff list items"=w944, "TSR Window Type"=w943, "Help"=w942, "Custom Curve IDs"=w941, "Default Curve Names"=w940, "Loose Particle waveform"=w939, "Imp Auto Mode"=w936, "Mic Auto Mode"=u16 0, "Curve Resolution"=u16 2, "Curve Resolution Hz"=10.0) -> (w1048:T3)
            }
            frame 9 {
              n66 = Unflatten From String(type=w1055, binary string=w1178) -> (value=w1175:T4, error out=w1176:errorcluster)  [unwired: 1 in, 3 out]
              n67 = Unbundle(w1176) -> ("status"=w1177:bool)  [unwired: 2 out]
              n68 = case shown="True" w1177 {
                tunnel: w1177 -> [_ w1179]
                frame False {
                }
                frame True {
                  n69 = local write "Error?"(w1179) -> ()
                }
              }
              n70 = Unbundle By Name(w1175) -> ("Name"=w1173:string, "Harmonics"=w1172:dbl[], "Algorithm"=w1171:u16, "delay"=w1170:dbl, "THD(%)"=w1169:bool, "Rub&Buzz"=w1168:bool, "Imp"=w1167:bool, "Imp Ref resistor"=w1166:dbl, "Y data"=w1165:u16, "Y prefix"=w1164:string, "Y unit"=w1163:string, "Y dB ref"=w1162:dbl, "Custom Curve Names"=w1161:string[], "har list items"=w1160:string[], "Envelope"=w1159:bool, "Envelope"=w1158:bool, "use custom unit"=w1157:bool, "autodelay ch"=w1156:dbl, "impulse"=w1155:bool, "start ms"=w1154:dbl, "stop ms"=w1153:dbl, "Scaling"=w1152:i32, "Default Overlap"=w1151:bool, "Advanced View"=w1150:bool, "Loose Particle"=w1149:bool, "Use default"=w1148:bool, "Auto-Correlation(Stimulus)"=w1147:bool, "Auto-Correlation(Response)"=w1146:bool, "Deconvolved Response"=w1145:bool, "Mic Current"=w1064:bool, "M List Vaiues"=w1144:u16, "Type"=w1143:u16, "Delay Method"=w1142:u16, "Apply Correction Out"=w1141:bool, "Apply Correction In"=w1140:bool, "Harmonics @ meas.frq"=w1139:bool, "THD Normalized(%)"=w1138:bool, "Total Distortion"=w1137:bool, "THD+Noise(%)"=w1136:bool, "Rub&Buzz Norm'd(%)"=w1135:bool, "Standard Error"=w1134:bool, "Confidence Limits"=w1133:bool, "Total Diff"=w1132:bool, "Total Noise"=w1131:bool, "Total DFD(%)"=w1130:bool, "Total IMD(%)"=w1129:bool, "Total IM"=w1128:bool, "Total DFD+Noise(%)"=w1127:bool, "Use Channel Name"=w1126:bool, "Waveform In"=w1125:string, "Waveform Out"=w1124:string, "Method"=w1123:u16, "Spectral Scaling"=w1122:u16, "Appliied Unit"=w1121:u16, "Length Unit"=w1120:u16, "Applied Units"=w1119:u16, "Sens Item"=w1118:u16, "Tab"=w1117:i32, "Distance Unit"=w1116:u16, "discard cycles"=w1115:dbl, "Weigting"=w1114:string, "Averaging Time"=w1113:dbl, "Max duration"=w1112:dbl, "Min duration"=w1111:dbl, "Attack Threshold"=w1110:dbl, "Hysteresis Up"=w1109:dbl, "Fmin(Hz)"=w1108:dbl, "Fmax(Hz)"=w1107:dbl, "Freq.Resolution"=w1106:dbl, "Over-samples Res."=w1105:dbl, "Win Resolution"=w1104:dbl, "distance"=w1103:dbl, "samples"=w1102:dbl, "Overlap"=w1101:dbl, "Record Length"=w1100:dbl, "No.of FFTs"=w1099:dbl, "Hz"=w1098:dbl, "record delay"=w1097:dbl, "Std Err"=w1096:dbl, "Response"=w1095:bool, "Coherent Power*"=w1094:bool, "Stimulus"=w1093:bool, "Measurement Confidence"=w1092:bool, "Auto Spectrum(Response)*"=w1091:bool, "Auto Spectrum(Stimulus)*"=w1090:bool, "Cross Spectrum*"=w1089:bool, "functions"=w1088:bool, "Frequency Response"=w1087:bool, "Non-Coherent Power*"=w1086:bool, "Coherence (%)"=w1085:bool, "Non-Coherence (%)"=w1084:bool, "Signal-Noise Ratio (dB)"=w1083:bool, "Non-Coherenct Distirtion*"=w1082:bool, "Result Waveforms"=w1081:bool, "Coupling"=w1080:bool, "Averaging"=w1079:u16, "Harmonics"=w1061:i32, "Custom Curve Names"=w1060:i32, "unLabel"=w1078:string, "Custom Curve Names"=w1059:string, "Unit"=w1077:string, "Total IMD + Noise(%)"=w1076:bool, "ResponseMe"=w1075:u16, "Intermod"=w1074:dbl[], "Diff"=w1073:dbl[], "Cross-Correlation"=w1072:bool, "IM list items"=w1071:string[], "Diff list items"=w1070:string[], "TSR Window Type"=w1069:string, "Help"=w1068:string, "Custom Curve IDs"=w1067:i32[], "Default Curve Names"=w1066:string[], "Loose Particle waveform"=w1065:bool, "Imp Auto Mode"=w1063:u16)
              n71 = Bundle By Name(cluster=w1056, "Name"=w1173, "Harmonics"=w1172, "Algorithm"=w1171, "delay"=w1170, "THD(%)"=w1169, "Rub&Buzz"=w1168, "Imp"=w1167, "Imp Ref resistor"=w1166, "Y data"=w1165, "Y prefix"=w1164, "Y unit"=w1163, "Y dB ref"=w1162, "Custom Curve Names"=w1161, "har list items"=w1160, "Envelope"=w1159, "Envelope"=w1158, "use custom unit"=w1157, "autodelay ch"=w1156, "impulse"=w1155, "start ms"=w1154, "stop ms"=w1153, "Scaling"=w1152, "Default Overlap"=w1151, "Advanced View"=w1150, "Loose Particle"=w1149, "Use default"=w1148, "Auto-Correlation(Stimulus)"=w1147, "Auto-Correlation(Response)"=w1146, "Deconvolved Response"=w1145, "Mic Current"=w1064, "M List Vaiues"=w1144, "Type"=w1143, "Delay Method"=w1142, "Apply Correction Out"=w1141, "Apply Correction In"=w1140, "Harmonics @ meas.frq"=w1139, "THD Normalized(%)"=w1138, "Total Distortion"=w1137, "THD+Noise(%)"=w1136, "Rub&Buzz Norm'd(%)"=w1135, "Standard Error"=w1134, "Confidence Limits"=w1133, "Total Diff"=w1132, "Total Noise"=w1131, "Total DFD(%)"=w1130, "Total IMD(%)"=w1129, "Total IM"=w1128, "Total DFD+Noise(%)"=w1127, "Use Channel Name"=w1126, "Waveform In"=w1125, "Waveform Out"=w1124, "Method"=w1123, "Spectral Scaling"=w1122, "Appliied Unit"=w1121, "Length Unit"=w1120, "Applied Units"=w1119, "Sens Item"=w1118, "Tab"=w1117, "Distance Unit"=w1116, "discard cycles"=w1115, "Weigting"=w1114, "Averaging Time"=w1113, "Max duration"=w1112, "Min duration"=w1111, "Attack Threshold"=w1110, "Hysteresis Up"=w1109, "Fmin(Hz)"=w1108, "Fmax(Hz)"=w1107, "Freq.Resolution"=w1106, "Over-samples Res."=w1105, "Win Resolution"=w1104, "distance"=w1103, "samples"=w1102, "Overlap"=w1101, "Record Length"=w1100, "No.of FFTs"=w1099, "Hz"=w1098, "record delay"=w1097, "Std Err"=w1096, "Response"=w1095, "Coherent Power*"=w1094, "Stimulus"=w1093, "Measurement Confidence"=w1092, "Auto Spectrum(Response)*"=w1091, "Auto Spectrum(Stimulus)*"=w1090, "Cross Spectrum*"=w1089, "functions"=w1088, "Frequency Response"=w1087, "Non-Coherent Power*"=w1086, "Coherence (%)"=w1085, "Non-Coherence (%)"=w1084, "Signal-Noise Ratio (dB)"=w1083, "Non-Coherenct Distirtion*"=w1082, "Result Waveforms"=w1081, "Coupling"=w1080, "Averaging"=w1079, "Harmonics"=w1061, "Custom Curve Names"=w1060, "unLabel"=w1078, "Custom Curve Names"=w1059, "Unit"=w1077, "Total IMD + Noise(%)"=w1076, "ResponseMe"=w1075, "Intermod"=w1074, "Diff"=w1073, "Cross-Correlation"=w1072, "IM list items"=w1071, "Diff list items"=w1070, "TSR Window Type"=w1069, "Help"=w1068, "Custom Curve IDs"=w1067, "Default Curve Names"=w1066, "Loose Particle waveform"=w1065, "Imp Auto Mode"=w1063, "Mic Auto Mode"=u16 0, "Curve Resolution"=u16 2, "Curve Resolution Hz"=10.0, "Polarity"=FALSE) -> (w1174:T3)
            }
            frame 10, Default {
              n72 = Unflatten From String(type=w1180, binary string=w1184) -> (value=w1181:T3, error out=w1182:errorcluster)  [unwired: 1 in, 3 out]
              n73 = Unbundle(w1182) -> ("status"=w1183:bool)  [unwired: 2 out]
              n74 = case shown="True" w1183 {
                tunnel: w1183 -> [_ w1185]
                frame False {
                }
                frame True {
                  n75 = local write "Error?"(w1185) -> ()
                }
              }
            }
          }
        }
      }
    }
    frame True {
      n76 = local write "Error?"(TRUE ("Error?")) -> ()
    }
  }
  "Analysis" <- w1
  n77 = Bundle("substring"=w14, w15, "unsigned byte array[2]"=w16) -> (→"Header info":T14)  [unwired: 1 out]
